vi "S16EPMS.vi"() -> ()   [LabVIEW 2019]
uses:
  sub_vi-s/Global/Global Variables/System Monitor Cluster.ctl
  sub_vi-s/Monitors/Utility/Monitor Communication/Gustav/20TVTI_Cluster.ctl
  sub_vi-s/Monitors/Utility/Monitor Communication/JT/JT-Cluster.ctl
  sub_vi-s/Monitors/Utility/Monitor Communication/S16/VTI-cluster.ctl
  sub_vi-s/Monitors/Utility/Monitor Communication/S16/16T-Cluster.ctl
  sub_vi-s/Monitors/Utility/Monitor Communication/SR830/SR830-Cluster.ctl
  sub_vi-s/Monitors/Utility/Monitor Communication/S16/ILM-Cluster.ctl
  sub_vi-s/Monitors/Utility/Status Monitor/Plot.ctl
  sub_vi-s/Monitors/Utility/Monitor Communication/Gustav/20T_Dewar_Cluster.ctl
  sub_vi-s/Monitors/Utility/Monitor Communication/K6221/K6221_Cluster.ctl
  sub_vi-s/Monitors/Utility/Monitor Communication/PE7265/PE7265-Cluster.ctl
  sub_vi-s/Monitors/Utility/Monitor Communication/PicowattAVS47/PicowattAVS47-Cluster.ctl
  sub_vi-s/Monitors/Utility/Monitor Communication/Mischer/Mischer_Levelmeter-Cluster.ctl
  sub_vi-s/Monitors/Utility/Monitor Communication/Mischer/5T-Cluster.ctl
  sub_vi-s/Monitors/Utility/Monitor Communication/Mischer/Mischer-Cluster.ctl
  sub_vi-s/Monitors/Utility/Monitor Communication/Mischer/VCM-Cluster.ctl
  sub_vi-s/Monitors/Utility/LS372/LS372-Cluster.ctl
  sub_vi-s/Monitors/Utility/Monitor Communication/AMI/AMI_cluster.ctl
  sub_vi-s/Monitors/Utility/Monitor Communication/AMI/AMI_Control.ctl
  sub_vi-s/Monitors/Utility/Monitor Communication/AH2500/AH2500-Cluster.ctl
  sub_vi-s/Monitors/Utility/Monitor Communication/AH2700/AH2700-Cluster.ctl
  sub_vi-s/Monitors/Utility/Monitor Communication/Berta/15T-Cluster.ctl
  sub_vi-s/Monitors/Utility/Monitor Communication/Gustav/20TILM_Cluster.ctl
  sub_vi-s/Monitors/Utility/LS370/Monitor/LS370_only_readout_cluster.ctl
  sub_vi-s/Monitors/Utility/LS372/LS372_read_only-Cluster.ctl
  sub_vi-s/Monitors/Utility/Monitor Communication/LS370/LS370-Control.ctl
  sub_vi-s/Monitors/Utility/ITC503/ITC503Monitor-Cluster.ctl
  sub_vi-s/Monitors/Utility/Monitor Communication/LIA7230/LIA7230-cluster.ctl
  sub_vi-s/Monitors/Utility/Monitor Communication/PPMS/P9_P14_Magnet-cluster.ctl
  sub_vi-s/Monitors/Utility/Monitor Communication/K2812A/K2812A_cluster.ctl
  sub_vi-s/Equipment/Keithley 622x/Configure/2182 -A/Low Level/Typedefs/KE2182 -- Voltage Ranges.ctl
  sub_vi-s/Monitors/Utility/Monitor Communication/Torque_TMC/TMCCluster.ctl
  sub_vi-s/Monitors/Utility/Monitor Communication/PPMS/P9P14-TCluster.ctl
  sub_vi-s/Monitors/Utility/Monitor Communication/zurich_lock_in/zurichinstMonitor.ctl
  sub_vi-s/Monitors/Utility/Monitor Communication/Gustav/20T_Cluster.ctl
  sub_vi-s/Monitors/Utility/Monitor Communication/Kelvinox/Kelvinox_Cluster.ctl
  sub_vi-s/Monitors/Utility/Monitor Communication/SIM921/SIM921_resistance_Bridge_cluster.ctl
  sub_vi-s/Monitors/Utility/Monitor Communication/S16/VTI-control.ctl
  sub_vi-s/Monitors/Utility/Monitor Communication/Gustav/20TVTI_Control.ctl
  sub_vi-s/Monitors/Utility/Monitor Communication/LS372/Ls372-Control.ctl
  sub_vi-s/Global/Global Variables/Data_Display_global.vi
  Instrument_Setup.vi
  sub_vi-s/Global/Global Variables/global.vi
  sub_vi-s/Monitors/Utility/Monitor Communication/sub-vis/ILM_Split_Cluster.vi
  sub_vi-s/Monitors/Utility/Monitor Communication/sub-vis/ILM_Open_Queue.vi
  sub_vi-s/Monitors/Utility/Monitor Communication/sub-vis/ILM_Queue_Commands.vi
  sub_vi-s/Monitors/Utility/Monitor Communication/sub-vis/ILM_Merge_Cluster.vi
  sub_vi-s/Monitors/Utility/Monitor Communication/sub-vis/20T_Open_Queue.vi
  sub_vi-s/Monitors/Utility/Monitor Communication/sub-vis/20T_Split_Cluster.vi
  sub_vi-s/Monitors/Utility/Monitor Communication/sub-vis/20T_Queue_Commands.vi
  sub_vi-s/Monitors/Utility/Monitor Communication/sub-vis/SR830_Open_Queue.vi
  sub_vi-s/Monitors/Utility/Monitor Communication/sub-vis/SR830_Manage_Monitor.vi
  sub_vi-s/Monitors/Utility/Monitor Communication/sub-vis/SR830-2_Open_Queue.vi
  sub_vi-s/Monitors/Utility/Monitor Communication/sub-vis/SR830-3_Open_Queue.vi
  sub_vi-s/Monitors/Utility/Monitor Communication/sub-vis/K6221_Manage_Monitor.vi
  sub_vi-s/Monitors/Utility/Monitor Communication/sub-vis/20TDewar_Open_Queue.vi
  sub_vi-s/Monitors/Utility/Monitor Communication/sub-vis/20TDewar_Manage_Monitor.vi
  sub_vi-s/Monitors/Utility/Monitor Communication/sub-vis/16T_Split_Cluster.vi
  sub_vi-s/Monitors/Utility/Monitor Communication/sub-vis/16T_Open_Queue.vi
  sub_vi-s/Monitors/Utility/Monitor Communication/sub-vis/16T_Queue_Commands.vi
  sub_vi-s/Monitors/Utility/Monitor Communication/sub-vis/16T_Merge_Cluster.vi
  sub_vi-s/Monitors/Utility/Monitor Communication/sub-vis/20T_Merge_Cluster.vi
  sub_vi-s/Monitors/Utility/Monitor Communication/sub-vis/20TVTI_Split_Cluster.vi
  sub_vi-s/Monitors/Utility/Monitor Communication/sub-vis/20TVTI_Open_Queue.vi
  sub_vi-s/Monitors/Utility/Monitor Communication/sub-vis/20TVTI_Queue_Commands.vi
  sub_vi-s/Monitors/Utility/Monitor Communication/sub-vis/20TVTI_Merge_Cluster.vi
  sub_vi-s/Monitors/Utility/Monitor Communication/sub-vis/LS370_Open_Queue.vi
  sub_vi-s/Monitors/Utility/Monitor Communication/sub-vis/JT_Split_Cluster.vi
  sub_vi-s/Monitors/Utility/Monitor Communication/sub-vis/LS370_Queue_Commands.vi
  sub_vi-s/Monitors/Utility/Monitor Communication/sub-vis/JT_Set_Monitor_Values.vi
  sub_vi-s/Monitors/Utility/Monitor Communication/sub-vis/JT_Merge_Cluster.vi
  sub_vi-s/Equipment/Keithley 622x/Keithley 622x.lvlib
panel:
  in  "SIM921":T1
  in  "Kelvinox-Cluster":T2 {"Sorb" format="%_3g"; "MC Heater" format="%#.0f"; "Sorb Heater" format="%#.0f"; "Still Heater" format="%#.0f"; "Rate (K/min)" min=0.0 max=1.0 step=0.001 format="%.3g"; "Setpoint-Manual" min=0.0 max=10.0 step=0.001 format="%.3f"; "T-Setpoint" format="%.3f"; "Sample" format="%_3g"; "4K" format="%_3g"; "MC" format="%_3g"; "Cold\nPlate" format="%_3g"; "1K Pot" format="%_3g"; "Still" format="%_3g"; "P5" format="%_3f"; "P4" format="%_3f"; "P3" format="%_3f"; "P2" format="%_3f"; "P1" format="%_3g"; "Dump" scale=0.0..1000.0}
  in  "20 T Magnet control":T3={"Clamp"=FALSE, "Switch Heater"=FALSE, "Go to Zero"=FALSE, "Go to set"=FALSE, "Go to Hold"=FALSE, "Clamped"=FALSE, "Hold"=FALSE, "Set"=FALSE, "Zero"=FALSE, "Magnet (T)"=0.0, "Leads (T)"=0.0, "Magnet T (K)"=3.4572, "Switch"=FALSE, "Target Field (T)"=3.4572, "Field Setpoint (T)"=0.0, "Rate Setpoint (T/min)"=0.0, "Set Rate"=FALSE, "Rate\n(T/min) "=3.4572, "lambda NV (%)"=3.4572, "lambda p (mbar)"=3.4572, "lambda-Control"=FALSE, "Activate lambda control"=FALSE, "lambda NV  SP"=3.4572, "Set lambda NV"=FALSE, "PSU Status"="", "PSU\nVoltage"=3.4572} {"PSU\nVoltage" format="%.3f"; "lambda NV  SP" format="%.1f"; "lambda p (mbar)" format="%.1f"; "lambda NV (%)" scale=0.0..100.0; "Rate\n(T/min)" format="%.3f"; "Rate Setpoint (T/min)" format="%6.3f"; "Field Setpoint (T)" format="%6.3f"; "Target Field (T)" format="%.3f"; "Magnet T (K)" format="%4.3f"; "Leads (T)" format="%.3f"; "Magnet (T)" format="%.3g"}
  in  "Zurich-Lock-In Monitor":T4
  in  "P9-P14 T-Cluster":T5={"Setpoint"=60.0, "Rate"=10.0, "Chanel 1"=92.8406, "Approach"=0, "Set"=FALSE, "Temperature\nStatus"=6, "Autoshutdown"=FALSE} {"Temperature\nStatus" items=["TemperatureUnknown"=0, "Stable"=1, "Tracking"=2, "Near"=5, "Chasing"=6, "Filling"=7, "Standby"=10, "Disabled"=13, "ImpedanceNotFunction"=14, "TempFailure"=15]; "Approach" items=["Fast Settle", "No O'Shoot"]}
  in  "TMC-Control":T6
  in  "K2182A":T7
  in  "P9/P14-Magnet-Cluster":T9={"Magnet (Oe)"=-0.333, "Setpoint (Oe)"=0.0, "Rate (Oe/min)"=100.0, "Set Field"=FALSE, "Go to zero"=FALSE, "Set Persitant/non-pers"=FALSE, "Approach"=0, "Magnet Status"=1, "Sweeping"=FALSE, "Quenched"=FALSE, "Persitant Mode "=TRUE, "Stable"=FALSE, "Steps"=1.0, "Paused Menu"=0.0, "B Step Start Field"=0.0} {"Magnet Status" items=["MagnetUnknown"=0, "StablePersistent"=1, "WarmingSwitch"=2, "CoolingSwitch"=3, "StableDriven"=4, "Iterating"=5, "Charging"=6, "Discharging"=7, "CurrentError"=8, "MagnetFailure"=15]; "Approach" items=["Linear", "NoOvershoot", "Oscillate"]}
  in  "LIA7230-3":T10={"Lockin 1"=[], "X1-Display"=0.0, "X1 Percent"=0.0, "Y1-Display"=0.0, "X1 Percent 2"=0.0, "Unit X1"="nV", "Unit X2"="nV", "X1 Overload"=FALSE, "Y1 Overload"=FALSE, "Sensitivity Setpoint"=26, "X1"=0.0, "Y1"=0.0, "Channel 3"=0.0, "Channel 4"=0.0, "Channel 4 Percent"=0.0, "Channel 3 Percent "=0.0, "Unit Channel 3"="nV", "Unit Channel 4"="nV", "Overload channel 3"=FALSE, "Overload channel 4"=FALSE, "Offsets (ON)"=FALSE, "Sensitivity Setpoint 2"=26} {"Sensitivity Setpoint 2" items=["2 nV", "5 nV", "10 nV", "20 nV", "50 nV", "100 nV", "200 nV", "500 nV", "1 µV", "2 µV", "5 µV", "10 µV", "20 µV", "50 µV", "100 µV", "200 µV", "500 µV", "1 mV", "2 mV", "5 mV", "10 mV", "20 mV", "50 mV", "100 mV", "200 mV", "500 mV", "1 V", ""]; "Channel 3 Percent" scale=0.0..100.0; "Channel 4 Percent" scale=0.0..100.0; "Sensitivity Setpoint" items=["2 nV", "5 nV", "10 nV", "20 nV", "50 nV", "100 nV", "200 nV", "500 nV", "1 µV", "2 µV", "5 µV", "10 µV", "20 µV", "50 µV", "100 µV", "200 µV", "500 µV", "1 mV", "2 mV", "5 mV", "10 mV", "20 mV", "50 mV", "100 mV", "200 mV", "500 mV", "1 V", ""]; "X1 Percent 2" scale=0.0..100.0; "X1 Percent" scale=0.0..100.0; "X1-Display" format="%#4_5f"}
  in  "LIA7230-2":T10={"Lockin 1"=[[0.0, 0.0, 0.0, 0.0, 0.0, -1e-08, -1e-08, -1e-08, 0.0, 0.0, 0.0, 0.0, 0.0, 0.0, 0.0, 0.0, 0.0, 0.0, 0.0, 0.0, 0.0, 0.0, 0.0, 0.0, 0.0, 0.0, 0.0, 0.0, 0.0, 0.0, 0.0, 0.0, 0.0, 0.0, 0.0, 0.0, 1e-08, 7e-08, 1.3e-07, 1.5e-07, 1.4e-07, 1.4e-07, 1.4e-07, 1.5e-07, 1.7000000000000001e-07, 1.7000000000000001e-07, 1.6e-07, 1.4e-07, 1.2e-07, 1.3e-07, 1.4e-07, 1.5e-07, 1.5e-07, 1.5e-07, 1.5e-07, 1.4e-07, 1.3e-07, 1.3e-07, 1.3e-07, 1.4e-07, 1.5e-07], [0.0, 0.0, 0.0, 0.0, 0.0, 0.0, 0.0, -1e-08, 0.0, 0.0, 0.0, 0.0, 0.0, 0.0, 0.0, 0.0, 0.0, 0.0, 0.0, 0.0, 0.0, 0.0, 0.0, 0.0, 0.0, 0.0, -1e-08, 0.0, 0.0, 0.0, 0.0, 0.0, 0.0, 0.0, 0.0, 0.0, 5.699999999999999e-07, 2.88e-06, 5.84e-06, 6.8e-06, 6.4000000000000006e-06, 6.38e-06, 6.480000000000001e-06, 6.9e-06, 7.8e-06, 8.2e-06, 7.62e-06, 6.59e-06, 5.940000000000001e-06, 6.04e-06, 6.5099999999999995e-06, 6.98e-06, 7.3099999999999995e-06, 7.34e-06, 7.04e-06, 6.730000000000001e-06, 6.570000000000001e-06, 6.24e-06, 6.22e-06, 6.89e-06, 7.42e-06]], "X1-Display"=0.15, "X1 Percent"=0.15, "Y1-Display"=7.42, "X1 Percent 2"=7.42, "Unit X1"="µV", "Unit X2"="µV", "X1 Overload"=FALSE, "Y1 Overload"=FALSE, "Sensitivity Setpoint"=15, "X1"=1.5e-07, "Y1"=7.42e-06, "Channel 3"=7.42, "Channel 4"=88.81, "Channel 4 Percent"=24.669444444444444, "Channel 3 Percent "=7.42, "Unit Channel 3"="µV", "Unit Channel 4"="°", "Overload channel 3"=FALSE, "Overload channel 4"=FALSE, "Offsets (ON)"=FALSE, "Sensitivity Setpoint 2"=15} {"Sensitivity Setpoint 2" items=["2 nV", "5 nV", "10 nV", "20 nV", "50 nV", "100 nV", "200 nV", "500 nV", "1 µV", "2 µV", "5 µV", "10 µV", "20 µV", "50 µV", "100 µV", "200 µV", "500 µV", "1 mV", "2 mV", "5 mV", "10 mV", "20 mV", "50 mV", "100 mV", "200 mV", "500 mV", "1 V", ""]; "Channel 3 Percent" scale=0.0..100.0; "Channel 4 Percent" scale=0.0..100.0; "Sensitivity Setpoint" items=["1 nV", "2 nV", "5 nV", "10 nV", "20 nV", "50 nV", "100 nV", "200 nV", "500 nV", "1 µV", "2 µV", "5 µV", "10 µV", "20 µV", "50 µV", "100 µV", "200 µV", "500 µV", "1 mV", "2 mV", "5 mV", "10 mV", "20 mV", "50 mV", "100 mV", "200 mV", "500 mV", "1 V"]; "X1 Percent 2" scale=0.0..100.0; "X1 Percent" scale=0.0..100.0; "X1-Display" format="%#4_6f"}
  in  "LIA7230-1":T10={"Lockin 1"=[[2e-06, 7e-06, 8.999999999999999e-06, 6e-06, 1e-06, -5e-06, -8.999999999999999e-06, -8.999999999999999e-06, -5e-06, 1e-06, 7e-06, 1e-05, 8.999999999999999e-06, 3e-06, -3e-06, -8e-06, -1e-05, -7e-06, -1e-06, 5e-06, 8.999999999999999e-06, 8e-06, 4e-06, -2e-06, -8e-06, -1e-05, -8e-06, -3e-06, 3e-06, 8e-06, 8.999999999999999e-06, 6e-06, 0.0, -6e-06, -1e-05, -8.999999999999999e-06, -3e-06, 0.0, -2e-06, -1e-06, 3e-06, 1e-06, -5e-06, -1e-05, -1.1e-05, -7e-06, 0.0, 6e-06, 8.999999999999999e-06, 7e-06, 3e-06, -3e-06, -8e-06, -1e-05, -7e-06, -2e-06, 4e-06, 8.999999999999999e-06, 8.999999999999999e-06, 5e-06, -1e-06], [-8.999999999999999e-06, -6e-06, 0.0, 6e-06, 8.999999999999999e-06, 8.999999999999999e-06, 4e-06, -3e-06, -8e-06, -1e-05, -7e-06, -1e-06, 5e-06, 8.999999999999999e-06, 8e-06, 4e-06, -1e-06, -7e-06, -1e-05, -8e-06, -3e-06, 3e-06, 8e-06, 1e-05, 6e-06, 0.0, -6e-06, -1e-05, -1e-05, -5e-06, 1e-06, 7e-06, 1e-05, 8e-06, 2e-06, -4e-06, -1.4e-05, -1.7999999999999997e-05, -6e-06, 2e-06, 5e-06, 8e-06, 8e-06, 4e-06, -3e-06, -8.999999999999999e-06, -1.1e-05, -8e-06, -2e-06, 3e-06, 7e-06, 8e-06, 5e-06, -1e-06, -7e-06, -1e-05, -8e-06, -4e-06, 2e-06, 8e-06, 1e-05]], "X1-Display"=-0.001, "X1 Percent"=0.01, "Y1-Display"=0.01, "X1 Percent 2"=0.1, "Unit X1"="mV", "Unit X2"="mV", "X1 Overload"=FALSE, "Y1 Overload"=FALSE, "Sensitivity Setpoint"=21, "X1"=-1e-06, "Y1"=1e-05, "Channel 3"=0.01, "Channel 4"=95.71, "Channel 4 Percent"=26.58611111111111, "Channel 3 Percent "=0.1, "Unit Channel 3"="mV", "Unit Channel 4"="°", "Overload channel 3"=FALSE, "Overload channel 4"=FALSE, "Offsets (ON)"=FALSE, "Sensitivity Setpoint 2"=21} {"Sensitivity Setpoint 2" items=["2 nV", "5 nV", "10 nV", "20 nV", "50 nV", "100 nV", "200 nV", "500 nV", "1 µV", "2 µV", "5 µV", "10 µV", "20 µV", "50 µV", "100 µV", "200 µV", "500 µV", "1 mV", "2 mV", "5 mV", "10 mV", "20 mV", "50 mV", "100 mV", "200 mV", "500 mV", "1 V", ""]; "Channel 3 Percent" scale=0.0..100.0; "Channel 4 Percent" scale=0.0..100.0; "Sensitivity Setpoint" items=["1 nV", "2 nV", "5 nV", "10 nV", "20 nV", "50 nV", "100 nV", "200 nV", "500 nV", "1 µV", "2 µV", "5 µV", "10 µV", "20 µV", "50 µV", "100 µV", "200 µV", "500 µV", "1 mV", "2 mV", "5 mV", "10 mV", "20 mV", "50 mV", "100 mV", "200 mV", "500 mV", "1 V"]; "X1 Percent 2" scale=0.0..100.0; "X1 Percent" scale=0.0..100.0; "X1-Display" format="%#4_6f"}
  in  "ITC503-Monitor":T11={"Temperatur (K)"=0.0, "Setpoint (K)"=0.0, "Rate (K/min)"=3.4572, "Heater (%)"=0.0, "NV (%)"=0.0, "Heater Manual"=FALSE, "NV Manual"=FALSE, "Go to Set"=FALSE, "Heater SP"=0.0, "Valid?"=FALSE, "Set Heater SP"=FALSE, "Set NV SP"=FALSE, "Heater (%) Display"=3.4572, "NV (%) Display"=3.4572, "NV Setpoint"=0.0, "Change Heater Status"=FALSE, "Change NV Status"=FALSE, "Sample 3"=0.0, "Sample 2"=0.0, "Sweep-State"=FALSE, "Set Auto PID"=FALSE, "Auto PID"=FALSE, "Stopp"=FALSE, "Setpoint-Sweep"=0.0, "Sample 1"=0.0, "Control Channel"=FALSE, "Channel 1"=FALSE, "Channel 2"=FALSE, "Channel 3"=FALSE} {"NV (%) Display" format="%4_5f"; "Heater (%) Display" format="%4_5f"; "NV (%)" scale=0.0..100.0; "Heater (%)" scale=0.0..100.0; "Rate (K/min)" format="%#4_5f"; "Setpoint (K)" format="%6_5f"}
  in  "LS370-Control":T12
  in  "LS372_Readout-Monitor":T13
  in  "LS370_Readout-Monitor":T14
  in  "20TILM":T15 {"Helium" format="%.2f"}
  in  "15T-Cluster":T16={"Magnet (T)"=0.0, "Leads (T)"=0.0, "Setpoint (T)"=3.4572, "Rate (T/min)"=0.0, "Set"=FALSE, "Zero"=FALSE, "Hold"=FALSE, "Go to zero"=FALSE, "Go to Hold"=FALSE, "Go to Set"=FALSE, "Clamp"=FALSE, "Switch Heater"=FALSE, "Rate limit"=FALSE, "Switch"=FALSE, "Clamped"=FALSE, "Persistent"=FALSE, "Quenched"=FALSE, "Sweeping"=FALSE, "Select"=FALSE} {"Rate (T/min)" format="%6_5f"; "Setpoint (T)" format="%6_5f"}
  in  "AH 2700 Monitor":T17={"Units Display"=1, "Sample Switch"=0, "Frequency"=0.0, "V excitation"=0.0, "Capacity Graphic"=[], "Loss Graphic"=[], "Capacity"=0.0, "Loss"=0.0, "Update AH2500"=FALSE, "Bias "=0.0, " AVerage"=0.0} {"V excitation" format="%#_6f"; "Units Display" items=["nanosiemens"=1, "dissipation factor"=2, "kilohms"=3, "gigohms"=4, "loss vector (jpF)"=5]}
  in  "AH2500 Monitor":T18={"Capacity Graphic"=[], "Loss Graphic"=[], "Update AH2500"=FALSE, "Capacity"=0.0, "Loss"=0.0, "AVerage"=enum."5", "ALternate"=enum."1", "BIas"=enum."Disabled", "V excitation"=enum."15.00"}
  out "AMI Status":T19
  in  "AMI_Cluster":T20={"Y Axis Status"=enum."RAMPING", "Z Axis Status"=enum."RAMPING", "Y-Axis (T)"=0.0, "Y-Axis Setpoint (T)"=0.0, "Y-Axis Rate (T/min)"=0.0, "Z-Axis (T)"=0.0, "Z-Axis Setpoint (T)"=0.0, "Z-Axis Rate (T/min)"=0.0, "B AMI rate (T)"=0.0, "AMI Monitor"=FALSE, "AMI Set field rates"=FALSE, "AMI Set field"=FALSE, "Switch Heater Y"=FALSE, "Switch Heater Z"=FALSE, "Switch Heater"=FALSE, "B AMI (T)"=0.0, "B AMI Setpoint (T)"=0.0, "Phi AMI (Deg) "=0.0, "Phi AMI Setpoint (Deg) "=0.0}
  in  "LS372-Cluster":T21={"Activate Tsweep"=FALSE, "Setpoint - Manual"=1.5, "Rate (K/min)"=0.05, "Update Lakeshores"=FALSE, "Still Heater"=FALSE, "Still Power (mW)"=0.0, "Manual Heater"=FALSE, "Manual Heater  (mW) "=0.0, "Heater Range"=0.0, "P (Gain)"=15.0, "I (Reset)"=80.0, "D (Rate)"=0.0, "Heater Power (mW)"=8.96, "MC Thermometer"=1, "MC Temperature"=1.49981, "LS372-T1"=3.18065, "LS372 -T2"=1.49981, "LS372-R1 "=779.91, "LS372-R2"=1745.45, "LS372-T3"=0.0, "LS372-T4"=0.0, "LS372-R3 "=0.0, "LS372-R4 \n\n\n\n"=0.0, "LS372-T5"=0.0, "LS372-T6"=0.0, "LS372-R5"=0.0, "LS372-R6 "=0.0, "Still Power ist"=0.0, "Set Temperatur Sweep main"=FALSE, "Setpoint ist"=1.5, "Disable Heater"=FALSE} {"MC Thermometer" items=["Speer 9905", "ROX U02453"]}
  in  "VCM Monitor":T22={"Steps"=50.0, "Amplitude SET"=1.5, "Frequenz"=19.0, "Amplitude IST"=0.0, "Frequenz IST"=0.0, "A max"=2.0, "iter"=0.0, "Update VCM"=FALSE}
  in  "Mischer Monitor":T23={"G4"=113.66, "G1"=805.0, "P2"=0.14926999999999999, "G3"=75.66, "Flow"=44.93228311689066, "Pot-Preas."=5.14, "IVC"=4.9729999999999996e-08, "G1 [mbar]"=TRUE, "G3 [mbar]"=TRUE, "G4 [mbar]"=TRUE, "IVC [mbar]"=TRUE, "P2 [mbar] "=TRUE, "Flow corrected"=149.3228311689066, "Pot-Pess. Cor"=3.661772246011217, "Pot Temp"=1.4493767123529135, "Pot [mbar]"=TRUE, "Plot"=array6x29267[175602 elements]}
  in  "5 T Cluster":T24={"Go to set"=FALSE, "Go to Zero"=FALSE, "Clamp"=FALSE, "Go to Hold"=FALSE, "Clamped "=FALSE, "Quenched 2"=FALSE, "Rate limit 2"=FALSE, "Magnet (T)"=0.0, "Leads (T)"=0.0, "Rate (T/min)"=0.2, "Sweeping"=FALSE, "Setpoint"=0.0, "Set"=FALSE, "Zero"=TRUE, "Hold"=FALSE, "Clamp"=FALSE} {"Rate (T/min)" format="%6_5f"; "Leads (T)" format="%6_5f"}
  in  "Mischer Levelmeter":T25={"Plot"=array4x25953[103812 elements], "N-Shield (%)"=70.0, "He (%)"=56.71010401793704, "Coldtrap (%)"=90.0, "He - POT (%)"=101.12017967442725, "N-Shield Refill"=FALSE, "Last fill Shield"="13.08.2019    05:51", "Auto Refill Shield"=FALSE, "Trap Refill"=FALSE, "Last fill Coldtrap"="13.08.2019    05:13", "Auto Refill Trap"=FALSE, "Shield Refill"=FALSE, "Coldtrap Refill"=FALSE, "Auto Trap activatet"=TRUE, "Auto Shield Activatet"=TRUE}
  in  "Picowatt AVS47/TS530 Cluster":T26={"Control Channel (K)"=1.4876135922130311, "AVS CH 5 (Res)"=0.0, "AVS CH 6 (Res) "=0.0, "AVS CH 7 (Res) "=0.0, "Control Res."=3914.0, "Auto Excitation"=FALSE, "Auto activatet"=FALSE, "AVS Excitation"=5} caption="Picowatt AVS47/TS530" {"AVS Excitation" items=["no Exc", "3uV", "10uV", "30uV", "100uV", "300uV", "1mV", "3mV"]}
  in  "PE7265-Cluster":T27={"Lockin 1"=[[1.143e-05, 1.14e-05, 1.139e-05, 1.142e-05, 1.142e-05, 1.142e-05, 1.138e-05, 1.133e-05, 1.136e-05, 1.133e-05, 1.124e-05, 1.124e-05, 1.129e-05, 1.132e-05, 1.138e-05, 1.141e-05, 1.132e-05, 1.124e-05, 1.123e-05, 1.125e-05, 1.132e-05, 1.142e-05, 1.142e-05, 1.131e-05, 1.124e-05, 1.126e-05, 1.125e-05, 1.124e-05, 1.131e-05, 1.131e-05, 1.126e-05, 1.126e-05, 1.131e-05, 1.133e-05, 1.131e-05, 1.132e-05, 1.136e-05, 1.135e-05, 1.134e-05, 1.14e-05, 1.14e-05, 1.135e-05, 1.133e-05, 1.133e-05, 1.129e-05, 1.124e-05, 1.131e-05, 1.13e-05, 1.133e-05, 1.137e-05, 1.134e-05, 1.134e-05, 1.134e-05, 1.131e-05, 1.134e-05, 1.138e-05, 1.137e-05, 1.131e-05, 1.13e-05, 1.134e-05, 1.137e-05], [3.5e-07, 3.5e-07, 3.1e-07, 3e-07, 2.8e-07, 2.7e-07, 2.9e-07, 3.2e-07, 3.7e-07, 4.5e-07, 4.3e-07, 3.3e-07, 3e-07, 3.8e-07, 4e-07, 2.9e-07, 2.7e-07, 3.5e-07, 3.9e-07, 3.5e-07, 3e-07, 2.9e-07, 2.9e-07, 2.9e-07, 2.8e-07, 2.9e-07, 3.5e-07, 4.2e-07, 4e-07, 3.5e-07, 3.3e-07, 3e-07, 2.6e-07, 2.2e-07, 2.3e-07, 2.9e-07, 2.8e-07, 1.8e-07, 1.5e-07, 2.3e-07, 3.5e-07, 3.5e-07, 3.3e-07, 3.3e-07, 3.4e-07, 3.6e-07, 3.7e-07, 3.4e-07, 3.1e-07, 2.9e-07, 3e-07, 3.3e-07, 3.4e-07, 3.3e-07, 3.6e-07, 3.6e-07, 3e-07, 2.4e-07, 2.1e-07, 2.6e-07, 3.6e-07]], "X1-Display"=11.37, "X1 Percent"=0.1137, "Y1-Display"=0.36, "X1 Percent 2"=0.0036, "Unit X1"="µV", "Unit X1a"="100 µV", "Unit X2"="µV", "Unit X2a"="100 µV", "X1 Overload"=FALSE, "Y1 Overload"=FALSE, "Sensitivity Setpoint"=14, "X1"=1.137e-05, "Y1"=3.6e-07} {"Sensitivity Setpoint" items=["2 nV", "5 nV", "10 nV", "20 nV", "50 nV", "100 nV", "200 nV", "500 nV", "1 µV", "2 µV", "5 µV", "10 µV", "20 µV", "50 µV", "100 µV", "200 µV", "500 µV", "1 mV", "2 mV", "5 mV", "10 mV", "20 mV", "50 mV", "100 mV", "200 mV", "500 mV", "1 V", ""]; "X1 Percent 2" scale=0.0..1.0; "X1 Percent" scale=0.0..1.0; "X1-Display" format="%#4_5f"}
  in  "Control Temperature":i16(ring)=8 caption="Control Temp" items=["Time", "LI1CH1", "LI1CH2", "LI2CH1", "LI2CH2", "LI3CH1", "LI3CH2", "Field", "N_Level", "H_Level", "Heat_370", "Sorb_Heat", "Still_Heat", "Capacity", "Loss", "Magnet_Temperature", "Lam_Pressure", "Lam_NValve", "370-T1", "370-T2", "370-T3", "370-T4", "370-T5", "370-R1", "370-R2", "370-R3", "370-R4", "370-R5", "372-T1", "372-T2", "372-T3", "372-T4", "372-T5", "372-T6", "372-R1", "372-R2", "372-R3", "372-R4", "372-R5", "372-R6", "Nada", "K2440_Res", "K2440_Current", "VTI_Heater", "VTI_NValve", "LS340_Heater", "K6221_Amplitude", "K6221_Frequency", "Cond_Pressure", "Still_Pressure", "FP_Out_Pressure", "Dump_Pressure", "V1", "V2", "V4", "V5", "V9", "Forepump", "Compressor", "K6221_Offset", "BoxTemp", "By", "Bz", "Phi", "heater-recond (%)", "Dewar Pressure ", "JT-SP-Control", "350 T1", "350 T2", "350 T3", "350 T4", "350 R1", "350 R2", "350 R3", "350 R4", "Angle", "VTI CH1", "VTI CH2", "VTI CH3", "ColdTrap", "Mischer Pot", "G1 (mbar)", "G3 (mbar) ", "G4 (mbar)", "IVC (mbar)", "P2 (mbar) ", "Pot mischer (mbar)", "AVS Control Channel (K)", "AVS Control Channel (RES)", "AVS  Channel 5 (RES) ", "LI3CH3", "LI3CH4", "LI1CH3", "LI1CH4", "LI2CH3", "LI2CH4", "Volt", "Watt", "Torque Angle", "Dewar heater (W)", "PSU Voltage", "Turbopump", "372-R7", "372-T7", "SIM921 Ch1"]
  in  "Main Sample Temperature":i16(ring)=8 caption="Sample Temp" items=["Time", "LI1CH1", "LI1CH2", "LI2CH1", "LI2CH2", "LI3CH1", "LI3CH2", "Field", "N_Level", "H_Level", "Heat_370", "Sorb_Heat", "Still_Heat", "Capacity", "Loss", "Magnet_Temperature", "Lam_Pressure", "Lam_NValve", "370-T1", "370-T2", "370-T3", "370-T4", "370-T5", "370-R1", "370-R2", "370-R3", "370-R4", "370-R5", "372-T1", "372-T2", "372-T3", "372-T4", "372-T5", "372-T6", "372-R1", "372-R2", "372-R3", "372-R4", "372-R5", "372-R6", "Nada", "K2440_Res", "K2440_Current", "VTI_Heater", "VTI_NValve", "LS340_Heater", "K6221_Amplitude", "K6221_Frequency", "Cond_Pressure", "Still_Pressure", "FP_Out_Pressure", "Dump_Pressure", "V1", "V2", "V4", "V5", "V9", "Forepump", "Compressor", "K6221_Offset", "BoxTemp", "By", "Bz", "Phi", "heater-recond (%)", "Dewar Pressure ", "JT-SP-Control", "350 T1", "350 T2", "350 T3", "350 T4", "350 R1", "350 R2", "350 R3", "350 R4", "Angle", "VTI CH1", "VTI CH2", "VTI CH3", "ColdTrap", "Mischer Pot", "G1 (mbar)", "G3 (mbar) ", "G4 (mbar)", "IVC (mbar)", "P2 (mbar) ", "Pot mischer (mbar)", "AVS Control Channel (K)", "AVS Control Channel (RES)", "AVS  Channel 5 (RES) ", "LI3CH3", "LI3CH4", "LI1CH3", "LI1CH4", "LI2CH3", "LI2CH4", "Volt", "Watt", "Torque Angle", "Dewar heater (W)", "PSU Voltage", "Turbopump", "372-R7", "372-T7", "SIM921 Ch1"]
  in  "K6221":T28={"Plot Window"=[], "A"=0.00707, "A (RMS)"=0.004999244934600001, "Hz"=22.08, "I (A)"=0.00707, "f (Hz)"=22.08, "Update"=FALSE, "Offset"=0.0, "Offset (A)"=0.0, "Compliance"=FALSE, "Output"=FALSE, "Output Status"=TRUE}
  out "Data #":dbl=44.0 format="%#_13g"
  out "Runtime":dbl=0.2294750213623047 format="%#_13g"
  in  "SR830-3":T29={"Lockin 1"=[], "X1-Display"=0.0, "Y1-Display"=0.0, "X1 Percent"=0.0, "X1 Overload"=FALSE, "Y1 Overload"=FALSE, "Unit X1"="nV", "Unit X2"="nV", "Unit X2a"="nV", "Unit X1a"="nV", "Sensitivity Setpoint"=26, "X1 Percent 2"=0.0, "Y1"=0.0, "X1"=0.0, "Preamp OVL"=FALSE} {"X1 Percent 2" scale=0.0..1.0; "Sensitivity Setpoint" items=["2 nV", "5 nV", "10 nV", "20 nV", "50 nV", "100 nV", "200 nV", "500 nV", "1 µV", "2 µV", "5 µV", "10 µV", "20 µV", "50 µV", "100 µV", "200 µV", "500 µV", "1 mV", "2 mV", "5 mV", "10 mV", "20 mV", "50 mV", "100 mV", "200 mV", "500 mV", "1 V", ""]; "X1 Percent" scale=0.0..1.0; "X1-Display" format="%#4_5f"}
  in  "20T-Dewar-Cluster":T30={"Dewar Heater (%) Bar"=0.0, "Dewar-Heater (%) Display"=3.4572, "Dewar-Heater (%) SP"=0.0, "Set Dewar-Heater SP"=FALSE, "Change D-Heater Status"=FALSE, "Dewar Pressure"=0.0, "Dewar heater manual"=FALSE, "Dewar Heater (W)"=0.0} {"Dewar Pressure" format="%4.2f"; "Dewar-Heater (%) Display" format="%4.2f"; "Dewar Heater (%) Bar" scale=0.0..100.0}
  in  "Plot 1":T31={"Measurement Graph"=[{"Y"=[3678179998.990376, 3678179999.2392263, 3678180000.2770944, 3678180001.2796392, 3678180002.2735825, 3678180003.27227, 3678180004.282026, 3678180005.268647, 3678180006.267665, 3678180007.2833424, 3678180008.273184, 3678180009.2614937, 3678180010.2721095, 3678180011.2755966, 3678180012.2743664, 3678180013.2815623, 3678180014.4197474, 3678180015.2346487, 3678180016.2441673, 3678180017.2422705, 3678180018.2973943, 3678180019.2844887, 3678180020.2784495, 3678180021.2750273, 3678180022.2797832, 3678180023.298014, 3678180024.271976, 3678180025.279363, 3678180026.2741265, 3678180027.2748265, 3678180028.281594, 3678180029.280332, 3678180030.2687154, 3678180031.2840753, 3678180032.277137, 3678180033.2809224, 3678180034.264525, 3678180035.385113, 3678180036.28983, 3678180037.285784, 3678180038.2776785, 3678180039.2631254, 3678180040.285936, 3678180041.2868166, 3678180042.264264], "X"=[-0.333, -0.333, -0.333, -0.333, -0.333, -0.333, -0.333, -0.333, -0.333, -0.333, -0.333, -0.333, -0.333, -0.333, -0.333, -0.333, -0.333, -0.333, -0.333, -0.333, -0.333, -0.333, -0.333, -0.333, -0.333, -0.333, -0.333, -0.333, -0.333, -0.333, -0.333, -0.333, -0.333, -0.333, -0.333, -0.333, -0.333, -0.333, -0.333, -0.333, -0.333, -0.333, -0.333, -0.333, -0.333]}, {"Y"=[3678179998.990376, 3678179999.2392263, 3678180000.2770944, 3678180001.2796392, 3678180002.2735825, 3678180003.27227, 3678180004.282026, 3678180005.268647, 3678180006.267665, 3678180007.2833424, 3678180008.273184, 3678180009.2614937, 3678180010.2721095, 3678180011.2755966, 3678180012.2743664, 3678180013.2815623, 3678180014.4197474, 3678180015.2346487, 3678180016.2441673, 3678180017.2422705, 3678180018.2973943, 3678180019.2844887, 3678180020.2784495, 3678180021.2750273, 3678180022.2797832, 3678180023.298014, 3678180024.271976, 3678180025.279363, 3678180026.2741265, 3678180027.2748265, 3678180028.281594, 3678180029.280332, 3678180030.2687154, 3678180031.2840753, 3678180032.277137, 3678180033.2809224, 3678180034.264525, 3678180035.385113, 3678180036.28983, 3678180037.285784, 3678180038.2776785, 3678180039.2631254, 3678180040.285936, 3678180041.2868166, 3678180042.264264], "X"=[1.5e-07, 1.5e-07, 1.5e-07, 1.5e-07, 1.5e-07, 1.5e-07, 1.5e-07, 1.5e-07, 1.5e-07, 1.5e-07, 1.5e-07, 1.5e-07, 1.5e-07, 1.5e-07, 1.5e-07, 1.5e-07, 1.5e-07, 1.5e-07, 1.5e-07, 1.5e-07, 1.5e-07, 1.5e-07, 1.5e-07, 1.5e-07, 1.5e-07, 1.5e-07, 1.5e-07, 1.5e-07, 1.5e-07, 1.5e-07, 1.5e-07, 1.5e-07, 1.5e-07, 1.5e-07, 1.5e-07, 1.5e-07, 1.5e-07, 1.5e-07, 1.5e-07, 1.5e-07, 1.5e-07, 1.5e-07, 1.5e-07, 1.5e-07, 1.5e-07]}, {"Y"=[3678179998.990376, 3678179999.2392263, 3678180000.2770944, 3678180001.2796392, 3678180002.2735825, 3678180003.27227, 3678180004.282026, 3678180005.268647, 3678180006.267665, 3678180007.2833424, 3678180008.273184, 3678180009.2614937, 3678180010.2721095, 3678180011.2755966, 3678180012.2743664, 3678180013.2815623, 3678180014.4197474, 3678180015.2346487, 3678180016.2441673, 3678180017.2422705, 3678180018.2973943, 3678180019.2844887, 3678180020.2784495, 3678180021.2750273, 3678180022.2797832, 3678180023.298014, 3678180024.271976, 3678180025.279363, 3678180026.2741265, 3678180027.2748265, 3678180028.281594, 3678180029.280332, 3678180030.2687154, 3678180031.2840753, 3678180032.277137, 3678180033.2809224, 3678180034.264525, 3678180035.385113, 3678180036.28983, 3678180037.285784, 3678180038.2776785, 3678180039.2631254, 3678180040.285936, 3678180041.2868166, 3678180042.264264], "X"=[-1e-06, -1e-06, -1e-06, -1e-06, -1e-06, -1e-06, -1e-06, -1e-06, -1e-06, -1e-06, -1e-06, -1e-06, -1e-06, -1e-06, -1e-06, -1e-06, -1e-06, -1e-06, -1e-06, -1e-06, -1e-06, -1e-06, -1e-06, -1e-06, -1e-06, -1e-06, -1e-06, -1e-06, -1e-06, -1e-06, -1e-06, -1e-06, -1e-06, -1e-06, -1e-06, -1e-06, -1e-06, -1e-06, -1e-06, -1e-06, -1e-06, -1e-06, -1e-06, -1e-06, -1e-06]}, {"Y"=[3678179998.990376, 3678179999.2392263, 3678180000.2770944, 3678180001.2796392, 3678180002.2735825, 3678180003.27227, 3678180004.282026, 3678180005.268647, 3678180006.267665, 3678180007.2833424, 3678180008.273184, 3678180009.2614937, 3678180010.2721095, 3678180011.2755966, 3678180012.2743664, 3678180013.2815623, 3678180014.4197474, 3678180015.2346487, 3678180016.2441673, 3678180017.2422705, 3678180018.2973943, 3678180019.2844887, 3678180020.2784495, 3678180021.2750273, 3678180022.2797832, 3678180023.298014, 3678180024.271976, 3678180025.279363, 3678180026.2741265, 3678180027.2748265, 3678180028.281594, 3678180029.280332, 3678180030.2687154, 3678180031.2840753, 3678180032.277137, 3678180033.2809224, 3678180034.264525, 3678180035.385113, 3678180036.28983, 3678180037.285784, 3678180038.2776785, 3678180039.2631254, 3678180040.285936, 3678180041.2868166, 3678180042.264264], "X"=[-1e-06, -1e-06, -1e-06, -1e-06, -1e-06, -1e-06, -1e-06, -1e-06, -1e-06, -1e-06, -1e-06, -1e-06, -1e-06, -1e-06, -1e-06, -1e-06, -1e-06, -1e-06, -1e-06, -1e-06, -1e-06, -1e-06, -1e-06, -1e-06, -1e-06, -1e-06, -1e-06, -1e-06, -1e-06, -1e-06, -1e-06, -1e-06, -1e-06, -1e-06, -1e-06, -1e-06, -1e-06, -1e-06, -1e-06, -1e-06, -1e-06, -1e-06, -1e-06, -1e-06, -1e-06]}], "X-Axis"=0, "Y-Axis Array"=[1, 1, 3, 7], "Scale Plot"=[], "Rescale X"=FALSE, "Rescale Y"=FALSE} {"Y-Axis Array" items=["Time", "LI1CH1", "LI1CH2", "LI2CH1", "LI2CH2", "LI3CH1", "LI3CH2", "Field", "N_Level", "H_Level", "Heat_370", "Sorb_Heat", "Still_Heat", "Capacity", "Loss", "Magnet_Temperature", "Lam_Pressure", "Lam_NValve", "370-T1", "370-T2", "370-T3", "370-T4", "370-T5", "370-R1", "370-R2", "370-R3", "370-R4", "370-R5", "372-T1", "372-T2", "372-T3", "372-T4", "372-T5", "372-T6", "372-R1", "372-R2", "372-R3", "372-R4", "372-R5", "372-R6", "Nada", "K2440_Res", "K2440_Current", "VTI_Heater", "VTI_NValve", "LS340_Heater", "K6221_Amplitude", "K6221_Frequency", "Cond_Pressure", "Still_Pressure", "FP_Out_Pressure", "Dump_Pressure", "V1", "V2", "V4", "V5", "V9", "Forepump", "Compressor", "K6221_Offset", "BoxTemp", "By", "Bz", "Phi", "heater-recond (%)", "Dewar Pressure ", "JT-SP-Control", "350 T1", "350 T2", "350 T3", "350 T4", "350 R1", "350 R2", "350 R3", "350 R4", "Angle", "VTI CH1", "VTI CH2", "VTI CH3", "ColdTrap", "Mischer Pot", "G1 (mbar)", "G3 (mbar) ", "G4 (mbar)", "IVC (mbar)", "P2 (mbar) ", "Pot mischer (mbar)", "AVS Control Channel (K)", "AVS Control Channel (RES)", "AVS  Channel 5 (RES) ", "LI3CH3", "LI3CH4", "LI1CH3", "LI1CH4", "LI2CH3", "LI2CH4", "Volt", "Watt", "Torque Angle", "Dewar heater (W)", "PSU Voltage", "Turbopump", "372-R7", "372-T7", "SIM921 Ch1"]; "X-Axis" items=["Time", "LI1CH1", "LI1CH2", "LI2CH1", "LI2CH2", "LI3CH1", "LI3CH2", "Field", "N_Level", "H_Level", "Heat_370", "Sorb_Heat", "Still_Heat", "Capacity", "Loss", "Magnet_Temperature", "Lam_Pressure", "Lam_NValve", "370-T1", "370-T2", "370-T3", "370-T4", "370-T5", "370-R1", "370-R2", "370-R3", "370-R4", "370-R5", "372-T1", "372-T2", "372-T3", "372-T4", "372-T5", "372-T6", "372-R1", "372-R2", "372-R3", "372-R4", "372-R5", "372-R6", "Nada", "K2440_Res", "K2440_Current", "VTI_Heater", "VTI_NValve", "LS340_Heater", "K6221_Amplitude", "K6221_Frequency", "Cond_Pressure", "Still_Pressure", "FP_Out_Pressure", "Dump_Pressure", "V1", "V2", "V4", "V5", "V9", "Forepump", "Compressor", "K6221_Offset", "BoxTemp", "By", "Bz", "Phi", "heater-recond (%)", "Dewar Pressure ", "JT-SP-Control", "350 T1", "350 T2", "350 T3", "350 T4", "350 R1", "350 R2", "350 R3", "350 R4", "Angle", "VTI CH1", "VTI CH2", "VTI CH3", "ColdTrap", "Mischer Pot", "G1 (mbar)", "G3 (mbar) ", "G4 (mbar)", "IVC (mbar)", "P2 (mbar) ", "Pot mischer (mbar)", "AVS Control Channel (K)", "AVS Control Channel (RES)", "AVS  Channel 5 (RES) ", "LI3CH3", "LI3CH4", "LI1CH3", "LI1CH4", "LI2CH3", "LI2CH4", "Volt", "Watt", "Torque Angle", "Dewar heater (W)", "PSU Voltage", "Turbopump", "372-R7", "372-T7", "SIM921 Ch1"]}
  in  "Plot 2":T31={"Measurement Graph"=[{"Y"=[3678179998.990376, 3678179999.2392263, 3678180000.2770944, 3678180001.2796392, 3678180002.2735825, 3678180003.27227, 3678180004.282026, 3678180005.268647, 3678180006.267665, 3678180007.2833424, 3678180008.273184, 3678180009.2614937, 3678180010.2721095, 3678180011.2755966, 3678180012.2743664, 3678180013.2815623, 3678180014.4197474, 3678180015.2346487, 3678180016.2441673, 3678180017.2422705, 3678180018.2973943, 3678180019.2844887, 3678180020.2784495, 3678180021.2750273, 3678180022.2797832, 3678180023.298014, 3678180024.271976, 3678180025.279363, 3678180026.2741265, 3678180027.2748265, 3678180028.281594, 3678180029.280332, 3678180030.2687154, 3678180031.2840753, 3678180032.277137, 3678180033.2809224, 3678180034.264525, 3678180035.385113, 3678180036.28983, 3678180037.285784, 3678180038.2776785, 3678180039.2631254, 3678180040.285936, 3678180041.2868166, 3678180042.264264], "X"=[]}, {"Y"=[3678179998.990376, 3678179999.2392263, 3678180000.2770944, 3678180001.2796392, 3678180002.2735825, 3678180003.27227, 3678180004.282026, 3678180005.268647, 3678180006.267665, 3678180007.2833424, 3678180008.273184, 3678180009.2614937, 3678180010.2721095, 3678180011.2755966, 3678180012.2743664, 3678180013.2815623, 3678180014.4197474, 3678180015.2346487, 3678180016.2441673, 3678180017.2422705, 3678180018.2973943, 3678180019.2844887, 3678180020.2784495, 3678180021.2750273, 3678180022.2797832, 3678180023.298014, 3678180024.271976, 3678180025.279363, 3678180026.2741265, 3678180027.2748265, 3678180028.281594, 3678180029.280332, 3678180030.2687154, 3678180031.2840753, 3678180032.277137, 3678180033.2809224, 3678180034.264525, 3678180035.385113, 3678180036.28983, 3678180037.285784, 3678180038.2776785, 3678180039.2631254, 3678180040.285936, 3678180041.2868166, 3678180042.264264], "X"=[1e-05, 1e-05, 1e-05, 1e-05, 1e-05, 1e-05, 1e-05, 1e-05, 1e-05, 1e-05, 1e-05, 1e-05, 1e-05, 1e-05, 1e-05, 1e-05, 1e-05, 1e-05, 1e-05, 1e-05, 1e-05, 1e-05, 1e-05, 1e-05, 1e-05, 1e-05, 1e-05, 1e-05, 1e-05, 1e-05, 1e-05, 1e-05, 1e-05, 1e-05, 1e-05, 1e-05, 1e-05, 1e-05, 1e-05, 1e-05, 1e-05, 1e-05, 1e-05, 1e-05, 1e-05]}, {"Y"=[3678179998.990376, 3678179999.2392263, 3678180000.2770944, 3678180001.2796392, 3678180002.2735825, 3678180003.27227, 3678180004.282026, 3678180005.268647, 3678180006.267665, 3678180007.2833424, 3678180008.273184, 3678180009.2614937, 3678180010.2721095, 3678180011.2755966, 3678180012.2743664, 3678180013.2815623, 3678180014.4197474, 3678180015.2346487, 3678180016.2441673, 3678180017.2422705, 3678180018.2973943, 3678180019.2844887, 3678180020.2784495, 3678180021.2750273, 3678180022.2797832, 3678180023.298014, 3678180024.271976, 3678180025.279363, 3678180026.2741265, 3678180027.2748265, 3678180028.281594, 3678180029.280332, 3678180030.2687154, 3678180031.2840753, 3678180032.277137, 3678180033.2809224, 3678180034.264525, 3678180035.385113, 3678180036.28983, 3678180037.285784, 3678180038.2776785, 3678180039.2631254, 3678180040.285936, 3678180041.2868166, 3678180042.264264], "X"=[-1e-06, -1e-06, -1e-06, -1e-06, -1e-06, -1e-06, -1e-06, -1e-06, -1e-06, -1e-06, -1e-06, -1e-06, -1e-06, -1e-06, -1e-06, -1e-06, -1e-06, -1e-06, -1e-06, -1e-06, -1e-06, -1e-06, -1e-06, -1e-06, -1e-06, -1e-06, -1e-06, -1e-06, -1e-06, -1e-06, -1e-06, -1e-06, -1e-06, -1e-06, -1e-06, -1e-06, -1e-06, -1e-06, -1e-06, -1e-06, -1e-06, -1e-06, -1e-06, -1e-06, -1e-06]}, {"Y"=[3678179998.990376, 3678179999.2392263, 3678180000.2770944, 3678180001.2796392, 3678180002.2735825, 3678180003.27227, 3678180004.282026, 3678180005.268647, 3678180006.267665, 3678180007.2833424, 3678180008.273184, 3678180009.2614937, 3678180010.2721095, 3678180011.2755966, 3678180012.2743664, 3678180013.2815623, 3678180014.4197474, 3678180015.2346487, 3678180016.2441673, 3678180017.2422705, 3678180018.2973943, 3678180019.2844887, 3678180020.2784495, 3678180021.2750273, 3678180022.2797832, 3678180023.298014, 3678180024.271976, 3678180025.279363, 3678180026.2741265, 3678180027.2748265, 3678180028.281594, 3678180029.280332, 3678180030.2687154, 3678180031.2840753, 3678180032.277137, 3678180033.2809224, 3678180034.264525, 3678180035.385113, 3678180036.28983, 3678180037.285784, 3678180038.2776785, 3678180039.2631254, 3678180040.285936, 3678180041.2868166, 3678180042.264264], "X"=[-1e-06, -1e-06, -1e-06, -1e-06, -1e-06, -1e-06, -1e-06, -1e-06, -1e-06, -1e-06, -1e-06, -1e-06, -1e-06, -1e-06, -1e-06, -1e-06, -1e-06, -1e-06, -1e-06, -1e-06, -1e-06, -1e-06, -1e-06, -1e-06, -1e-06, -1e-06, -1e-06, -1e-06, -1e-06, -1e-06, -1e-06, -1e-06, -1e-06, -1e-06, -1e-06, -1e-06, -1e-06, -1e-06, -1e-06, -1e-06, -1e-06, -1e-06, -1e-06, -1e-06, -1e-06]}], "X-Axis"=0, "Y-Axis Array"=[1, 1, 2, 82], "Scale Plot"=[], "Rescale X"=FALSE, "Rescale Y"=FALSE} {"Y-Axis Array" items=["Time", "LI1CH1", "LI1CH2", "LI2CH1", "LI2CH2", "LI3CH1", "LI3CH2", "Field", "N_Level", "H_Level", "Heat_370", "Sorb_Heat", "Still_Heat", "Capacity", "Loss", "Magnet_Temperature", "Lam_Pressure", "Lam_NValve", "370-T1", "370-T2", "370-T3", "370-T4", "370-T5", "370-R1", "370-R2", "370-R3", "370-R4", "370-R5", "372-T1", "372-T2", "372-T3", "372-T4", "372-T5", "372-T6", "372-R1", "372-R2", "372-R3", "372-R4", "372-R5", "372-R6", "Nada", "K2440_Res", "K2440_Current", "VTI_Heater", "VTI_NValve", "LS340_Heater", "K6221_Amplitude", "K6221_Frequency", "Cond_Pressure", "Still_Pressure", "FP_Out_Pressure", "Dump_Pressure", "V1", "V2", "V4", "V5", "V9", "Forepump", "Compressor", "K6221_Offset", "BoxTemp", "By", "Bz", "Phi", "heater-recond (%)", "Dewar Pressure ", "JT-SP-Control", "350 T1", "350 T2", "350 T3", "350 T4", "350 R1", "350 R2", "350 R3", "350 R4", "Angle", "VTI CH1", "VTI CH2", "VTI CH3", "ColdTrap", "Mischer Pot", "G1 (mbar)", "G3 (mbar) ", "G4 (mbar)", "IVC (mbar)", "P2 (mbar) ", "Pot mischer (mbar)", "AVS Control Channel (K)", "AVS Control Channel (RES)", "AVS  Channel 5 (RES) ", "LI3CH3", "LI3CH4", "LI1CH3", "LI1CH4", "LI2CH3", "LI2CH4", "Volt", "Watt", "Torque Angle", "Dewar heater (W)", "PSU Voltage", "Turbopump", "372-R7", "372-T7", "SIM921 Ch1"]; "X-Axis" items=["Time", "LI1CH1", "LI1CH2", "LI2CH1", "LI2CH2", "LI3CH1", "LI3CH2", "Field", "N_Level", "H_Level", "Heat_370", "Sorb_Heat", "Still_Heat", "Capacity", "Loss", "Magnet_Temperature", "Lam_Pressure", "Lam_NValve", "370-T1", "370-T2", "370-T3", "370-T4", "370-T5", "370-R1", "370-R2", "370-R3", "370-R4", "370-R5", "372-T1", "372-T2", "372-T3", "372-T4", "372-T5", "372-T6", "372-R1", "372-R2", "372-R3", "372-R4", "372-R5", "372-R6", "Nada", "K2440_Res", "K2440_Current", "VTI_Heater", "VTI_NValve", "LS340_Heater", "K6221_Amplitude", "K6221_Frequency", "Cond_Pressure", "Still_Pressure", "FP_Out_Pressure", "Dump_Pressure", "V1", "V2", "V4", "V5", "V9", "Forepump", "Compressor", "K6221_Offset", "BoxTemp", "By", "Bz", "Phi", "heater-recond (%)", "Dewar Pressure ", "JT-SP-Control", "350 T1", "350 T2", "350 T3", "350 T4", "350 R1", "350 R2", "350 R3", "350 R4", "Angle", "VTI CH1", "VTI CH2", "VTI CH3", "ColdTrap", "Mischer Pot", "G1 (mbar)", "G3 (mbar) ", "G4 (mbar)", "IVC (mbar)", "P2 (mbar) ", "Pot mischer (mbar)", "AVS Control Channel (K)", "AVS Control Channel (RES)", "AVS  Channel 5 (RES) ", "LI3CH3", "LI3CH4", "LI1CH3", "LI1CH4", "LI2CH3", "LI2CH4", "Volt", "Watt", "Torque Angle", "Dewar heater (W)", "PSU Voltage", "Turbopump", "372-R7", "372-T7", "SIM921 Ch1"]}
  in  "Plot 3":T31 {"Y-Axis Array" items=["Time", "LI1CH1", "LI1CH2", "LI2CH1", "LI2CH2", "LI3CH1", "LI3CH2", "Field", "N_Level", "H_Level", "Heat_370", "Sorb_Heat", "Still_Heat", "Capacity", "Loss", "Magnet_Temperature", "Lam_Pressure", "Lam_NValve", "370-T1", "370-T2", "370-T3", "370-T4", "370-T5", "370-R1", "370-R2", "370-R3", "370-R4", "370-R5", "372-T1", "372-T2", "372-T3", "372-T4", "372-T5", "372-T6", "372-R1", "372-R2", "372-R3", "372-R4", "372-R5", "372-R6", "Nada", "K2440_Res", "K2440_Current", "VTI_Heater", "VTI_NValve", "LS340_Heater", "K6221_Amplitude", "K6221_Frequency", "Cond_Pressure", "Still_Pressure", "FP_Out_Pressure", "Dump_Pressure", "V1", "V2", "V4", "V5", "V9", "Forepump", "Compressor", "K6221_Offset", "BoxTemp", "By", "Bz", "Phi", "heater-recond (%)", "Dewar Pressure ", "JT-SP-Control", "350 T1", "350 T2", "350 T3", "350 T4", "350 R1", "350 R2", "350 R3", "350 R4", "Angle", "VTI CH1", "VTI CH2", "VTI CH3", "ColdTrap", "Mischer Pot", "G1 (mbar)", "G3 (mbar) ", "G4 (mbar)", "IVC (mbar)", "P2 (mbar) ", "Pot mischer (mbar)", "AVS Control Channel (K)", "AVS Control Channel (RES)", "AVS  Channel 5 (RES) ", "LI3CH3", "LI3CH4", "LI1CH3", "LI1CH4", "LI2CH3", "LI2CH4", "Volt", "Watt", "Torque Angle", "Dewar heater (W)", "PSU Voltage", "Turbopump", "372-R7", "372-T7", "SIM921 Ch1"]; "X-Axis" items=["Time", "LI1CH1", "LI1CH2", "LI2CH1", "LI2CH2", "LI3CH1", "LI3CH2", "Field", "N_Level", "H_Level", "Heat_370", "Sorb_Heat", "Still_Heat", "Capacity", "Loss", "Magnet_Temperature", "Lam_Pressure", "Lam_NValve", "370-T1", "370-T2", "370-T3", "370-T4", "370-T5", "370-R1", "370-R2", "370-R3", "370-R4", "370-R5", "372-T1", "372-T2", "372-T3", "372-T4", "372-T5", "372-T6", "372-R1", "372-R2", "372-R3", "372-R4", "372-R5", "372-R6", "Nada", "K2440_Res", "K2440_Current", "VTI_Heater", "VTI_NValve", "LS340_Heater", "K6221_Amplitude", "K6221_Frequency", "Cond_Pressure", "Still_Pressure", "FP_Out_Pressure", "Dump_Pressure", "V1", "V2", "V4", "V5", "V9", "Forepump", "Compressor", "K6221_Offset", "BoxTemp", "By", "Bz", "Phi", "heater-recond (%)", "Dewar Pressure ", "JT-SP-Control", "350 T1", "350 T2", "350 T3", "350 T4", "350 R1", "350 R2", "350 R3", "350 R4", "Angle", "VTI CH1", "VTI CH2", "VTI CH3", "ColdTrap", "Mischer Pot", "G1 (mbar)", "G3 (mbar) ", "G4 (mbar)", "IVC (mbar)", "P2 (mbar) ", "Pot mischer (mbar)", "AVS Control Channel (K)", "AVS Control Channel (RES)", "AVS  Channel 5 (RES) ", "LI3CH3", "LI3CH4", "LI1CH3", "LI1CH4", "LI2CH3", "LI2CH4", "Volt", "Watt", "Torque Angle", "Dewar heater (W)", "PSU Voltage", "Turbopump", "372-R7", "372-T7", "SIM921 Ch1"]}
  in  "20TVTI":T32={"Temperatur (K)"=70.6986, "Setpoint (K)"=0.0, "Rate (K/min)"=3.4572, "Heater (%)"=0.0017142857142857142, "NV (%)"=0.0, "Heater Manual"=TRUE, "NV Manual"=TRUE, "Go to Set"=FALSE, "Pressure"=1.0208606, "Heater SP"=0.0, "Valid?"=FALSE, "Set Heater SP"=FALSE, "Set NV SP"=FALSE, "Heater (%) Display"=0.0, "NV (%) Display"=0.0, "NV Setpoint"=0.0, "Change Heater Status"=FALSE, "Change NV Status"=FALSE, "Change Sweep Type"=FALSE} {"NV (%) Display" format="%4_5f"; "Heater (%) Display" format="%4_5f"; "Heater SP" format="%#4_5f"; "Pressure" format="%#4_5f"; "NV (%)" scale=0.0..100.0; "Heater (%)" scale=0.0..100.0; "Rate (K/min)" format="%#4_5f"; "Setpoint (K)" format="%6_5f"}
  in  "ILM":T33 {"Nitrogen" format="%#4_5f"}
  out "Final rate":dbl format="%#4_5f"
  out "Init rate":dbl format="%#4_5f"
  in  "Panel 6":i16(ring) items=["empty", "SR830-1", "SR830-2", "ILM", "20TILM", "AH2700", "K6221", "Plot3", "20T-Dewar", "SR830-3", "PE7265", "MischerMonitor", "MischerLevelmeter", "LS370 Readout", "LS372 Readout", "LIA7230-1", "LIA7230-2", "LIA7230-3", "K2182A", "TMC Monitor", "zurich_Lock_in", "SIM921"]
  in  "Panel 2":i16(ring) items=["empty", "SR830-1", "SR830-2", "ILM", "20TILM", "AH2700", "K6221", "Plot3", "20T-Dewar", "SR830-3", "PE7265", "MischerMonitor", "MischerLevelmeter", "LS370 Readout", "LS372 Readout", "LIA7230-1", "LIA7230-2", "LIA7230-3", "K2182A", "TMC Monitor", "zurich_Lock_in", "SIM921"]
  in  "Panel 4":i16(ring) items=["empty", "SR830-1", "SR830-2", "ILM", "20TILM", "AH2700", "K6221", "Plot3", "20T-Dewar", "SR830-3", "PE7265", "MischerMonitor", "MischerLevelmeter", "LS370 Readout", "LS372 Readout", "LIA7230-1", "LIA7230-2", "LIA7230-3", "K2182A", "TMC Monitor", "zurich_Lock_in", "SIM921"]
  in  "Panel 5":i16(ring) items=["empty", "SR830-1", "SR830-2", "ILM", "20TILM", "AH2700", "K6221", "Plot3", "20T-Dewar", "SR830-3", "PE7265", "MischerMonitor", "MischerLevelmeter", "LS370 Readout", "LS372 Readout", "LIA7230-1", "LIA7230-2", "LIA7230-3", "K2182A", "TMC Monitor", "zurich_Lock_in", "SIM921"]
  in  "Panel 3":i16(ring)=16 items=["empty", "SR830-1", "SR830-2", "ILM", "20TILM", "AH2700", "K6221", "Plot3", "20T-Dewar", "SR830-3", "PE7265", "MischerMonitor", "MischerLevelmeter", "LS370 Readout", "LS372 Readout", "LIA7230-1", "LIA7230-2", "LIA7230-3", "K2182A", "TMC Monitor", "zurich_Lock_in", "SIM921"]
  in  "Panel 1":i16(ring)=15 items=["empty", "SR830-1", "SR830-2", "ILM", "20TILM", "AH2700", "K6221", "Plot3", "20T-Dewar", "SR830-3", "PE7265", "MischerMonitor", "MischerLevelmeter", "LS370 Readout", "LS372 Readout", "LIA7230-1", "LIA7230-2", "LIA7230-3", "K2182A", "TMC Monitor", "zurich_Lock_in", "SIM921"]
  in  "SR830-2":T29={"Lockin 1"=[], "X1-Display"=0.0, "Y1-Display"=0.0, "X1 Percent"=0.0, "X1 Overload"=FALSE, "Y1 Overload"=FALSE, "Unit X1"="nV", "Unit X2"="nV", "Unit X2a"="nV", "Unit X1a"="nV", "Sensitivity Setpoint"=22, "X1 Percent 2"=0.0, "Y1"=0.0, "X1"=0.0, "Preamp OVL"=FALSE} {"X1 Percent 2" scale=0.0..1.0; "Sensitivity Setpoint" items=["2 nV", "5 nV", "10 nV", "20 nV", "50 nV", "100 nV", "200 nV", "500 nV", "1 µV", "2 µV", "5 µV", "10 µV", "20 µV", "50 µV", "100 µV", "200 µV", "500 µV", "1 mV", "2 mV", "5 mV", "10 mV", "20 mV", "50 mV", "100 mV", "200 mV", "500 mV", "1 V", ""]; "X1 Percent" scale=0.0..1.0; "X1-Display" format="%#_5f"}
  in  "SR830-1":T29={"Lockin 1"=[[1.4931e-05, 1.4931e-05, 1.4931e-05, 1.4931e-05, 1.4931e-05, 1.4931e-05, 1.4931e-05, 1.4931e-05, 1.4931e-05, 1.4931e-05, 1.4931e-05, 1.4931e-05, 1.4931e-05, 1.4931e-05, 1.4931e-05, 1.4931e-05, 1.4931e-05, 1.4931e-05, 1.4931e-05, 1.4931e-05, 1.4931e-05, 1.4931e-05, 1.4931e-05, 1.4931e-05, 1.4931e-05, 1.4931e-05, 1.4931e-05, 1.4931e-05, 1.4931e-05, 1.4931e-05, 1.4931e-05, 1.4931e-05, 1.4931e-05, 1.4931e-05, 1.4931e-05, 1.4931e-05, 1.4931e-05, 1.4931e-05, 1.4931e-05, 1.4931e-05, 1.4931e-05, 1.4931e-05, 1.4931e-05, 1.4931e-05, 1.4931e-05, 1.4931e-05, 1.4931e-05, 1.4931e-05, 1.4931e-05, 1.4931e-05, 1.4931e-05, 1.4931e-05, 1.4931e-05, 1.4931e-05, 1.4931e-05, 1.4931e-05, 1.4931e-05, 1.4931e-05, 1.4931e-05, 1.4931e-05, 1.4931e-05], [2.11598e-06, 2.11598e-06, 2.11598e-06, 2.11598e-06, 2.11598e-06, 2.11598e-06, 2.11598e-06, 2.11598e-06, 2.11598e-06, 2.11598e-06, 2.11598e-06, 2.11598e-06, 2.11598e-06, 2.11598e-06, 2.11598e-06, 2.11598e-06, 2.11598e-06, 2.11598e-06, 2.11598e-06, 2.11598e-06, 2.11598e-06, 2.11598e-06, 2.11598e-06, 2.11598e-06, 2.11598e-06, 2.11598e-06, 2.11598e-06, 2.11598e-06, 2.11598e-06, 2.11598e-06, 2.11598e-06, 2.11598e-06, 2.11598e-06, 2.11598e-06, 2.11598e-06, 2.11598e-06, 2.11598e-06, 2.11598e-06, 2.11598e-06, 2.11598e-06, 2.11598e-06, 2.11598e-06, 2.11598e-06, 2.11598e-06, 2.11598e-06, 2.11598e-06, 2.11598e-06, 2.11598e-06, 2.11598e-06, 2.11598e-06, 2.11598e-06, 2.11598e-06, 2.11598e-06, 2.11598e-06, 2.11598e-06, 2.11598e-06, 2.11598e-06, 2.11598e-06, 2.11598e-06, 2.11598e-06, 2.11598e-06]], "X1-Display"=14.931, "Y1-Display"=2.11598, "X1 Percent"=0.029862, "X1 Overload"=FALSE, "Y1 Overload"=FALSE, "Unit X1"="µV", "Unit X2"="µV", "Unit X2a"="500 µV", "Unit X1a"="500 µV", "Sensitivity Setpoint"=16, "X1 Percent 2"=0.00423196, "Y1"=2.11598e-06, "X1"=1.4931e-05, "Preamp OVL"=FALSE} {"X1 Percent 2" scale=0.0..1.0; "Sensitivity Setpoint" items=["2 nV", "5 nV", "10 nV", "20 nV", "50 nV", "100 nV", "200 nV", "500 nV", "1 µV", "2 µV", "5 µV", "10 µV", "20 µV", "50 µV", "100 µV", "200 µV", "500 µV", "1 mV", "2 mV", "5 mV", "10 mV", "20 mV", "50 mV", "100 mV", "200 mV", "500 mV", "1 V", ""]; "X1 Percent" scale=0.0..1.0; "X1-Display" format="%-#1_5f"}
  in  "16 T Magnet control":T34={"Clamp"=FALSE, "Switch Heater"=FALSE, "Go to Zero"=FALSE, "Go to set"=FALSE, "Go to Hold"=FALSE, "Clamped"=FALSE, "Quenched"=FALSE, "Rate limit"=FALSE, "Persistent"=FALSE, "Hold"=FALSE, "Set"=FALSE, "Zero"=FALSE, "Magnet (T)"=0.0, "Leads (T)"=0.0, "Magnet T (K)"=0.0, "Switch"=FALSE, "Setpoint (T)"=0.0, "Rate (T/min)"=0.001, "Select"=FALSE, "Sweeping"=FALSE} {"Rate (T/min)" format="%#_5f"; "Setpoint (T)" format="%#_5f"; "Magnet T (K)" format="%#4_5f"; "Leads (T)" format="%#_5f"}
  in  "VTI":T35={"Temperatur (K)"=0.0, "Setpoint (K)"=0.0, "Rate (K/min)"=3.4572, "Heater (%)"=0.0, "NV (%)"=0.0, "Heater Manual"=FALSE, "NV Manual"=FALSE, "Go to Set"=FALSE, "Pressure"=0.0, "Heater SP"=0.0, "Valid?"=FALSE, "Set Heater SP"=FALSE, "Set NV SP"=FALSE, "Heater (%) Display"=3.4572, "NV (%) Display"=3.4572, "NV Setpoint"=0.0, "Change Heater Status"=FALSE, "Change NV Status"=FALSE, "Sample 3"=0.0, "Sample 2"=0.0, "Sweep-State"=FALSE, "Set Auto PID"=FALSE, "Auto PID"=FALSE, "Stopp"=FALSE, "Setpoint-Sweep"=0.0} {"NV (%) Display" format="%4_5f"; "Heater (%) Display" format="%4_5f"; "Pressure" format="%#4_5f"; "NV (%)" scale=0.0..100.0; "Heater (%)" scale=0.0..100.0; "Rate (K/min)" format="%#4_5f"; "Setpoint (K)" format="%#_5f"}
  in  "Reset Warning":bool
  in  "JT-Cluster":T36={"Setpoint - Manual"=0.0, "Rate (K/min)"=0.0, "Activate Tsweep"=FALSE, "Disable Heater"=FALSE, "Update Lakeshores"=FALSE, "Still Heater"=FALSE, "Sorb Heater"=FALSE, "Still Power (mW)"=0.0, "Sorb Power (mW)"=0.0, "V2"=FALSE, "V5"=FALSE, "V1"=FALSE, "V9"=FALSE, "F"=FALSE, "C"=FALSE, "V4"=FALSE, "Dump"=0, "P3"=0.0, "P1"=0.0, "P2"=0.0, "P5"=0.0, "Box Temp"=0.0, "Pressure 1"=0, "Pressure 2"=0, "Pressure 3"=15, "Pressure 4"=13, "Setpoint"=0.0, "MC Heater Output"=0.0, "Still Heater Output"=0.0, "Sorb  Heater Output"=0.0, "Heater"=[], "Pressures"=[]} {"Pressure 4" items=["Time", "LI1CH1", "LI1CH2", "LI2CH1", "LI2CH2", "LI3CH1", "LI3CH2", "Field", "Temperature", "Temperature 2", "Temperatrue 3", "Nitrogen_Level", "Helium_Level", "Heater_LS370", "Sorb_Heater", "Still_Heater", "Capacity", "Loss", "Magnet_Temperature", "Lambda_Pressure", "Lambda_Needle_Valve", "LS370-CH1-T", "LS370-CH2-T", "LS370-CH3-T", "LS370-CH4-T", "LS370-TC-T", "LS370-CH1-R", "LS370-CH2-R", "LS370-CH3-R", "LS370-CH4-R", "LS370-TC-R", "LS372-CH1-T", "LS372-CH2-T", "LS372-CH3-T", "LS372-CH4-T", "LS372-CH5-T", "LS372-CH1-R", "LS372-CH2-R", "LS372-CH3-R", "LS372-CH4-R", "LS372-CH5-R", "Nada", "Keithley_Res", "Keithley_Current", "VTI_Heater", "VTI_Needle Valve", "LS340_Heater", "Keithley_6221_Amplitude", "Keithley_6221_Frequency", "Condense_Pressure", "Still_Pressure", "FP_Out_Pressure", "Dump_Pressure", "V1", "V2", "V4", "V5", "V9", "Forepump", "Compressor", "Keihtley_6221_Offset", "BoxTemp", "By", "Bz", "Phi", "heater-recond (%)", "Dewar Pressure "]; "Pressure 3" items=["Time", "LI1CH1", "LI1CH2", "LI2CH1", "LI2CH2", "LI3CH1", "LI3CH2", "Field", "Temperature", "Temperature 2", "Temperatrue 3", "Nitrogen_Level", "Helium_Level", "Heater_LS370", "Sorb_Heater", "Still_Heater", "Capacity", "Loss", "Magnet_Temperature", "Lambda_Pressure", "Lambda_Needle_Valve", "LS370-CH1-T", "LS370-CH2-T", "LS370-CH3-T", "LS370-CH4-T", "LS370-TC-T", "LS370-CH1-R", "LS370-CH2-R", "LS370-CH3-R", "LS370-CH4-R", "LS370-TC-R", "LS372-CH1-T", "LS372-CH2-T", "LS372-CH3-T", "LS372-CH4-T", "LS372-CH5-T", "LS372-CH1-R", "LS372-CH2-R", "LS372-CH3-R", "LS372-CH4-R", "LS372-CH5-R", "Nada", "Keithley_Res", "Keithley_Current", "VTI_Heater", "VTI_Needle Valve", "LS340_Heater", "Keithley_6221_Amplitude", "Keithley_6221_Frequency", "Condense_Pressure", "Still_Pressure", "FP_Out_Pressure", "Dump_Pressure", "V1", "V2", "V4", "V5", "V9", "Forepump", "Compressor", "Keihtley_6221_Offset", "BoxTemp", "By", "Bz", "Phi", "heater-recond (%)", "Dewar Pressure "]; "Pressure 2" items=["Time", "LI1CH1", "LI1CH2", "LI2CH1", "LI2CH2", "LI3CH1", "LI3CH2", "Field", "Temperature", "Temperature 2", "Temperatrue 3", "Nitrogen_Level", "Helium_Level", "Heater_LS370", "Sorb_Heater", "Still_Heater", "Capacity", "Loss", "Magnet_Temperature", "Lambda_Pressure", "Lambda_Needle_Valve", "LS370-CH1-T", "LS370-CH2-T", "LS370-CH3-T", "LS370-CH4-T", "LS370-TC-T", "LS370-CH1-R", "LS370-CH2-R", "LS370-CH3-R", "LS370-CH4-R", "LS370-TC-R", "LS372-CH1-T", "LS372-CH2-T", "LS372-CH3-T", "LS372-CH4-T", "LS372-CH5-T", "LS372-CH1-R", "LS372-CH2-R", "LS372-CH3-R", "LS372-CH4-R", "LS372-CH5-R", "Nada", "Keithley_Res", "Keithley_Current", "VTI_Heater", "VTI_Needle Valve", "LS340_Heater", "Keithley_6221_Amplitude", "Keithley_6221_Frequency", "Condense_Pressure", "Still_Pressure", "FP_Out_Pressure", "Dump_Pressure", "V1", "V2", "V4", "V5", "V9", "Forepump", "Compressor", "Keihtley_6221_Offset", "BoxTemp", "By", "Bz", "Phi", "heater-recond (%)", "Dewar Pressure "]; "Pressure 1" items=["Time", "LI1CH1", "LI1CH2", "LI2CH1", "LI2CH2", "LI3CH1", "LI3CH2", "Field", "Temperature", "Temperature 2", "Temperatrue 3", "Nitrogen_Level", "Helium_Level", "Heater_LS370", "Sorb_Heater", "Still_Heater", "Capacity", "Loss", "Magnet_Temperature", "Lambda_Pressure", "Lambda_Needle_Valve", "LS370-CH1-T", "LS370-CH2-T", "LS370-CH3-T", "LS370-CH4-T", "LS370-TC-T", "LS370-CH1-R", "LS370-CH2-R", "LS370-CH3-R", "LS370-CH4-R", "LS370-TC-R", "LS372-CH1-T", "LS372-CH2-T", "LS372-CH3-T", "LS372-CH4-T", "LS372-CH5-T", "LS372-CH1-R", "LS372-CH2-R", "LS372-CH3-R", "LS372-CH4-R", "LS372-CH5-R", "Nada", "Keithley_Res", "Keithley_Current", "VTI_Heater", "VTI_Needle Valve", "LS340_Heater", "Keithley_6221_Amplitude", "Keithley_6221_Frequency", "Condense_Pressure", "Still_Pressure", "FP_Out_Pressure", "Dump_Pressure", "V1", "V2", "V4", "V5", "V9", "Forepump", "Compressor", "Keihtley_6221_Offset", "BoxTemp", "By", "Bz", "Phi", "heater-recond (%)", "Dewar Pressure "]; "Dump" scale=0.0..540.0}
  in  "Open":bool
  in  "Save":bool
  out "Emergency Stop JT":string
  out "Phi (Deg)":dbl format="%#4_5f"
  out "Step #":dbl format="%#4_5f"
  in  "Truncate Button 2":bool
  in  "Time Stamp":timestamp
  in  "Truncate Button":bool
  in  "Keep every nth":i32=2 min=1 max=10 step=1
  in  "Readout \nMeas (s)":dbl=1.0 format="%#_13g"
  in  "Readout\nMonitor (s)":dbl=1.0 format="%#_13g"
  in  "E-mail of Experiment resposible":string
  out "Warning-Bool":bool
  out "Warning":string
  in  "Temperature 6":i16(ring)=41 items=["Time", "LI1CH1", "LI1CH2", "LI2CH1", "LI2CH2", "LI3CH1", "LI3CH2", "Field", "N_Level", "H_Level", "Heat_370", "Sorb_Heat", "Still_Heat", "Capacity", "Loss", "Magnet_Temperature", "Lam_Pressure", "Lam_NValve", "370-T1", "370-T2", "370-T3", "370-T4", "370-T5", "370-R1", "370-R2", "370-R3", "370-R4", "370-R5", "372-T1", "372-T2", "372-T3", "372-T4", "372-T5", "372-T6", "372-R1", "372-R2", "372-R3", "372-R4", "372-R5", "372-R6", "Nada", "K2440_Res", "K2440_Current", "VTI_Heater", "VTI_NValve", "LS340_Heater", "K6221_Amplitude", "K6221_Frequency", "Cond_Pressure", "Still_Pressure", "FP_Out_Pressure", "Dump_Pressure", "V1", "V2", "V4", "V5", "V9", "Forepump", "Compressor", "K6221_Offset", "BoxTemp", "By", "Bz", "Phi", "heater-recond (%)", "Dewar Pressure ", "JT-SP-Control", "350 T1", "350 T2", "350 T3", "350 T4", "350 R1", "350 R2", "350 R3", "350 R4", "Angle", "VTI CH1", "VTI CH2", "VTI CH3", "ColdTrap", "Mischer Pot", "G1 (mbar)", "G3 (mbar) ", "G4 (mbar)", "IVC (mbar)", "P2 (mbar) ", "Pot mischer (mbar)", "AVS Control Channel (K)", "AVS Control Channel (RES)", "AVS  Channel 5 (RES) ", "LI3CH3", "LI3CH4", "LI1CH3", "LI1CH4", "LI2CH3", "LI2CH4", "Volt", "Watt", "Torque Angle", "Dewar heater (W)", "PSU Voltage", "Turbopump", "372-R7", "372-T7", "SIM921 Ch1"]
  in  "Temperature 5":i16(ring)=41 items=["Time", "LI1CH1", "LI1CH2", "LI2CH1", "LI2CH2", "LI3CH1", "LI3CH2", "Field", "N_Level", "H_Level", "Heat_370", "Sorb_Heat", "Still_Heat", "Capacity", "Loss", "Magnet_Temperature", "Lam_Pressure", "Lam_NValve", "370-T1", "370-T2", "370-T3", "370-T4", "370-T5", "370-R1", "370-R2", "370-R3", "370-R4", "370-R5", "372-T1", "372-T2", "372-T3", "372-T4", "372-T5", "372-T6", "372-R1", "372-R2", "372-R3", "372-R4", "372-R5", "372-R6", "Nada", "K2440_Res", "K2440_Current", "VTI_Heater", "VTI_NValve", "LS340_Heater", "K6221_Amplitude", "K6221_Frequency", "Cond_Pressure", "Still_Pressure", "FP_Out_Pressure", "Dump_Pressure", "V1", "V2", "V4", "V5", "V9", "Forepump", "Compressor", "K6221_Offset", "BoxTemp", "By", "Bz", "Phi", "heater-recond (%)", "Dewar Pressure ", "JT-SP-Control", "350 T1", "350 T2", "350 T3", "350 T4", "350 R1", "350 R2", "350 R3", "350 R4", "Angle", "VTI CH1", "VTI CH2", "VTI CH3", "ColdTrap", "Mischer Pot", "G1 (mbar)", "G3 (mbar) ", "G4 (mbar)", "IVC (mbar)", "P2 (mbar) ", "Pot mischer (mbar)", "AVS Control Channel (K)", "AVS Control Channel (RES)", "AVS  Channel 5 (RES) ", "LI3CH3", "LI3CH4", "LI1CH3", "LI1CH4", "LI2CH3", "LI2CH4", "Volt", "Watt", "Torque Angle", "Dewar heater (W)", "PSU Voltage", "Turbopump", "372-R7", "372-T7", "SIM921 Ch1"]
  in  "Temperature 4":i16(ring)=41 items=["Time", "LI1CH1", "LI1CH2", "LI2CH1", "LI2CH2", "LI3CH1", "LI3CH2", "Field", "N_Level", "H_Level", "Heat_370", "Sorb_Heat", "Still_Heat", "Capacity", "Loss", "Magnet_Temperature", "Lam_Pressure", "Lam_NValve", "370-T1", "370-T2", "370-T3", "370-T4", "370-T5", "370-R1", "370-R2", "370-R3", "370-R4", "370-R5", "372-T1", "372-T2", "372-T3", "372-T4", "372-T5", "372-T6", "372-R1", "372-R2", "372-R3", "372-R4", "372-R5", "372-R6", "Nada", "K2440_Res", "K2440_Current", "VTI_Heater", "VTI_NValve", "LS340_Heater", "K6221_Amplitude", "K6221_Frequency", "Cond_Pressure", "Still_Pressure", "FP_Out_Pressure", "Dump_Pressure", "V1", "V2", "V4", "V5", "V9", "Forepump", "Compressor", "K6221_Offset", "BoxTemp", "By", "Bz", "Phi", "heater-recond (%)", "Dewar Pressure ", "JT-SP-Control", "350 T1", "350 T2", "350 T3", "350 T4", "350 R1", "350 R2", "350 R3", "350 R4", "Angle", "VTI CH1", "VTI CH2", "VTI CH3", "ColdTrap", "Mischer Pot", "G1 (mbar)", "G3 (mbar) ", "G4 (mbar)", "IVC (mbar)", "P2 (mbar) ", "Pot mischer (mbar)", "AVS Control Channel (K)", "AVS Control Channel (RES)", "AVS  Channel 5 (RES) ", "LI3CH3", "LI3CH4", "LI1CH3", "LI1CH4", "LI2CH3", "LI2CH4", "Volt", "Watt", "Torque Angle", "Dewar heater (W)", "PSU Voltage", "Turbopump", "372-R7", "372-T7", "SIM921 Ch1"]
  out "T2-v 2":dbl format="%#4_5f"
  out "T1-v 2":dbl format="%#4_5f"
  out "T3-v 2":dbl format="%#4_5f"
  in  "Temperature 3":i16(ring)=29 items=["Time", "LI1CH1", "LI1CH2", "LI2CH1", "LI2CH2", "LI3CH1", "LI3CH2", "Field", "N_Level", "H_Level", "Heat_370", "Sorb_Heat", "Still_Heat", "Capacity", "Loss", "Magnet_Temperature", "Lam_Pressure", "Lam_NValve", "370-T1", "370-T2", "370-T3", "370-T4", "370-T5", "370-R1", "370-R2", "370-R3", "370-R4", "370-R5", "372-T1", "372-T2", "372-T3", "372-T4", "372-T5", "372-T6", "372-R1", "372-R2", "372-R3", "372-R4", "372-R5", "372-R6", "Nada", "K2440_Res", "K2440_Current", "VTI_Heater", "VTI_NValve", "LS340_Heater", "K6221_Amplitude", "K6221_Frequency", "Cond_Pressure", "Still_Pressure", "FP_Out_Pressure", "Dump_Pressure", "V1", "V2", "V4", "V5", "V9", "Forepump", "Compressor", "K6221_Offset", "BoxTemp", "By", "Bz", "Phi", "heater-recond (%)", "Dewar Pressure ", "JT-SP-Control", "350 T1", "350 T2", "350 T3", "350 T4", "350 R1", "350 R2", "350 R3", "350 R4", "Angle", "VTI CH1", "VTI CH2", "VTI CH3", "ColdTrap", "Mischer Pot", "G1 (mbar)", "G3 (mbar) ", "G4 (mbar)", "IVC (mbar)", "P2 (mbar) ", "Pot mischer (mbar)", "AVS Control Channel (K)", "AVS Control Channel (RES)", "AVS  Channel 5 (RES) ", "LI3CH3", "LI3CH4", "LI1CH3", "LI1CH4", "LI2CH3", "LI2CH4", "Volt", "Watt", "Torque Angle", "Dewar heater (W)", "PSU Voltage", "Turbopump", "372-R7", "372-T7", "SIM921 Ch1"]
  in  "Temperature 2":i16(ring)=9 items=["Time", "LI1CH1", "LI1CH2", "LI2CH1", "LI2CH2", "LI3CH1", "LI3CH2", "Field", "N_Level", "H_Level", "Heat_370", "Sorb_Heat", "Still_Heat", "Capacity", "Loss", "Magnet_Temperature", "Lam_Pressure", "Lam_NValve", "370-T1", "370-T2", "370-T3", "370-T4", "370-T5", "370-R1", "370-R2", "370-R3", "370-R4", "370-R5", "372-T1", "372-T2", "372-T3", "372-T4", "372-T5", "372-T6", "372-R1", "372-R2", "372-R3", "372-R4", "372-R5", "372-R6", "Nada", "K2440_Res", "K2440_Current", "VTI_Heater", "VTI_NValve", "LS340_Heater", "K6221_Amplitude", "K6221_Frequency", "Cond_Pressure", "Still_Pressure", "FP_Out_Pressure", "Dump_Pressure", "V1", "V2", "V4", "V5", "V9", "Forepump", "Compressor", "K6221_Offset", "BoxTemp", "By", "Bz", "Phi", "heater-recond (%)", "Dewar Pressure ", "JT-SP-Control", "350 T1", "350 T2", "350 T3", "350 T4", "350 R1", "350 R2", "350 R3", "350 R4", "Angle", "VTI CH1", "VTI CH2", "VTI CH3", "ColdTrap", "Mischer Pot", "G1 (mbar)", "G3 (mbar) ", "G4 (mbar)", "IVC (mbar)", "P2 (mbar) ", "Pot mischer (mbar)", "AVS Control Channel (K)", "AVS Control Channel (RES)", "AVS  Channel 5 (RES) ", "LI3CH3", "LI3CH4", "LI1CH3", "LI1CH4", "LI2CH3", "LI2CH4", "Volt", "Watt", "Torque Angle", "Dewar heater (W)", "PSU Voltage", "Turbopump", "372-R7", "372-T7", "SIM921 Ch1"]
  in  "Temperature 1":i16(ring)=8 items=["Time", "LI1CH1", "LI1CH2", "LI2CH1", "LI2CH2", "LI3CH1", "LI3CH2", "Field", "N_Level", "H_Level", "Heat_370", "Sorb_Heat", "Still_Heat", "Capacity", "Loss", "Magnet_Temperature", "Lam_Pressure", "Lam_NValve", "370-T1", "370-T2", "370-T3", "370-T4", "370-T5", "370-R1", "370-R2", "370-R3", "370-R4", "370-R5", "372-T1", "372-T2", "372-T3", "372-T4", "372-T5", "372-T6", "372-R1", "372-R2", "372-R3", "372-R4", "372-R5", "372-R6", "Nada", "K2440_Res", "K2440_Current", "VTI_Heater", "VTI_NValve", "LS340_Heater", "K6221_Amplitude", "K6221_Frequency", "Cond_Pressure", "Still_Pressure", "FP_Out_Pressure", "Dump_Pressure", "V1", "V2", "V4", "V5", "V9", "Forepump", "Compressor", "K6221_Offset", "BoxTemp", "By", "Bz", "Phi", "heater-recond (%)", "Dewar Pressure ", "JT-SP-Control", "350 T1", "350 T2", "350 T3", "350 T4", "350 R1", "350 R2", "350 R3", "350 R4", "Angle", "VTI CH1", "VTI CH2", "VTI CH3", "ColdTrap", "Mischer Pot", "G1 (mbar)", "G3 (mbar) ", "G4 (mbar)", "IVC (mbar)", "P2 (mbar) ", "Pot mischer (mbar)", "AVS Control Channel (K)", "AVS Control Channel (RES)", "AVS  Channel 5 (RES) ", "LI3CH3", "LI3CH4", "LI1CH3", "LI1CH4", "LI2CH3", "LI2CH4", "Volt", "Watt", "Torque Angle", "Dewar heater (W)", "PSU Voltage", "Turbopump", "372-R7", "372-T7", "SIM921 Ch1"]
  out "T2-v":dbl format="%#4_5f"
  out "T1-v":dbl format="%#4_5f"
  out "T3-v":dbl format="%#4_5f"
  out "Runstring":string
  out "Runtime":timestamp=timestamp(3678179993.3334064 s since 1904-01-01)
  in  "System Monitor Variables":T37={"Time"=[], "LI1CH1"=[], "LI1CH2"=[], "LI2CH1"=[], "LI2CH2"=[], "LI3CH1"=[], "LI3CH2"=[], "Field"=[], "N_Level"=[], "H_Level"=[], "Heat_370"=[], "Sorb_Heat"=[], "Still_Heat"=[], "Capacity"=[], "Loss"=[], "Magnet_Temperature"=[], "Lam_Pressure"=[], "Lam_NValve"=[], "370-T1"=[], "370-T2"=[], "370-T3"=[], "370-T4"=[], "370-T5"=[], "370-R1"=[], "370-R2"=[], "370-R3"=[], "370-R4"=[], "370-R5"=[], "372-T1"=[], "372-T2"=[], "372-T3"=[], "372-T4"=[], "372-T5"=[], "372-T6"=[], "372-R1"=[], "372-R2"=[], "372-R3"=[], "372-R4"=[], "372-R5"=[], "372-R6"=[], "Nada"=[nan], "K2440_Res"=[], "K2440_Current"=[], "VTI_Heater"=[], "VTI_NValve"=[], "LS340_Heater"=[], "K6221_Amplitude"=[], "K6221_Frequency"=[], "Cond_Pressure"=[], "Still_Pressure"=[], "FP_Out_Pressure"=[], "Dump_Pressure"=[], "V1"=[], "V2"=[], "V4"=[], "V5"=[], "V9"=[], "Forepump"=[], "Compressor"=[], "K6221_Offset"=[], "BoxTemp"=[], "By"=[], "Bz"=[], "Phi"=[], "heater-recond (%)"=[], "Dewar Pressure "=[], "JT-SP-Control"=[], "350 T1"=[], "350 T2"=[], "350 T3"=[], "350 T4"=[], "350 R1"=[], "350 R2"=[], "350 R3"=[], "350 R4"=[], "Angle"=[], "VTI CH1"=[], "VTI CH2"=[], "VTI CH3"=[], "ColdTrap"=[], "Mischer Pot"=[], "G1 (mbar)"=[], "G3 (mbar) "=[], "G4 (mbar)"=[], "IVC (mbar)"=[], "P2 (mbar) "=[], "Pot mischer (mbar)"=[], "AVS Control Channel (K)"=[], "AVS Control Channel (RES)"=[], "AVS  Channel 5 (RES) "=[], "LI3CH3"=[], "LI3CH4"=[], "LI1CH3"=[], "LI1CH4"=[], "LI2CH3"=[], "LI2CH4"=[], "Volt"=[], "Watt"=[], "Torque Angle"=[], "Dewar heater (W)"=[], "PSU Voltage"=[], "Turbopump"=[], "372-R7"=[], "372-T7"=[], "SIM921 Ch1"=[]}
  out "Stop Main":bool
  out "Quench Danger":bool=TRUE
  out "Remaining time of rows":string="Row 18 ends 7/17/2020 5:32:07 PM (00h:54m:50s)\r\nRow 19 ends 7/17/2020 5:39:15 PM (00h:07m:08s)\r\nRow 20 ends 7/17/2020 6:34:05 PM (00h:54m:50s)\r\nRow 21 ends 7/17/2020 8:22:15 PM (01h:48m:09s)\r\nRow 22 ends 7/17/2020 8:29:23 PM (00h:07m:08s)\r\nRow 23 ends 7/17/2020 9:24:13 PM (00h:54m:50s)\r\nRow 24 ends 7/17/2020 9:31:21 PM (00h:07m:08s)\r\nRow 25 ends 7/17/2020 10:26:11 PM (00h:54m:50s)\r\nRow 26 ends 7/18/2020 12:14:21 AM (01h:48m:09s)\r\nRow 27 ends 7/18/2020 12:14:41 AM (00h:00m:20s)\r\n"
  out "Remaining time":string="-00d 00h:00m:48s"
  out "Waiting time":dbl format="%#4_5f"
  out "CC Running time":dbl format="%#4_5f"
  out "Sweep Type":string
  out "Init":dbl format="%#4_5f"
  out "Final":dbl format="%#4_5f"
  out "B (T)":dbl format="%#4_5f"
  out "T (K)":dbl format="%#4_5f"
  out "Row":dbl format="%#4_5f"
  in  "Pause":bool
  in  "Stop":bool
  in  "Start":bool
  out "Current Measurement":string="Stopped"
  out "End of measurement":string="7/21/2020 2:39:53 PM"
  out "Measurement":bool
  in  "Stop Monitor":bool
  # "Lehrstuhl für Topologie korrelierter Systeme"
  # "Sweet 16 enhanced precision measurement software"
  # "Remaining time\nTotal:"
  # "Single rows:"
  # "Measurement ends:"
  # "Current row"
  # "Hz"
  # "Pressures in mbar"
  # "Temperatures in K"
  # "Heater Outputs\nin µW"
  # "DU"
  # "He\nTrap"
  # "LN2\nTrap"
  # "20 T"
  # "K 2182A"
  # "Helium (%)"
  # "Levelmeter"
  # "AMI-Cluster"
  # "2"
  # "to Condenser"
  # "1"
  # "7"
  # "From Still"
  # "5"
  # "Mischer\nEinheit"
  # "12"
  # "Cold\nTrap"
  # "Dump"
  # "9"
  # "8"
  # "K 6221"
  # "SR830-3"
  # "Dewar Pressure\n(mbar)"
  # "Dewar Heater\nPower (%)"
  # "Dewar Heater\nPower (W)"
  # "20T Dewar"
  # "N (%)"
  # "He (%)"
  # "Levelmeter"
  # "SR830-2"
  # "SR830-1"
  # "Dill. unit"
  # "LN2\nTrap"
  # "15"
  # "12"
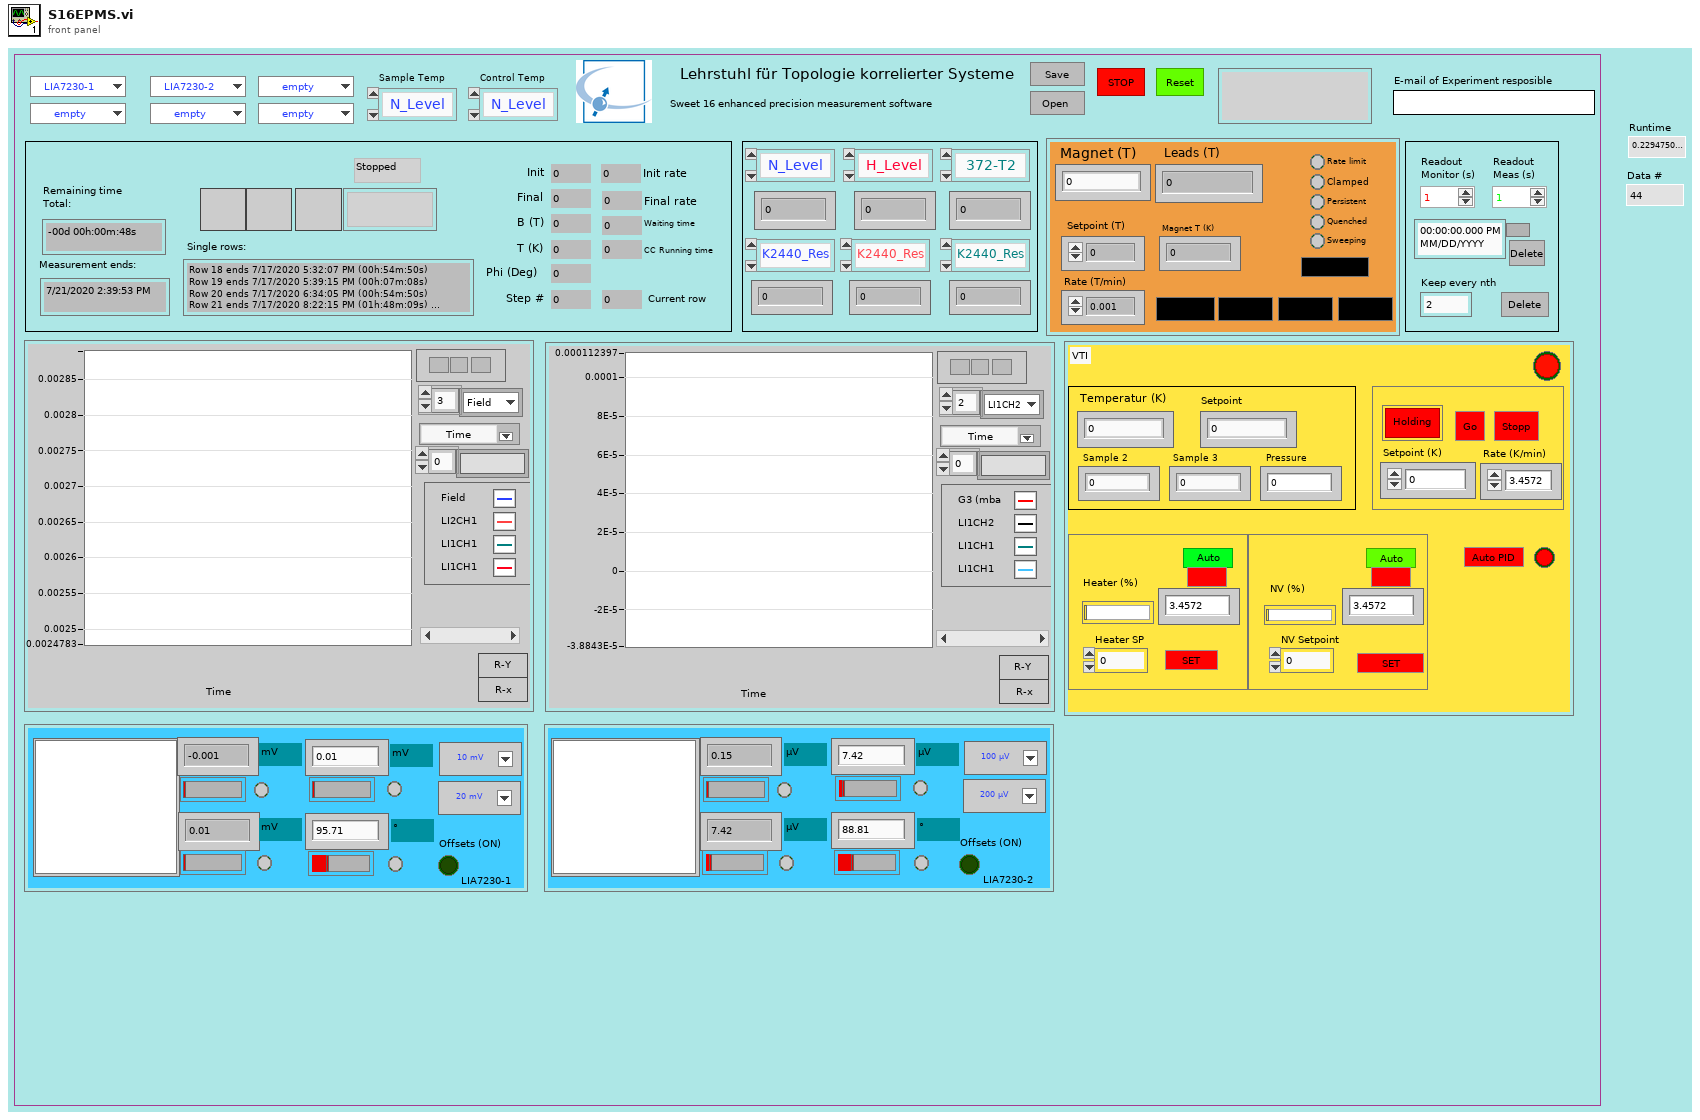
[diagram p1: front panel]
types:
  T1 = typedef "SIM921_resistance_Bridge_cluster.ctl" = cluster{"Resistance Ch1":dbl, "Update":bool}
  T2 = typedef "Kelvinox_Cluster.ctl" = cluster{"V1":bool, "V2":bool, "Dump":u16, "V4":bool, "V5":bool, "V9":bool, "P1":dbl, "P2":dbl, "P3":dbl, "P4":dbl, "P5":dbl, "Turbo":bool, "Forepump":bool, "speed":dbl, "Sorb":dbl, "1K Pot":dbl, "Still":dbl, "Cold\nPlate":dbl, "MC":dbl, "4K":dbl, "Sample":dbl, "T-Setpoint":dbl, "Setpoint-Manual":dbl, "Rate (K/min)":dbl, "Emergency Stop":bool, "Still Heater":dbl, "Sorb Heater":dbl, "T Control active":bool, "MC Heater":dbl, "Sorb Res":dbl, "1K Pot Res":dbl, "Still Res":dbl, "Cold Plate Res":dbl, "MC Res":dbl, "4K Res":dbl, "Sample Res":dbl, "Set Setpoint":bool, "Ramping":bool, "Change T Control Status":bool}
  T3 = typedef "20T_Cluster.ctl" = cluster{"Clamp":bool, "Switch Heater":bool, "Go to Zero":bool, "Go to set":bool, "Go to Hold":bool, "Clamped":bool, "Hold":bool, "Set":bool, "Zero":bool, "Magnet (T)":dbl, "Leads (T)":dbl, "Magnet T (K)":dbl, "Switch":bool, "Target Field (T)":dbl, "Field Setpoint (T)":dbl, "Rate Setpoint (T/min)":dbl, "Set Rate":bool, "Rate\n(T/min) ":dbl, "lambda NV (%)":dbl, "lambda p (mbar)":dbl, "lambda-Control":bool, "Activate lambda control":bool, "lambda NV  SP":dbl, "Set lambda NV":bool, "PSU Status":string, "PSU\nVoltage":dbl}
  T4 = typedef "zurichinstMonitor.ctl" = cluster{"Dmod 1 X":dbl, "Dmod 1 Y":dbl, "Dmod 1 R":dbl, "Dmod 1 Theta":dbl, "Update Oscillators":bool, "Dmod 2 X":dbl, "Dmod 2 R":dbl, "Dmod 2 Y":dbl, "Dmod 2 Theta":dbl}
  T5 = typedef "P9P14-TCluster.ctl" = cluster{"Setpoint":dbl, "Rate":dbl, "Chanel 1":dbl, "Approach":u16, "Set":bool, "Temperature\nStatus":i32, "Autoshutdown":bool}
  T6 = typedef "TMCCluster.ctl" = cluster{"Winkel Setpoint":dbl, "Ausgelesener Winkel":dbl, "Aktuelle Position als 0° Setzen":bool, "Da ist was verkehrt!":bool, "Winkel setzen":bool}
  T7 = typedef "K2812A_cluster.ctl" = cluster{"Plot Window":dbl[][], "Range":dbl, "Update":bool, "Range selector":T8, "Auto Range":bool, "V":dbl, "Auto Range set":bool}
  T8 = typedef "Keithley 622x.lvlib/KE2182 -- Voltage Ranges.ctl" = enum16{"10mV", "100mV", "1V", "10V", "100V"}
  T9 = typedef "P9_P14_Magnet-cluster.ctl" = cluster{"Magnet (Oe)":dbl, "Setpoint (Oe)":dbl, "Rate (Oe/min)":dbl, "Set Field":bool, "Go to zero":bool, "Set Persitant/non-pers":bool, "Approach":i32, "Magnet Status":i32, "Sweeping":bool, "Quenched":bool, "Persitant Mode ":bool, "Stable":bool, "Steps":dbl, "Paused Menu":dbl, "B Step Start Field":dbl}
  T10 = typedef "LIA7230-cluster.ctl" = cluster{"Lockin 1":dbl[][], "X1-Display":dbl, "X1 Percent":dbl, "Y1-Display":dbl, "X1 Percent 2":dbl, "Unit X1":string, "Unit X2":string, "X1 Overload":bool, "Y1 Overload":bool, "Sensitivity Setpoint":i16, "X1":dbl, "Y1":dbl, "Channel 3":dbl, "Channel 4":dbl, "Channel 4 Percent":dbl, "Channel 3 Percent ":dbl, "Unit Channel 3":string, "Unit Channel 4":string, "Overload channel 3":bool, "Overload channel 4":bool, "Offsets (ON)":bool, "Sensitivity Setpoint 2":i16}
  T11 = typedef "ITC503Monitor-Cluster.ctl" = cluster{"Temperatur (K)":dbl, "Setpoint (K)":dbl, "Rate (K/min)":dbl, "Heater (%)":dbl, "NV (%)":dbl, "Heater Manual":bool, "NV Manual":bool, "Go to Set":bool, "Heater SP":dbl, "Valid?":bool, "Set Heater SP":bool, "Set NV SP":bool, "Heater (%) Display":dbl, "NV (%) Display":dbl, "NV Setpoint":dbl, "Change Heater Status":bool, "Change NV Status":bool, "Sample 3":dbl, "Sample 2":dbl, "Sweep-State":bool, "Set Auto PID":bool, "Auto PID":bool, "Stopp":bool, "Setpoint-Sweep":dbl, "Sample 1":dbl, "Control Channel":bool, "Channel 1":bool, "Channel 2":bool, "Channel 3":bool}
  T12 = typedef "LS370-Control.ctl" = cluster{"Disable Heater":bool, "Activate Tsweep":bool, "Update Lakeshores":bool, "Setpoint - Manual":dbl, "Rate (K/min)":dbl, "Sorb Power (mW)":dbl, "Still Power (mW)":dbl, "Sorb Heater":bool, "Still Heater":bool, "Set Temperature Sweep Main":bool}
  T13 = typedef "LS372_read_only-Cluster.ctl" = cluster{"LS372-T1":dbl, "LS372 -T2":dbl, "LS372-T4":dbl, "LS372-T5":dbl, "LS372-T6":dbl, "LS372-R1 ":dbl, "LS372-R2":dbl, "LS372-R3 ":dbl, "LS372-R4 \n\n\n\n":dbl, "LS372-R5":dbl, "LS372-R6 ":dbl, "LS372-T3":dbl, "Update Lakeshores":bool}
  T14 = typedef "LS370_only_readout_cluster.ctl" = cluster{"LS370 T1":dbl, "LS370 T2":dbl, "LS370 T3":dbl, "LS370 T4":dbl, "LS370 T5":dbl, "LS370 R1":dbl, "LS370 R2":dbl, "LS370 R3":dbl, "LS370 R4":dbl, "LS370 R5":dbl, "LS370 T6":dbl, "LS370 T7":dbl, "LS370 T8":dbl, "LS370 T9":dbl, "LS370 R6":dbl, "LS370 R7":dbl, "LS370 R8":dbl, "LS370 R9":dbl, "LS370 TC-T":dbl, "LS370 TC-R":dbl, "Update Lakeshores":bool}
  T15 = typedef "20TILM_Cluster.ctl" = cluster{"Helium":dbl, "Nitrogen":dbl, "Slow":bool, "Fast":bool, "Plot":cluster{"X":dbl, "Y":dbl}[], "Rate":bool}
  T16 = typedef "15T-Cluster.ctl" = cluster{"Magnet (T)":dbl, "Leads (T)":dbl, "Setpoint (T)":dbl, "Rate (T/min)":dbl, "Set":bool, "Zero":bool, "Hold":bool, "Go to zero":bool, "Go to Hold":bool, "Go to Set":bool, "Clamp":bool, "Switch Heater":bool, "Rate limit":bool, "Switch":bool, "Clamped":bool, "Persistent":bool, "Quenched":bool, "Sweeping":bool, "Select":bool}
  T17 = typedef "AH2700-Cluster.ctl" = cluster{"Units Display":i32, "Sample Switch":i32, "Frequency":dbl, "V excitation":dbl, "Capacity Graphic":dbl[][], "Loss Graphic":dbl[][], "Capacity":dbl, "Loss":dbl, "Update AH2500":bool, "Bias ":dbl, " AVerage":dbl}
  T18 = typedef "AH2500-Cluster.ctl" = cluster{"Capacity Graphic":dbl[][], "Loss Graphic":dbl[][], "Update AH2500":bool, "Capacity":dbl, "Loss":dbl, "AVerage":enum16{"0", "1", "2", "3", "4", "5", "6", "7", "8", "9", "10", "11", "12", "13", "14", "15"}, "ALternate":enum16{"0", "1", "2", "3", "4", "5", "6", "7"}, "BIas":enum16{"Disabled", "100 MOhm", "1 MOhm"}, "V excitation":enum16{"15.00", "7.50", "3.75", "3.00", "1.50", "0.750", "0.375", "0.250", "0.125", "0.100", "0.050", "0.030", "0.015", "0.010", "0.0050", "0.0030", "0.0015", "0.0010", "0.0005"}}
  T19 = typedef "AMI_Control.ctl" = cluster{"B AMI rate (T)":dbl, "AMI Set field":bool, "B AMI Setpoint (T)":dbl, "Phi AMI Setpoint (Deg) ":dbl, "Switch Heater":bool, "Y-Axis Setpoint (T)":dbl, "Y-Axis Rate (T/min)":dbl, "Z-Axis Setpoint (T)":dbl, "Z-Axis Rate (T/min)":dbl}
  T20 = typedef "AMI_cluster.ctl" = cluster{"Y Axis Status":enum16{"", "RAMPING", "HOLDING", "PAUSED", "MANUAL UP", "MANUAL DOWN", "ZEROING CURRENT", "QUENCH DETECTED", "HEATING SWITCH", "AT ZER0", "COOLING SWITCH"}, "Z Axis Status":enum16{"", "RAMPING", "HOLDING", "PAUSED", "MANUAL UP", "MANUAL DOWN", "ZEROING CURRENT", "QUENCH DETECTED", "HEATING SWITCH", "AT ZER0", "COOLING SWITCH"}, "Y-Axis (T)":dbl, "Y-Axis Setpoint (T)":dbl, "Y-Axis Rate (T/min)":dbl, "Z-Axis (T)":dbl, "Z-Axis Setpoint (T)":dbl, "Z-Axis Rate (T/min)":dbl, "B AMI rate (T)":dbl, "AMI Monitor":bool, "AMI Set field rates":bool, "AMI Set field":bool, "Switch Heater Y":bool, "Switch Heater Z":bool, "Switch Heater":bool, "B AMI (T)":dbl, "B AMI Setpoint (T)":dbl, "Phi AMI (Deg) ":dbl, "Phi AMI Setpoint (Deg) ":dbl}
  T21 = typedef "LS372-Cluster.ctl" = cluster{"Activate Tsweep":bool, "Setpoint - Manual":dbl, "Rate (K/min)":dbl, "Update Lakeshores":bool, "Still Heater":bool, "Still Power (mW)":dbl, "Manual Heater":bool, "Manual Heater  (mW) ":dbl, "Heater Range":dbl, "P (Gain)":dbl, "I (Reset)":dbl, "D (Rate)":dbl, "Heater Power (mW)":dbl, "MC Thermometer":u16, "MC Temperature":dbl, "LS372-T1":dbl, "LS372 -T2":dbl, "LS372-R1 ":dbl, "LS372-R2":dbl, "LS372-T3":dbl, "LS372-T4":dbl, "LS372-R3 ":dbl, "LS372-R4 \n\n\n\n":dbl, "LS372-T5":dbl, "LS372-T6":dbl, "LS372-R5":dbl, "LS372-R6 ":dbl, "Still Power ist":dbl, "Set Temperatur Sweep main":bool, "Setpoint ist":dbl, "Disable Heater":bool}
  T22 = typedef "VCM-Cluster.ctl" = cluster{"Steps":dbl, "Amplitude SET":dbl, "Frequenz":dbl, "Amplitude IST":dbl, "Frequenz IST":dbl, "A max":dbl, "iter":dbl, "Update VCM":bool}
  T23 = typedef "Mischer-Cluster.ctl" = cluster{"G4":dbl, "G1":dbl, "P2":dbl, "G3":dbl, "Flow":dbl, "Pot-Preas.":dbl, "IVC":dbl, "G1 [mbar]":bool, "G3 [mbar]":bool, "G4 [mbar]":bool, "IVC [mbar]":bool, "P2 [mbar] ":bool, "Flow corrected":dbl, "Pot-Pess. Cor":dbl, "Pot Temp":dbl, "Pot [mbar]":bool, "Plot":dbl[][]}
  T24 = typedef "5T-Cluster.ctl" = cluster{"Go to set":bool, "Go to Zero":bool, "Clamp":bool, "Go to Hold":bool, "Clamped ":bool, "Quenched 2":bool, "Rate limit 2":bool, "Magnet (T)":dbl, "Leads (T)":dbl, "Rate (T/min)":dbl, "Sweeping":bool, "Setpoint":dbl, "Set":bool, "Zero":bool, "Hold":bool, "Clamp":bool}
  T25 = typedef "Mischer_Levelmeter-Cluster.ctl" = cluster{"Plot":dbl[][], "N-Shield (%)":dbl, "He (%)":dbl, "Coldtrap (%)":dbl, "He - POT (%)":dbl, "N-Shield Refill":bool, "Last fill Shield":string, "Auto Refill Shield":bool, "Trap Refill":bool, "Last fill Coldtrap":string, "Auto Refill Trap":bool, "Shield Refill":bool, "Coldtrap Refill":bool, "Auto Trap activatet":bool, "Auto Shield Activatet":bool}
  T26 = typedef "PicowattAVS47-Cluster.ctl" = cluster{"Control Channel (K)":dbl, "AVS CH 5 (Res)":dbl, "AVS CH 6 (Res) ":dbl, "AVS CH 7 (Res) ":dbl, "Control Res.":dbl, "Auto Excitation":bool, "Auto activatet":bool, "AVS Excitation":i16}
  T27 = typedef "PE7265-Cluster.ctl" = cluster{"Lockin 1":dbl[][], "X1-Display":dbl, "X1 Percent":dbl, "Y1-Display":dbl, "X1 Percent 2":dbl, "Unit X1":string, "Unit X1a":string, "Unit X2":string, "Unit X2a":string, "X1 Overload":bool, "Y1 Overload":bool, "Sensitivity Setpoint":i16, "X1":dbl, "Y1":dbl}
  T28 = typedef "K6221_Cluster.ctl" = cluster{"Plot Window":dbl[][], "A":dbl, "A (RMS)":dbl, "Hz":dbl, "I (A)":dbl, "f (Hz)":dbl, "Update":bool, "Offset":dbl, "Offset (A)":dbl, "Compliance":bool, "Output":bool, "Output Status":bool}
  T29 = typedef "SR830-Cluster.ctl" = cluster{"Lockin 1":dbl[][], "X1-Display":dbl, "Y1-Display":dbl, "X1 Percent":dbl, "X1 Overload":bool, "Y1 Overload":bool, "Unit X1":string, "Unit X2":string, "Unit X2a":string, "Unit X1a":string, "Sensitivity Setpoint":i16, "X1 Percent 2":dbl, "Y1":dbl, "X1":dbl, "Preamp OVL":bool}
  T30 = typedef "20T_Dewar_Cluster.ctl" = cluster{"Dewar Heater (%) Bar":dbl, "Dewar-Heater (%) Display":dbl, "Dewar-Heater (%) SP":dbl, "Set Dewar-Heater SP":bool, "Change D-Heater Status":bool, "Dewar Pressure":dbl, "Dewar heater manual":bool, "Dewar Heater (W)":dbl}
  T31 = typedef "Plot.ctl" = cluster{"Measurement Graph":cluster{"Y":dbl[], "X":dbl[]}[], "X-Axis":i16, "Y-Axis Array":i16[], "Scale Plot":string[], "Rescale X":bool, "Rescale Y":bool}
  T32 = typedef "20TVTI_Cluster.ctl" = cluster{"Temperatur (K)":dbl, "Setpoint (K)":dbl, "Rate (K/min)":dbl, "Heater (%)":dbl, "NV (%)":dbl, "Heater Manual":bool, "NV Manual":bool, "Go to Set":bool, "Pressure":dbl, "Heater SP":dbl, "Valid?":bool, "Set Heater SP":bool, "Set NV SP":bool, "Heater (%) Display":dbl, "NV (%) Display":dbl, "NV Setpoint":dbl, "Change Heater Status":bool, "Change NV Status":bool, "Change Sweep Type":bool}
  T33 = typedef "ILM-Cluster.ctl" = cluster{"Plot":dbl[][], "Nitrogen":dbl, "Helium":dbl, "Fast":bool, "Slow":bool, "Rate":bool}
  T34 = typedef "16T-Cluster.ctl" = cluster{"Clamp":bool, "Switch Heater":bool, "Go to Zero":bool, "Go to set":bool, "Go to Hold":bool, "Clamped":bool, "Quenched":bool, "Rate limit":bool, "Persistent":bool, "Hold":bool, "Set":bool, "Zero":bool, "Magnet (T)":dbl, "Leads (T)":dbl, "Magnet T (K)":dbl, "Switch":bool, "Setpoint (T)":dbl, "Rate (T/min)":dbl, "Select":bool, "Sweeping":bool}
  T35 = typedef "VTI-cluster.ctl" = cluster{"Temperatur (K)":dbl, "Setpoint (K)":dbl, "Rate (K/min)":dbl, "Heater (%)":dbl, "NV (%)":dbl, "Heater Manual":bool, "NV Manual":bool, "Go to Set":bool, "Pressure":dbl, "Heater SP":dbl, "Valid?":bool, "Set Heater SP":bool, "Set NV SP":bool, "Heater (%) Display":dbl, "NV (%) Display":dbl, "NV Setpoint":dbl, "Change Heater Status":bool, "Change NV Status":bool, "Sample 3":dbl, "Sample 2":dbl, "Sweep-State":bool, "Set Auto PID":bool, "Auto PID":bool, "Stopp":bool, "Setpoint-Sweep":dbl}
  T36 = typedef "JT-Cluster.ctl" = cluster{"Setpoint - Manual":dbl, "Rate (K/min)":dbl, "Activate Tsweep":bool, "Disable Heater":bool, "Update Lakeshores":bool, "Still Heater":bool, "Sorb Heater":bool, "Still Power (mW)":dbl, "Sorb Power (mW)":dbl, "V2":bool, "V5":bool, "V1":bool, "V9":bool, "F":bool, "C":bool, "V4":bool, "Dump":u8, "P3":dbl, "P1":dbl, "P2":dbl, "P5":dbl, "Box Temp":dbl, "Pressure 1":i16, "Pressure 2":i16, "Pressure 3":i16, "Pressure 4":i16, "Setpoint":dbl, "MC Heater Output":dbl, "Still Heater Output":dbl, "Sorb  Heater Output":dbl, "Heater":dbl[][], "Pressures":dbl[][]}
  T37 = typedef "System Monitor Cluster.ctl" = cluster{"Time":timestamp[], "LI1CH1":dbl[], "LI1CH2":dbl[], "LI2CH1":dbl[], "LI2CH2":dbl[], "LI3CH1":dbl[], "LI3CH2":dbl[], "Field":dbl[], "N_Level":dbl[], "H_Level":dbl[], "Heat_370":dbl[], "Sorb_Heat":dbl[], "Still_Heat":dbl[], "Capacity":dbl[], "Loss":dbl[], "Magnet_Temperature":dbl[], "Lam_Pressure":dbl[], "Lam_NValve":dbl[], "370-T1":dbl[], "370-T2":dbl[], "370-T3":dbl[], "370-T4":dbl[], "370-T5":dbl[], "370-R1":dbl[], "370-R2":dbl[], "370-R3":dbl[], "370-R4":dbl[], "370-R5":dbl[], "372-T1":dbl[], "372-T2":dbl[], "372-T3":dbl[], "372-T4":dbl[], "372-T5":dbl[], "372-T6":dbl[], "372-R1":dbl[], "372-R2":dbl[], "372-R3":dbl[], "372-R4":dbl[], "372-R5":dbl[], "372-R6":dbl[], "Nada":dbl[], "K2440_Res":dbl[], "K2440_Current":dbl[], "VTI_Heater":dbl[], "VTI_NValve":dbl[], "LS340_Heater":dbl[], "K6221_Amplitude":dbl[], "K6221_Frequency":dbl[], "Cond_Pressure":dbl[], "Still_Pressure":dbl[], "FP_Out_Pressure":dbl[], "Dump_Pressure":dbl[], "V1":dbl[], "V2":dbl[], "V4":dbl[], "V5":dbl[], "V9":dbl[], "Forepump":dbl[], "Compressor":dbl[], "K6221_Offset":dbl[], "BoxTemp":dbl[], "By":dbl[], "Bz":dbl[], "Phi":dbl[], "heater-recond (%)":dbl[], "Dewar Pressure ":dbl[], "JT-SP-Control":dbl[], "350 T1":dbl[], "350 T2":dbl[], "350 T3":dbl[], "350 T4":dbl[], "350 R1":dbl[], "350 R2":dbl[], "350 R3":dbl[], "350 R4":dbl[], "Angle":dbl[], "VTI CH1":dbl[], "VTI CH2":dbl[], "VTI CH3":dbl[], "ColdTrap":dbl[], "Mischer Pot":dbl[], "G1 (mbar)":dbl[], "G3 (mbar) ":dbl[], "G4 (mbar)":dbl[], "IVC (mbar)":dbl[], "P2 (mbar) ":dbl[], "Pot mischer (mbar)":dbl[], "AVS Control Channel (K)":dbl[], "AVS Control Channel (RES)":dbl[], "AVS  Channel 5 (RES) ":dbl[], "LI3CH3":dbl[], "LI3CH4":dbl[], "LI1CH3":dbl[], "LI1CH4":dbl[], "LI2CH3":dbl[], "LI2CH4":dbl[], "Volt":dbl[], "Watt":dbl[], "Torque Angle":dbl[], "Dewar heater (W)":dbl[], "PSU Voltage":dbl[], "Turbopump":dbl[], "372-R7":dbl[], "372-T7":dbl[], "SIM921 Ch1":dbl[]}
  T38 = enum16{"open", "replace", "create", "open or create", "replace or create", "replace or create with confirmation"}
  T39 = enum32{"Bad", "Idle", "Run top level", "Running"}
  T40 = enum8{"Enabled", "Disabled", "Disabled and Grayed Out"}
  T41 = typedef "Ls372-Control.ctl" = cluster{"Activate Tsweep":bool, "Setpoint - Manual":dbl, "Rate (K/min)":dbl, "Update Lakeshores":bool, "Still Heater":bool, "Still Power (mW)":dbl, "Manual Heater":bool, "Manual Heater  (mW) ":dbl, "MC Thermometer":u16, "Set Temperature Sweeep main":bool, "Disable Heater":bool}
  T42 = cluster{"AVerage":dbl, "Bias":dbl, "V excitation":dbl, "AH Frequency":dbl}
  T43 = cluster{"LIA7230-Running":bool, "LIA7230-Running 2":bool, "LIA7230-Running 3":bool, "SR830-Running":bool, "SR830-Running 2":bool, "SR830-Running 3":bool, "PE7265-running":bool, "zurich_Lock_in-running":bool}
  T44 = typedef "Mischer_Levelmeter_Status.ctl" = cluster{"Plot":dbl[][], "N-Shield (%)":dbl, "He (%)":dbl, "Coldtrap (%)":dbl, "He - POT (%)":dbl, "Shield Refill":bool, "Coldtrap Refill":bool, "Last fill Shield":string, "Last fill Coldtrap":string, "Auto Shield refill Activatet":bool, "Auto Trap refill activatet":bool}
  T45 = typedef "Mischer_Levelmeter_Control.ctl" = cluster{"N-Shield Refill":bool, "Automatic Refill Shield":bool, "Trap Refill":bool, "Automatic Refill Trap":bool}
  T46 = typedef "Mischer-Control.ctl" = cluster{"G1 [mbar]":bool, "G3 [mbar]":bool, "G4 [mbar]":bool, "IVC [mbar]":bool, "P2 [mbar] ":bool, "Pot [mbar]":bool}
  T47 = typedef "Mischer-Status.ctl" = cluster{"G4":dbl, "G1":dbl, "P2":dbl, "G3":dbl, "Flow":dbl, "Pot-Preas.":dbl, "IVC":dbl, "Flow corrected":dbl, "Pot-Pess. Cor":dbl, "Pot Temp":dbl, "Plot":dbl[][]}
  T48 = typedef "ILM-Control.ctl" = cluster{"Rate":bool}
  T49 = typedef "ILM-Status.ctl" = cluster{"Plot":dbl[][], "Nitrogen":dbl, "Helium":dbl, "Fast":bool, "Slow":bool}
  T50 = typedef "20TILM_Control.ctl" = cluster{"Rate":bool}
  T51 = typedef "20TILM_Status.ctl" = cluster{"Helium":dbl, "Nitrogen":dbl, "Slow":bool, "Fast":bool, "Plot":cluster{"X":dbl, "Y":dbl}[]}
  T52 = typedef "20T_Control.ctl" = cluster{"Clamp":bool, "Switch Heater":bool, "Go to Zero":bool, "Go to Set":bool, "Go to Hold":bool, "Field Setpoint (T)":dbl, "Rate Setpoint (T/min)":dbl, "Set Rate":bool, "Activate lambda control":bool, "Set lambda NV":bool, "lambda NV  SP":dbl}
  T53 = typedef "K2812A_control.ctl" = cluster{"Update":bool, "Range selector":T8, "Auto Range":bool}
  T54 = typedef "K2812A_status.ctl" = cluster{"Plot Window":dbl[][], "Range":dbl, "V":dbl, "Auto Range set":bool}
  T55 = typedef "AH2500-Control.ctl" = cluster{"Update AH2500":bool}
  T56 = typedef "AH2500-Status.ctl" = cluster{"Capacity Graphic":dbl[][], "Loss Graphic":dbl[][], "Capacity":dbl, "Loss":dbl, "AVerage":enum16{"0", "1", "2", "3", "4", "5", "6", "7", "8", "9", "10", "11", "12", "13", "14", "15"}, "ALternate":enum16{"0", "1", "2", "3", "4", "5", "6", "7"}, "BIas":enum16{"Disabled", "100 MOhm", "1 MOhm"}, "V excitation":enum16{"15.00", "7.50", "3.75", "3.00", "1.50", "0.750", "0.375", "0.250", "0.125", "0.100", "0.050", "0.030", "0.015", "0.010", "0.0050", "0.0030", "0.0015", "0.0010", "0.0005"}}
  T57 = typedef "AH2700-Control.ctl" = cluster{"Update AH2500":bool}
  T58 = typedef "AH2700-Status.ctl" = cluster{"Units Display":i32, "Sample Switch":i32, "Frequency":dbl, "V excitation":dbl, "Capacity Graphic":dbl[][], "Loss Graphic":dbl[][], "Capacity":dbl, "Loss":dbl, "Bias ":dbl, " AVerage":dbl}
  T59 = typedef "SIM921_control_cluster.ctl" = cluster{"Update":bool}
  T60 = typedef "SIM921_status_cluster.ctl" = cluster{"Resistance Ch1":dbl}
  T61 = typedef "VCM-Status.ctl" = cluster{"Amplitude IST":dbl, "Frequenz IST":dbl, "iter":dbl}
  T62 = typedef "VCM-Control.ctl" = cluster{"Steps":dbl, "Amplitude SET":dbl, "Frequenz":dbl, "A max":dbl, "Update VCM":bool}
  T63 = typedef "TMC_Status.ctl" = cluster{"Ausgelesener Winkel":dbl, "Da ist was verkehrt!":bool}
  T64 = typedef "TMC_Control.ctl" = cluster{"Winkel Setpoint":dbl, "Aktuelle Position als 0° Setzen":bool, "Winkel setzen":bool}
  T65 = typedef "16T_Control.ctl" = cluster{"Clamp":bool, "Switch Heater":bool, "Go to Zero":bool, "Go to Set":bool, "Go to Hold":bool, "Setpoint (T)":dbl, "Rate (T/min)":dbl, "Set Rate":bool}
  T66 = typedef "16T_Status.ctl" = cluster{"Clamped":bool, "Quenched":bool, "Rate limit":bool, "Persistent":bool, "Hold":bool, "Set":bool, "Zero":bool, "Magnet (T)":dbl, "Leads (T)":dbl, "Magnet T (K)":dbl, "Switch":bool, "Sweeping":bool}
  T67 = typedef "5T_Control.ctl" = cluster{"Rate (T/min)":dbl, "Setpoint":dbl, "Go to set":bool, "Go to Zero":bool, "Clamp":bool, "Go to Hold":bool, "Set Rate":bool}
  T68 = typedef "5T_Status.ctl" = cluster{"Magnet (T)":dbl, "Leads (T)":dbl, "Clamped ":bool, "Quenched 2":bool, "Rate limit 2":bool, "Sweeping":bool, "Set":bool, "Zero":bool, "Hold":bool}
  T69 = typedef "15T-Control.ctl" = cluster{"Setpoint (T)":dbl, "Rate (T/min)":dbl, "Go to zero":bool, "Go to Hold":bool, "Go to Set":bool, "Clamp":bool, "Switch Heater":bool}
  T70 = typedef "15T-Status.ctl" = cluster{"Magnet (T)":dbl, "Leads (T)":dbl, "Set":bool, "Zero":bool, "Hold":bool, "Rate limit":bool, "Switch":bool, "Clamped":bool, "Persistent":bool, "Quenched":bool, "Sweeping":bool, "Select":bool}
  T71 = typedef "AMI_Status.ctl" = cluster{"Y-Axis (T)":dbl, "Z-Axis (T)":dbl, "B AMI (T)":dbl, "Phi AMI (Deg) ":dbl, "Switch Heater Y":bool, "Switch Heater Z":bool, "Y Axis Status":enum16{"", "RAMPING", "HOLDING", "PAUSED", "MANUAL UP", "MANUAL DOWN", "ZEROING CURRENT", "QUENCH DETECTED", "HEATING SWITCH", "AT ZER0", "COOLING SWITCH"}, "Z Axis Status":enum16{"", "RAMPING", "HOLDING", "PAUSED", "MANUAL UP", "MANUAL DOWN", "ZEROING CURRENT", "QUENCH DETECTED", "HEATING SWITCH", "AT ZER0", "COOLING SWITCH"}}
  T72 = typedef "20T_Status.ctl" = cluster{"Clamped":bool, "lambda-Control":bool, "Hold":bool, "Set":bool, "Zero":bool, "Magnet (T)":dbl, "Leads (T)":dbl, "Magnet T (K)":dbl, "Switch":bool, "Target Field (T)":dbl, "Rate (T/min)":dbl, "lambda NV (%)":dbl, "lambda p (mbar)":dbl, "PSU Status":string, "PSU Voltage":dbl}
  T73 = typedef "P9P14_Magnet_Status.ctl" = cluster{"Magnet (Oe)":dbl, "Magnet Status":i32, "Sweeping":bool, "Quenched":bool, "Persitant Mode ":bool, "Stable":bool}
  T74 = typedef "P9P14_Magnet_Control.ctl" = cluster{"Setpoint (Oe)":dbl, "Rate (Oe/min)":dbl, "Set Field":bool, "Go to zero":bool, "Set Persitant/non-pers":bool, "Approach":i32, "Steps":dbl, "Paused Menu":dbl, "B Step start Field":dbl}
  T75 = typedef "VTI-control.ctl" = cluster{"Set VTI SP":bool, "Change NV Status":bool, "Set NV Setpoint":bool, "Change Heater Status":bool, "Set Heater Setpoint":bool, "Setpoint (K)":dbl, "Rate (K/min)":dbl, "Setpoint Heater":dbl, "Setpoint NV":dbl, "Change Auto PID":bool, "Stop Sweep":bool}
  T76 = typedef "VTI-status.ctl" = cluster{"Temperatur (K)":dbl, "Heater (%)":dbl, "NV (%)":dbl, "Heater Manual":bool, "NV Manual":bool, "Pressure":dbl, "Valid?":bool, "Heater (%) Display":dbl, "NV (%) Display":dbl, "Sample 2":dbl, "Sample 3":dbl, "Auto PID":bool, "Sweep-Status":bool, "Setpoint-Sweep":dbl}
  T77 = typedef "20TVTI_Control.ctl" = cluster{"Set VTI SP":bool, "Change NV Status":bool, "Set NV Setpoint":bool, "Change Heater Status":bool, "Set D-Heater Setpoint":bool, "Set Heater Setpoint":bool, "Change D-Heater Status":bool, "Set Sweep Type":bool, "Setpoint (K)":dbl, "Rate (K/min)":dbl, "Setpoint Heater":dbl, "Setpoint D-Heater":dbl, "Setpoint NV":dbl}
  T78 = typedef "20TVTI_Status.ctl" = cluster{"Temperatur (K)":dbl, "Heater (%)":dbl, "NV (%)":dbl, "Heater Manual":bool, "NV Manual":bool, "Pressure":dbl, "Dewar Pressure":dbl, "Valid?":bool, "Dewar Heater Manual":bool, "Heater (%) Display":dbl, "NV (%) Display":dbl, "Dewar Heater (%)":dbl, "D-Heater (%) Display":dbl}
  T79 = typedef "JT-Status.ctl" = cluster{"V2":bool, "V5":bool, "V1":bool, "V9":bool, "F":bool, "C":bool, "V4":bool, "Dump":u8, "P3":dbl, "P1":dbl, "P2":dbl, "P5":dbl, "Box Temp":dbl, "Pressure 1":i16, "Pressure 2":i16, "Pressure 3":i16, "Pressure 4":i16, "Setpoint":dbl, "MC Heater Output":dbl, "Still Heater Output":dbl, "Sorb  Heater Output":dbl, "Heater":dbl[][], "Pressures":dbl[][]}
  T80 = typedef "Kelvinox_Status.ctl" = cluster{"V1":bool, "V2":bool, "Dump":u16, "V4":bool, "V5":bool, "V9":bool, "P1":dbl, "P2":dbl, "P3":dbl, "P4":dbl, "P5":dbl, "Turbo":bool, "Forepump":bool, "speed":dbl, "Sorb":dbl, "1K Pot":dbl, "Still":dbl, "Cold\nPlate":dbl, "MC":dbl, "4K":dbl, "Sample":dbl, "T-Setpoint":dbl, "MC Heater":dbl, "Still Heater":dbl, "Sorb Heater":dbl, "T Control active":bool, "Sorb Res":dbl, "1K Pot Res":dbl, "Still Res":dbl, "Cold Plate Res":dbl, "MC Res":dbl, "4K Res":dbl, "Sample Res":dbl, "Ramping":bool}
  T81 = typedef "Kelvinox_Control.ctl" = cluster{"T-Setpoint-Manual":dbl, "Rate (K/min)":dbl, "Change T Control Status":bool, "Emergency Stop":bool, "Set Setpoint":bool}
  T82 = typedef "LS370_read_only_control.ctl" = cluster{"Update Lakeshores":bool}
  T83 = typedef "LS370_read_only_status.ctl" = cluster{"LS370 T1":dbl, "LS370 T2":dbl, "LS370 T3":dbl, "LS370 T4":dbl, "LS370 T5":dbl, "LS370 R1":dbl, "LS370 R2":dbl, "LS370 R3":dbl, "LS370 R4":dbl, "LS370 R5":dbl, "LS370 T6":dbl, "LS370 T7":dbl, "LS370 T8":dbl, "LS370 T9":dbl, "LS370 R6":dbl, "LS370 R7":dbl, "LS370 R8":dbl, "LS370 R9":dbl, "LS370 TC-T":dbl, "LS370 TC-R":dbl}
  T84 = typedef "LS372_read_only-Control.ctl" = cluster{"Update Lakeshores":bool}
  T85 = typedef "LS372_read_only-Status.ctl" = cluster{"LS372-T1":dbl, "LS372 -T2":dbl, "LS372-T4":dbl, "LS372-T5":dbl, "LS372-T6":dbl, "LS372-R1 ":dbl, "LS372-R2":dbl, "LS372-R3 ":dbl, "LS372-R4 \n\n\n\n":dbl, "LS372-R5":dbl, "LS372-R6 ":dbl, "LS372-T3":dbl}
  T86 = typedef "LS372-Status.ctl" = cluster{"Heater Range":dbl, "P (Gain)":dbl, "I (Reset)":dbl, "D (Rate)":dbl, "Heater Power (mW)":dbl, "MC Temperature":dbl, "LS372-T1":dbl, "LS372 -T2":dbl, "LS372-R1 ":dbl, "LS372-R2":dbl, "LS372-T3":dbl, "LS372-T4":dbl, "LS372-R3 ":dbl, "LS372-R4 \n\n\n\n":dbl, "LS372-T5":dbl, "LS372-T6":dbl, "LS372-R5":dbl, "LS372-R6 ":dbl, "Still Power ist":dbl, "Setpoint ist":dbl}
  T87 = typedef "ITC503_control.ctl" = cluster{"Setpoint (K)":dbl, "Rate (K/min)":dbl, "Go to Set":bool, "Set Heater SP":bool, "Set NV SP":bool, "Change Heater Status":bool, "Change NV Status":bool, "Set Auto PID":bool, "Stopp":bool, "Control Channel":bool, "Heater SP":dbl, "NV Setpoint":dbl}
  T88 = typedef "ITC503_Status.ctl" = cluster{"Temperatur (K)":dbl, "Heater (%)":dbl, "NV (%)":dbl, "Heater Manual":bool, "NV Manual":bool, "Valid?":bool, "Heater (%) Display":dbl, "NV (%) Display":dbl, "Sample 3":dbl, "Sample 2":dbl, "Sweep-State":bool, "Auto PID":bool, "Setpoint-Sweep":dbl, "Sample 1":dbl, "Channel 1":bool, "Channel 2":bool, "Channel 3":bool}
  T89 = typedef "P9P14-TCluster-Status.ctl" = cluster{"Chanel 1":dbl, "Temperature\nStatus":i32}
  T90 = typedef "P9P14-TCluster-Control.ctl" = cluster{"Setpoint":dbl, "Rate":dbl, "Approach":u16, "Set":bool, "Autoshutdown":bool}
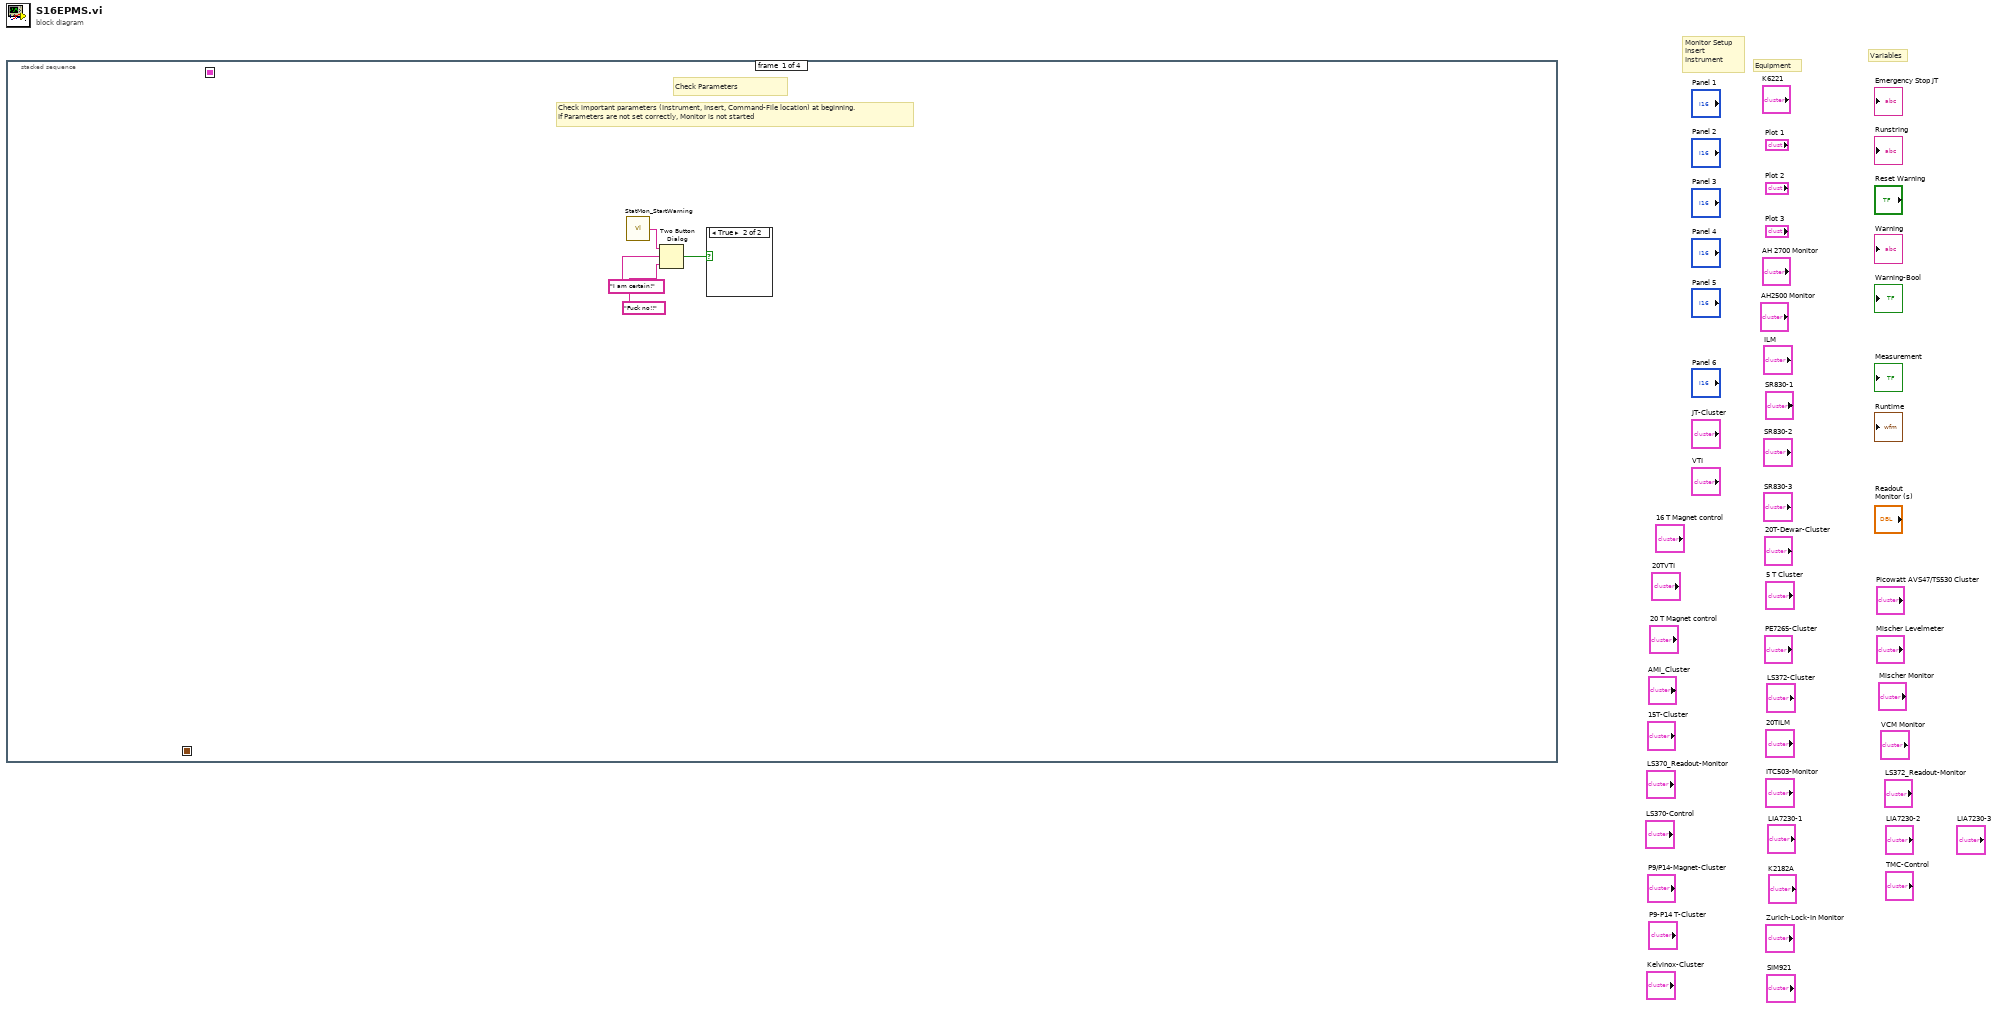
[diagram p0: block diagram]
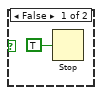
[diagram p2: hidden frame]
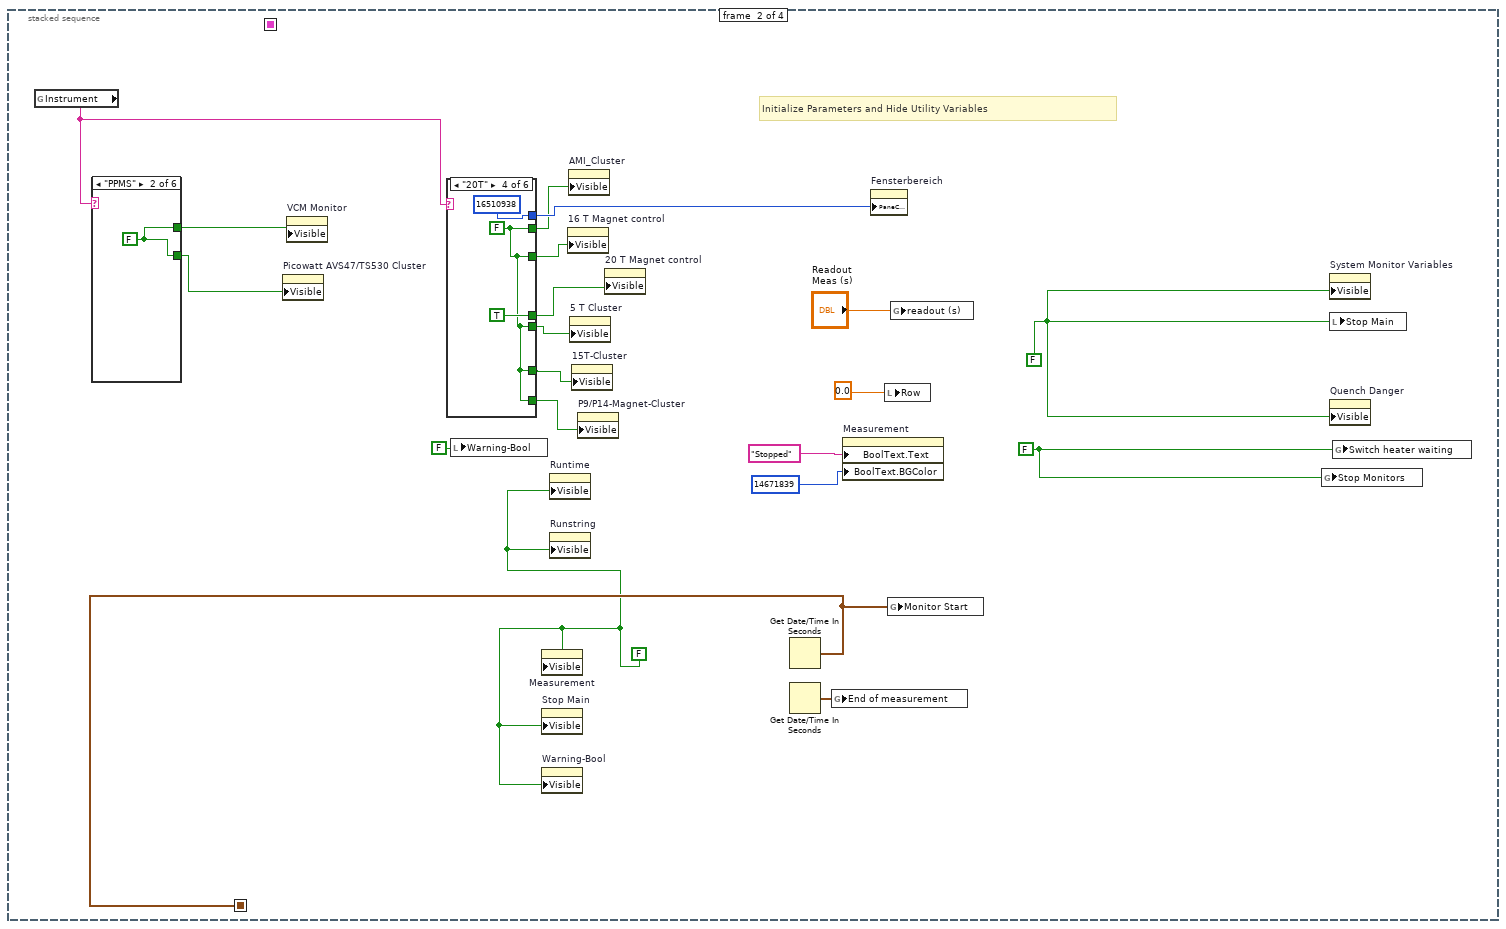
[diagram p3: hidden frame]
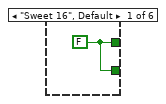
[diagram p4: hidden frame]
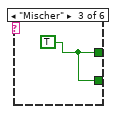
[diagram p5: hidden frame]
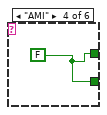
[diagram p6: hidden frame]
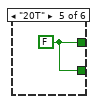
[diagram p7: hidden frame]
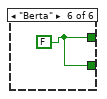
[diagram p8: hidden frame]
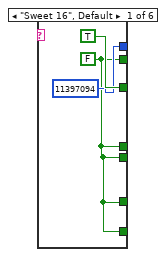
[diagram p9: hidden frame]
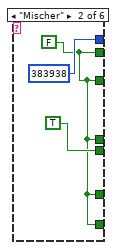
[diagram p10: hidden frame]
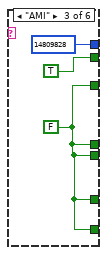
[diagram p11: hidden frame]
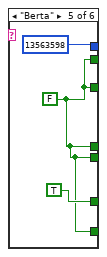
[diagram p12: hidden frame]
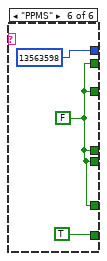
[diagram p13: hidden frame]
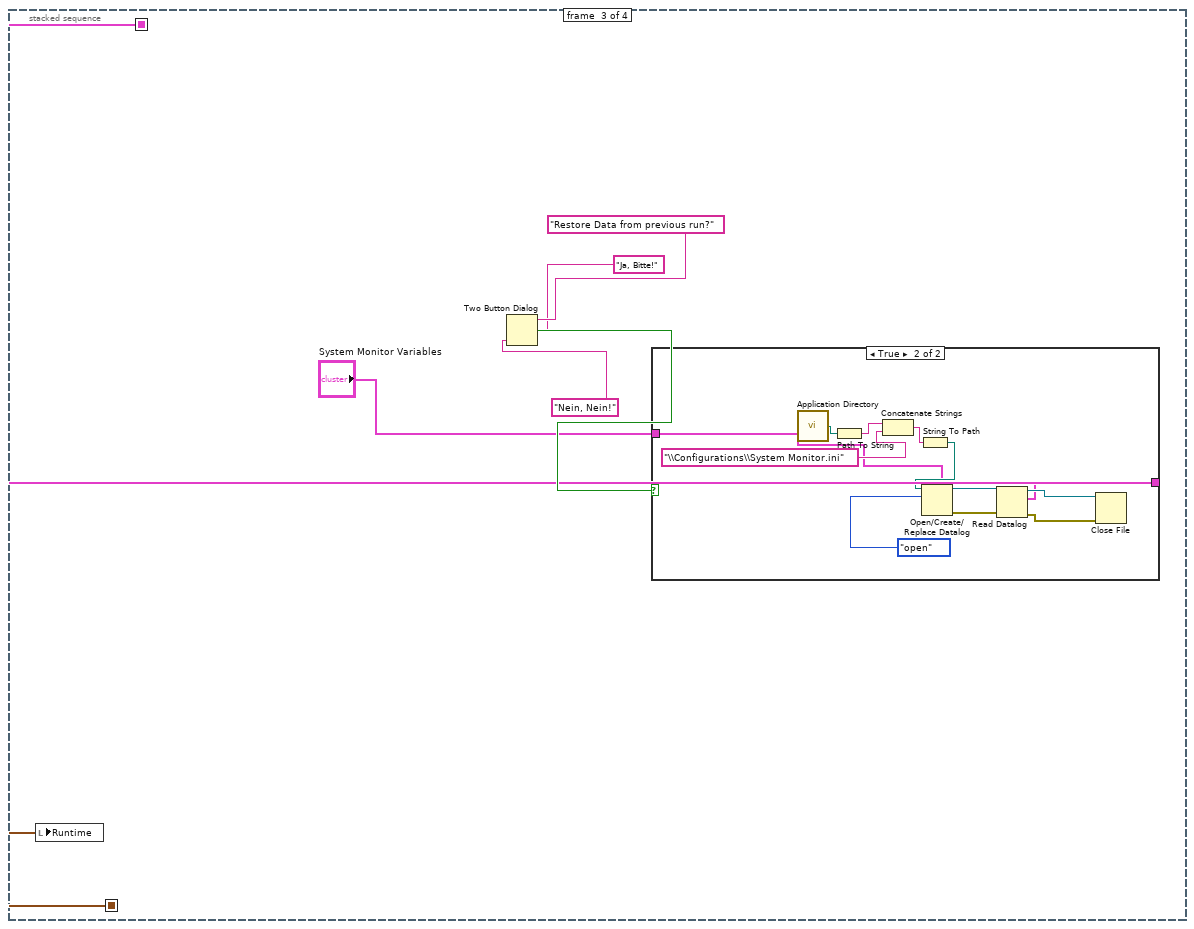
[diagram p14: hidden frame]
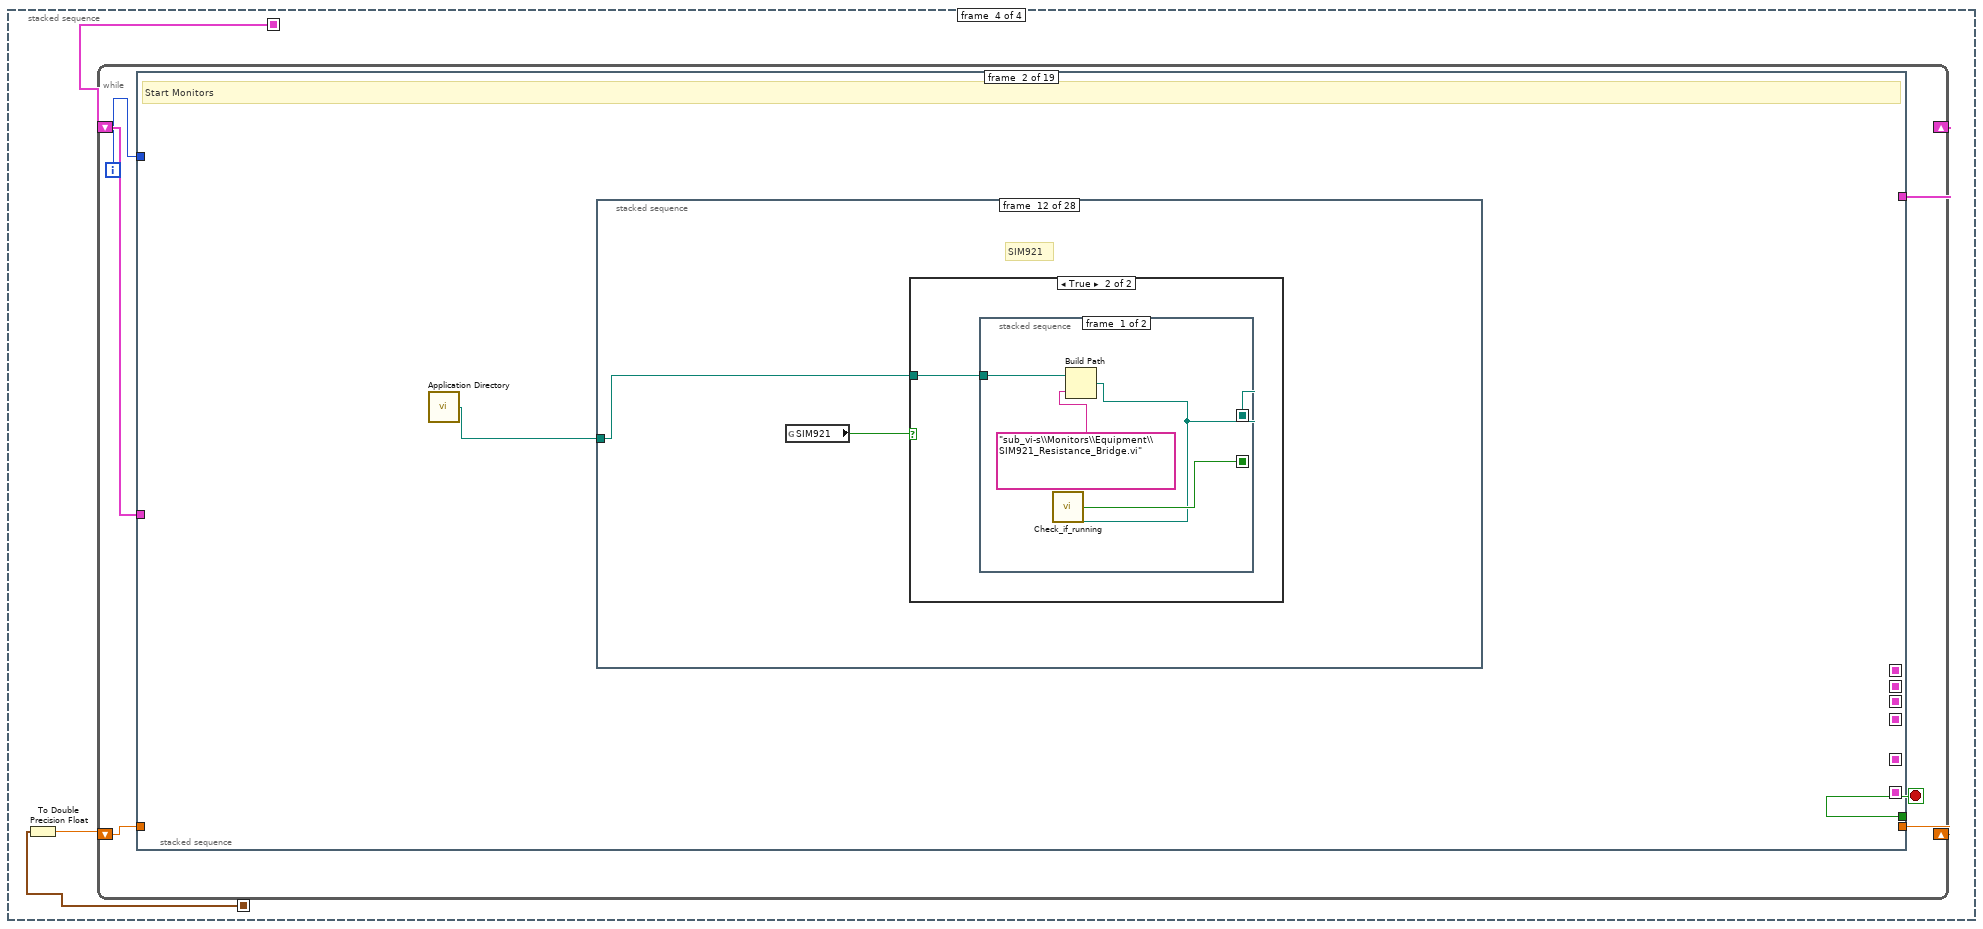
[diagram p16: hidden frame]
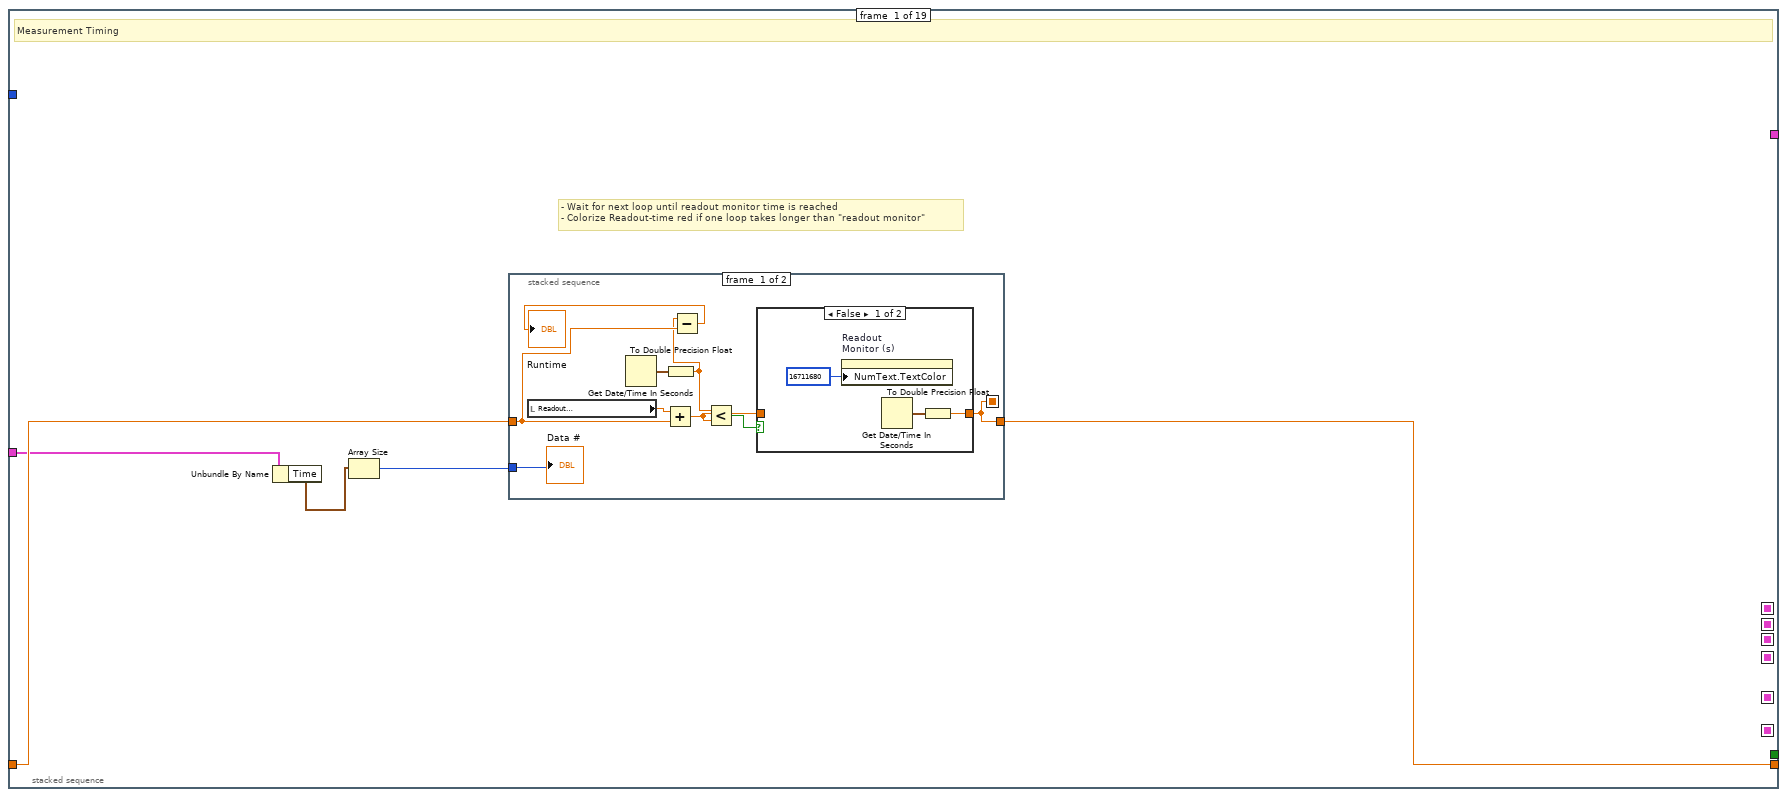
[diagram p17: hidden frame]
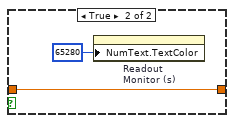
[diagram p18: hidden frame]
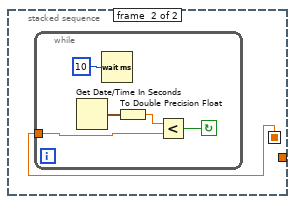
[diagram p19: hidden frame]
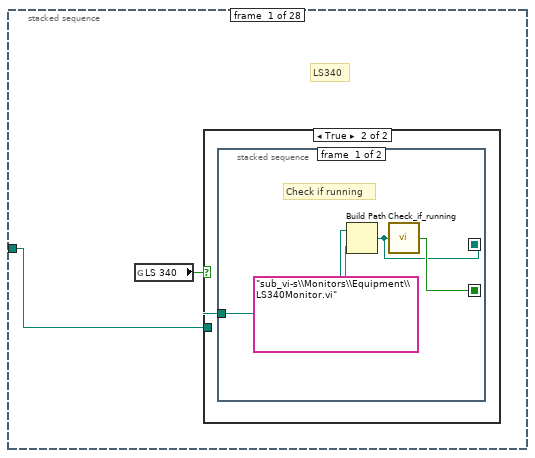
[diagram p20: hidden frame]
diagram:
  # "Variables"
  # "Equipment"
  # "Monitor Setup\nInsert\nInstrument"
  n1 = stacked-sequence {
    seq-local: [_ w17 _ _] -> [_ _ w51 w70]
    seq-local: [_ _ w55 _] -> [_ _ _ w71]
    frame #0 {
      # "Check Parameters"
      # "Check important parameters (Instrument, Insert, Command-File location) at beginning.\nIf Parameters are not set correctly, Monitor is not started"
      n2 = call "StatMon_StartWarning.vi"() -> ("String"=w4:string)  [unwired: 2 in]
      n3 = Two Button Dialog(message=w4, 1:"Fuck no!!", 2:"I am certain!") -> (T button?=w1:bool)
      n4 = case shown="True" w1 {
        frame False {
          n5 = Stop(stop? (T)=TRUE) -> ()
        }
        frame True {
        }
      }
    }
    frame #1 {
      w16 = FALSE
      w20 = FALSE
      w22 = FALSE
      # "Initialize Parameters and Hide Utility Variables"
      n6 = global read "Instrument_Setup.vi" "Instrument"() -> (w12:string)
      n7 = case shown="\"PPMS\"" w12 {
        tunnel: [w26 w27 w28 w29 w30 w31] -> w11
        tunnel: [w26 w27 w28 w29 w30 w31] -> w10
        frame "Sweet 16", Default {
          w26 = FALSE
        }
        frame "PPMS" {
          w27 = FALSE
        }
        frame "Mischer" {
          w28 = TRUE
        }
        frame "AMI" {
          w29 = FALSE
        }
        frame "20T" {
          w30 = FALSE
        }
        frame "Berta" {
          w31 = FALSE
        }
      }
      n8 = property on="Picowatt AVS47/TS530 Cluster" class="Clust (strict)"("Visible"=w10) -> ()  [unwired: 2 in, 2 out]
      n9 = property on="VCM Monitor" class="Clust (strict)"("Visible"=w11) -> ()  [unwired: 2 in, 2 out]
      n10 = case shown="\"20T\"" w12 {
        tunnel: [w32 w35 w38 TRUE w44 w49] -> w6
        tunnel: [w32 w35 TRUE w41 w44 w49] -> w9
        tunnel: [TRUE w35 w38 w41 w44 w49] -> w15
        tunnel: [u32 11397094 ("Pane Color") u32 383938 ("Pane Color") u32 14809828 ("Pane Color") u32 16510938 ("Pane Color") u32 13563598 ("Pane Color") u32 13563598 ("Pane Color")] -> w14
        tunnel: [w32 TRUE w38 w41 w44 w49] -> w13
        tunnel: [w32 w35 w38 w41 TRUE w49] -> w8
        tunnel: [w32 w35 w38 w41 w44 TRUE] -> w7
        frame "Sweet 16", Default {
          w32 = FALSE
        }
        frame "Mischer" {
          w35 = FALSE
        }
        frame "AMI" {
          w38 = FALSE
        }
        frame "20T" {
          w41 = FALSE
        }
        frame "Berta" {
          w44 = FALSE
        }
        frame "PPMS" {
          w49 = FALSE
        }
      }
      n11 = local write "Warning-Bool"(FALSE) -> ()
      n12 = property on="Measurement" class="Bool (strict)"("Visible"=w16) -> ()  [unwired: 2 in, 2 out]
      n13 = property on="Stop Main" class="Bool (strict)"("Visible"=w16) -> ()  [unwired: 2 in, 2 out]
      n14 = property on="Warning-Bool" class="Bool (strict)"("Visible"=w16) -> ()  [unwired: 2 in, 2 out]
      n15 = property on="Runtime" class="AbsTime (strict)"("Visible"=w16) -> ()  [unwired: 2 in, 2 out]
      n16 = property on="Runstring" class="Str"("Visible"=w16) -> ()  [unwired: 2 in, 2 out]
      n17 = property on="16 T Magnet control" class="Clust (strict)"("Visible"=w15) -> ()  [unwired: 2 in, 2 out]
      n18 = property on="AMI_Cluster" class="Clust (strict)"("Visible"=w9) -> ()  [unwired: 2 in, 2 out]
      n19 = property on="5 T Cluster" class="Clust (strict)"("Visible"=w13) -> ()  [unwired: 2 in, 2 out]
      n20 = property on="15T-Cluster" class="Clust (strict)"("Visible"=w8) -> ()  [unwired: 2 in, 2 out]
      n21 = property on="P9/P14-Magnet-Cluster" class="Clust (strict)"("Visible"=w7) -> ()  [unwired: 2 in, 2 out]
      n22 = property on="20 T Magnet control" class="Clust (strict)"("Visible"=w6) -> ()  [unwired: 2 in, 2 out]
      n23 = Get Date/Time In Seconds() -> (seconds since 1Jan1904=w17:timestamp)
      n24 = Get Date/Time In Seconds() -> (seconds since 1Jan1904=w19:timestamp)
      n25 = global write "Data_Display_global.vi" "End of measurement"(w19) -> ()
      n26 = property on="Measurement" class="Bool (strict)"("BoolText.Text"="Stopped", "BoolText.BGColor"=14671839) -> ()  [unwired: 2 in, 2 out]
      n27 = property on="Fensterbereich" class="Pane"("PaneColor"=w14) -> ()  [unwired: 2 in, 2 out]
      n28 = local write "Row"(0.0) -> ()
      n29 = global write "Data_Display_global.vi" "Monitor Start"(w17) -> ()
      n30 = global write "Instrument_Setup.vi" "readout (s)"("Readout \nMeas (s)") -> ()
      n31 = global write "Data_Display_global.vi" "Stop Monitors"(w22) -> ()
      n32 = property on="System Monitor Variables" class="Clust (strict)"("Visible"=w20) -> ()  [unwired: 2 in, 2 out]
      n33 = local write "Stop Main"(w20) -> ()
      n34 = property on="Quench Danger" class="Bool (strict)"("Visible"=w20) -> ()  [unwired: 2 in, 2 out]
      n35 = global write "Data_Display_global.vi" "Switch heater waiting"(w22) -> ()
    }
    frame #2 {
      n36 = local write "Runtime"(w51) -> ()
      n37 = Two Button Dialog(message="Restore Data from previous run?", 1:"Nein, Nein!", 2:"Ja, Bitte!") -> (T button?=w56:bool)
      n38 = case shown="True" w56 {
        tunnel: [w57 w60] -> w55
        tunnel: "System Monitor Variables" -> [w57 w58]
        frame False {
        }
        frame True {
          n39 = call <vilib>:"Application Directory.vi"() -> ("Application Directory"=w67:path)
          n40 = Path To String(path=w67) -> (string=w68:string)
          n41 = Concatenate Strings(w68, "\\Configurations\\System Monitor.ini") -> (w66:string)
          n42 = String To Path(string=w66) -> (path=w62:path)
          n43 = Open/Create/Replace Datalog(5:w58, 10:T38."open" ("operation (0:open)"), 11:w62) -> (0:w65:errorcluster, 3:w61:refnum<k1>)  [unwired: 1 in, 3 out]
          n44 = Read Datalog(4:w65, 7:w61) -> (0:w63:errorcluster, 2:w60:T37, 3:w64:refnum<k1>)  [unwired: 1 in]
          n45 = Close File(refnum=w64, error in=w63) -> ()  [unwired: 2 out]
        }
      }
    }
    frame #3 {
      n46 = To Double Precision Float(number=w70) -> (double precision float=w72:dbl)
      n47 = while {
        shift-right: [w75] -> _
        shift-left: w71 -> [w78]
        shift-right: [w76] -> _
        shift-left: w72 -> [w77]
        i -> [w74]
        stop <- w73 stop-if-true
        n48 = stacked-sequence {
          seq-local: [_ _ _ _ w802 _ _ _ _ _ _ _ _ _ _ _ _ _ _] -> [_ _ _ _ _ _ w940 w958 _ _ _ _ _ _ _ _ _ _ _]
          seq-local: [_ _ _ _ _ _ _ _ w1278 _ _ _ _ _ _ _ _ _ _] -> [_ _ _ _ _ _ _ _ _ w1447 _ _ _ _ _ _ _ _ _]
          seq-local: [_ _ _ _ _ _ _ _ _ w1446 _ _ _ _ _ _ _ _ _] -> [_ _ _ _ _ _ _ _ _ _ w1466 _ _ _ _ _ _ _ _]
          seq-local: [_ _ _ _ _ _ _ _ _ _ w1469 _ _ _ _ _ _ _ _] -> [_ _ _ _ _ _ _ _ _ _ _ w1545 _ _ _ _ _ _ _]
          seq-local: [_ _ _ _ _ _ _ w959 _ _ _ _ _ _ _ _ _ _ _] -> [_ _ _ _ _ _ _ _ w1279 _ _ _ _ _ _ _ _ _ _]
          seq-local: [_ _ _ _ _ _ _ _ _ _ _ w1544 _ _ _ _ _ _ _] -> [_ _ _ _ _ _ _ _ _ _ _ _ w1629 _ w1633 _ w1664 w1699 w1717]
          tunnel: w78 -> [w81 _ _ _ w803 _ _ _ _ _ _ _ _ _ _ _ _ _ _]
          tunnel: [_ _ _ _ _ _ _ _ _ _ _ _ _ _ _ _ _ w1700 _] -> w75
          tunnel: w77 -> [w83 _ _ _ _ _ _ _ _ _ _ _ _ _ _ _ _ _ _]
          tunnel: [w82 _ _ _ _ _ _ _ _ _ _ _ _ _ _ _ _ _ _] -> w76
          tunnel: [_ _ _ _ _ _ _ _ _ _ _ _ _ _ w1634 _ _ _ _] -> w73
          tunnel: w74 -> [_ _ w578 _ _ _ _ _ _ _ _ _ _ _ _ _ _ _ _]
          frame #0 {
            # "- Wait for next loop until readout monitor time is reached\n- Colorize Readout-time red if one loop takes longer than \"readout monitor\""
            # "Measurement Timing"
            n49 = Unbundle By Name(w81) -> ("Time"=w80:timestamp[])
            n50 = Array Size(array=w80) -> (size(s)=w79:i32)
            n51 = stacked-sequence {
              seq-local: [w88 _] -> [_ w98]
              tunnel: w83 -> [w87 _]
              tunnel: [w88 _] -> w82
              tunnel: w79 -> [w84 _]
              frame #0 {
                n52 = local read "Readout\nMonitor (s)"() -> (w90:dbl)
                n53 = Get Date/Time In Seconds() -> (seconds since 1Jan1904=w92:timestamp)
                n54 = Add(x=w90, y=w87) -> (x+y=w89:dbl)
                n55 = To Double Precision Float(number=w92) -> (double precision float=w86:dbl)
                n56 = Subtract(x=w86, y=w87) -> (x-y=→"Runtime":dbl)
                n57 = Less?(x=w86, y=w89) -> (x < y?=w91:bool)
                n58 = case shown="False" w91 {
                  tunnel: w89 -> [_ w96]
                  tunnel: [w93 w96] -> w88
                  frame False {
                    n59 = property on="Readout\nMonitor (s)" class="DigNum (strict)"("NumText.TextColor"=16711680) -> ()  [unwired: 2 in, 2 out]
                    n60 = Get Date/Time In Seconds() -> (seconds since 1Jan1904=w94:timestamp)
                    n61 = To Double Precision Float(number=w94) -> (double precision float=w93:dbl)
                  }
                  frame True {
                    n62 = property on="Readout\nMonitor (s)" class="DigNum (strict)"("NumText.TextColor"=65280) -> ()  [unwired: 2 in, 2 out]
                  }
                }
                "Data #" <- w84
              }
              frame #1 {
                n63 = while {
                  tunnel: w98 -> [w100]
                  stop <- w101 continue-if-true
                  n64 = Get Date/Time In Seconds() -> (seconds since 1Jan1904=w103:timestamp)
                  n65 = Wait (ms)(milliseconds to wait=10) -> ()  [unwired: 1 out]
                  n66 = To Double Precision Float(number=w103) -> (double precision float=w102:dbl)
                  n67 = Less?(x=w102, y=w100) -> (x < y?=w101:bool)
                }
              }
            }
          }
          frame #1 {
            # "Start Monitors"
            n68 = call <vilib>:"Application Directory.vi"() -> ("Application Directory"=w104:path)
            n69 = stacked-sequence {
              tunnel: w104 -> [w105 _ w123 w133 w149 w158 w168 w178 w192 _ _ w223 w249 w285 w332 w383 w434 w444 w454 w464 w474 w485 w512 w522 w535 w552 w567 _]
              frame #0 {
                # "LS340"
                n70 = global read "Instrument_Setup.vi" "LS 340"() -> (w106:bool)
                n71 = case shown="True" w106 {
                  tunnel: w105 -> [_ w107]
                  frame False {
                  }
                  frame True {
                    n72 = stacked-sequence {
                      seq-local: [w109 _] -> [_ w113]
                      seq-local: [w111 _] -> [_ w112]
                      tunnel: w107 -> [w108 _]
                      frame #0 {
                        # "Check if running"
                        n73 = Build Path(base path=w108, name or relative path="sub_vi-s\\Monitors\\Equipment\\LS340Monitor.vi") -> (appended path=w109:path)
                        n74 = call "Check_if_running.vi"("VI-Pfad"=w109) -> ("Running"=w111:bool)
                      }
                      frame #1 {
                        n75 = case shown="False" w112 {
                          tunnel: w113 -> [w114 _]
                          frame False {
                            # "Start Monitor"
                            n76 = call "Start_Vi.vi"("VI-Pfad"=w114) -> ()  [unwired: 1 in]
                          }
                          frame True {
                          }
                        }
                      }
                    }
                  }
                }
              }
              frame #1 {
                # "LS350"
                n77 = global read "Instrument_Setup.vi" "LS 350"() -> (w115:bool)
                n78 = case shown="True" w115 {
                  frame False {
                  }
                  frame True {
                    n79 = stacked-sequence {
                      seq-local: [w116 _] -> [_ w121]
                      seq-local: [w119 _] -> [_ w120]
                      frame #0 {
                        n80 = call <vilib>:"Application Directory.vi"() -> ("Application Directory"=w118:path)
                        n81 = Build Path(base path=w118, name or relative path="sub_vi-s\\Monitors\\Equipment\\LS350Monitor.vi") -> (appended path=w116:path)
                        n82 = call "Check_if_running.vi"("VI-Pfad"=w116) -> ("Running"=w119:bool)
                      }
                      frame #1 {
                        n83 = case shown="False" w120 {
                          tunnel: w121 -> [w122 _]
                          frame False {
                            # "Start Monitor"
                            n84 = call "Start_Vi.vi"("VI-Pfad"=w122) -> ()  [unwired: 1 in]
                          }
                          frame True {
                          }
                        }
                      }
                    }
                  }
                }
              }
              frame #2 {
                # "LS 370 start über T-control"
                n85 = global read "Instrument_Setup.vi" "T-control"() -> (w124:string)
                n86 = case shown="\"LS370\"" w124 {
                  tunnel: w123 -> [_ w125]
                  frame "None", Default {
                  }
                  frame "LS370" {
                    n87 = stacked-sequence {
                      seq-local: [w127 _] -> [_ w131]
                      seq-local: [w129 _] -> [_ w130]
                      tunnel: w125 -> [w126 _]
                      frame #0 {
                        n88 = Build Path(base path=w126, name or relative path="sub_vi-s\\Monitors\\Equipment\\LS370Monitor.vi") -> (appended path=w127:path)
                        n89 = call "Check_if_running.vi"("VI-Pfad"=w127) -> ("Running"=w129:bool)
                      }
                      frame #1 {
                        n90 = case shown="False" w130 {
                          tunnel: w131 -> [w132 _]
                          frame False {
                            # "Start Monitor"
                            n91 = call "Start_Vi.vi"("VI-Pfad"=w132) -> ()  [unwired: 1 in]
                          }
                          frame True {
                          }
                        }
                      }
                    }
                  }
                }
              }
              frame #3 {
                # "LS 370 start über Insert JT"
                n92 = global read "Instrument_Setup.vi" "Insert"() -> (w134:string)
                n93 = case shown="\"JT\"" w134 {
                  tunnel: w133 -> [_ w135]
                  frame "None", Default {
                  }
                  frame "JT" {
                    n94 = stacked-sequence {
                      seq-local: [w137 _] -> [_ w141]
                      seq-local: [w139 _] -> [_ w140]
                      tunnel: w135 -> [w136 _]
                      frame #0 {
                        n95 = Build Path(base path=w136, name or relative path="sub_vi-s\\Monitors\\Equipment\\LS370Monitor.vi") -> (appended path=w137:path)
                        n96 = call "Check_if_running.vi"("VI-Pfad"=w137) -> ("Running"=w139:bool)
                      }
                      frame #1 {
                        n97 = case shown="False" w140 {
                          tunnel: w141 -> [w142 _]
                          frame False {
                            # "Start Monitor"
                            n98 = call "Start_Vi.vi"("VI-Pfad"=w142) -> ()  [unwired: 1 in]
                          }
                          frame True {
                          }
                        }
                      }
                    }
                  }
                }
              }
              frame #4 {
                # "LS 370 readout no temperature Control"
                n99 = global read "Instrument_Setup.vi" "LS 370"() -> (w145:bool)
                n100 = Build Path(base path=w149, name or relative path="sub_vi-s\\Monitors\\Equipment\\LS370Monitor.vi") -> (appended path=w147:path)
                n101 = call "Check_if_running.vi"("VI-Pfad"=w147) -> ("Running"=w146:bool)
                n102 = Not(x=w146) -> (.not. x?=w144:bool)
                n103 = And(x=w144, y=w145) -> (x .and. y?=w143:bool)
                n104 = case shown="False" w143 {
                  tunnel: w149 -> [_ w150]
                  frame False {
                  }
                  frame True {
                    n105 = stacked-sequence {
                      seq-local: [w152 _] -> [_ w155]
                      seq-local: [w151 _] -> [_ w156]
                      tunnel: w150 -> [w154 _]
                      frame #0 {
                        n106 = Build Path(base path=w154, name or relative path="sub_vi-s\\Monitors\\Equipment\\LS370_only_readout_Monitor.vi") -> (appended path=w152:path)
                        n107 = call "Check_if_running.vi"("VI-Pfad"=w152) -> ("Running"=w151:bool)
                      }
                      frame #1 {
                        n108 = case shown="False" w156 {
                          tunnel: w155 -> [w157 _]
                          frame False {
                            n109 = call "Start_Vi.vi"("VI-Pfad"=w157) -> ()  [unwired: 1 in]
                          }
                          frame True {
                          }
                        }
                      }
                    }
                  }
                }
              }
              frame #5 {
                # "LS 372"
                n110 = global read "Instrument_Setup.vi" "T-control"() -> (w159:string)
                n111 = case shown="\"None\", Default" w159 {
                  tunnel: w158 -> [_ w160]
                  frame "None", Default {
                  }
                  frame "LS372" {
                    n112 = stacked-sequence {
                      seq-local: [w162 _] -> [_ w166]
                      seq-local: [w164 _] -> [_ w165]
                      tunnel: w160 -> [w161 _]
                      frame #0 {
                        n113 = Build Path(base path=w161, name or relative path="sub_vi-s\\Monitors\\Equipment\\LS372Monitor.vi") -> (appended path=w162:path)
                        n114 = call "Check_if_running.vi"("VI-Pfad"=w162) -> ("Running"=w164:bool)
                      }
                      frame #1 {
                        n115 = case shown="False" w165 {
                          tunnel: w166 -> [w167 _]
                          frame False {
                            # "Start Vi"
                            n116 = call "Start_Vi.vi"("VI-Pfad"=w167) -> ()  [unwired: 1 in]
                          }
                          frame True {
                          }
                        }
                      }
                    }
                  }
                }
              }
              frame #6 {
                n117 = global read "Instrument_Setup.vi" "T-control"() -> (w169:string)
                n118 = case shown="\"ITC503\"" w169 {
                  tunnel: w168 -> [_ w170]
                  frame "None", Default {
                  }
                  frame "ITC503" {
                    n119 = stacked-sequence {
                      seq-local: [w172 _] -> [_ w176]
                      seq-local: [w174 _] -> [_ w175]
                      tunnel: w170 -> [w171 _]
                      frame #0 {
                        n120 = Build Path(base path=w171, name or relative path="sub_vi-s\\Monitors\\Equipment\\ITC503controlMonitor.vi") -> (appended path=w172:path)
                        n121 = call "Check_if_running.vi"("VI-Pfad"=w172) -> ("Running"=w174:bool)
                      }
                      frame #1 {
                        n122 = case shown="False" w175 {
                          tunnel: w176 -> [w177 _]
                          frame False {
                            # "Start Vi"
                            n123 = call "Start_Vi.vi"("VI-Pfad"=w177) -> ()  [unwired: 1 in]
                          }
                          frame True {
                          }
                        }
                      }
                    }
                  }
                }
              }
              frame #7 {
                n124 = global read "Instrument_Setup.vi" "T-control"() -> (w179:string)
                n125 = case shown="\"PPMS\"" w179 {
                  tunnel: w178 -> [_ w180]
                  frame "None", Default {
                  }
                  frame "PPMS" {
                    n126 = stacked-sequence {
                      seq-local: [w182 _] -> [_ w186]
                      seq-local: [w184 _] -> [_ w185]
                      tunnel: w180 -> [w181 _]
                      frame #0 {
                        n127 = Build Path(base path=w181, name or relative path="sub_vi-s\\Monitors\\Instrument\\P9-P14TMonitor.vi") -> (appended path=w182:path)
                        n128 = call "Check_if_running.vi"("VI-Pfad"=w182) -> ("Running"=w184:bool)
                      }
                      frame #1 {
                        n129 = case shown="False" w185 {
                          tunnel: w186 -> [w187 _]
                          frame False {
                            # "Start Vi"
                            n130 = call "Start_Vi.vi"("VI-Pfad"=w187) -> ()  [unwired: 1 in]
                          }
                          frame True {
                          }
                        }
                      }
                    }
                  }
                }
              }
              frame #8 {
                # "LS 372 only readout Monitor no temperture Control"
                n131 = global read "Instrument_Setup.vi" "LS 372"() -> (w191:bool)
                n132 = Build Path(base path=w192, name or relative path="sub_vi-s\\Monitors\\Equipment\\LS372Monitor.vi") -> (appended path=w194:path)
                n133 = call "Check_if_running.vi"("VI-Pfad"=w194) -> ("Running"=w193:bool)
                n134 = Not(x=w193) -> (.not. x?=w190:bool)
                n135 = And(x=w191, y=w190) -> (x .and. y?=w189:bool)
                n136 = case shown="True" w189 {
                  tunnel: w192 -> [_ w195]
                  frame False {
                  }
                  frame True {
                    n137 = stacked-sequence {
                      seq-local: [w197 _] -> [_ w201]
                      seq-local: [w196 _] -> [_ w200]
                      tunnel: w195 -> [w198 _]
                      frame #0 {
                        n138 = Build Path(base path=w198, name or relative path="sub_vi-s\\Monitors\\Equipment\\LS372_only_readout_Monitor.vi") -> (appended path=w196:path)
                        n139 = call "Check_if_running.vi"("VI-Pfad"=w196) -> ("Running"=w197:bool)
                      }
                      frame #1 {
                        n140 = case shown="True" w201 {
                          tunnel: w200 -> [_ w202]
                          frame False {
                          }
                          frame True {
                            n141 = call "Start_Vi.vi"("VI-Pfad"=w202) -> ()  [unwired: 1 in]
                          }
                        }
                      }
                    }
                  }
                }
              }
              frame #9 {
                # "AH2700"
                n142 = global read "Instrument_Setup.vi" "AH 2700"() -> (w203:bool)
                n143 = case shown="True" w203 {
                  frame False {
                  }
                  frame True {
                    n144 = stacked-sequence {
                      frame #0 {
                        # "Set frequency"
                        n145 = global read "Instrument_Setup.vi" "AH 2700 Parameters"() -> (w205:T42)
                        n146 = Unbundle By Name(w205) -> ("AH Frequency"=w204:dbl)
                        n147 = global write "global.vi" "Frequency"(w204) -> ()
                      }
                      frame #1 {
                        n148 = stacked-sequence {
                          seq-local: [w206 _] -> [_ w211]
                          seq-local: [w209 _] -> [_ w210]
                          frame #0 {
                            n149 = call <vilib>:"Application Directory.vi"() -> ("Application Directory"=w208:path)
                            n150 = Build Path(base path=w208, name or relative path="sub_vi-s\\Monitors\\Equipment\\AH2700Monitor.vi") -> (appended path=w206:path)
                            n151 = call "Check_if_running.vi"("VI-Pfad"=w206) -> ("Running"=w209:bool)
                          }
                          frame #1 {
                            n152 = case shown="False" w210 {
                              tunnel: w211 -> [w212 _]
                              frame False {
                                # "Start Monitor"
                                n153 = call "Start_Vi.vi"("VI-Pfad"=w212) -> ()  [unwired: 1 in]
                              }
                              frame True {
                              }
                            }
                          }
                        }
                      }
                    }
                  }
                }
              }
              frame #10 {
                # "AH2500"
                n154 = global read "Instrument_Setup.vi" "AH 2500"() -> (w213:bool)
                n155 = case shown="True" w213 {
                  frame False {
                  }
                  frame True {
                    n156 = stacked-sequence {
                      frame #0 {
                        # "Set frequency"
                        n157 = global read "Instrument_Setup.vi" "AH 2700 Parameters"() -> (w215:T42)
                        n158 = Unbundle By Name(w215) -> ("AH Frequency"=w214:dbl)
                        n159 = global write "global.vi" "Frequency"(w214) -> ()
                      }
                      frame #1 {
                        n160 = stacked-sequence {
                          seq-local: [w216 _] -> [_ w221]
                          seq-local: [w219 _] -> [_ w220]
                          frame #0 {
                            n161 = call <vilib>:"Application Directory.vi"() -> ("Application Directory"=w218:path)
                            n162 = Build Path(base path=w218, name or relative path="sub_vi-s\\Monitors\\Equipment\\AH2500Monitor.vi") -> (appended path=w216:path)
                            n163 = call "Check_if_running.vi"("VI-Pfad"=w216) -> ("Running"=w219:bool)
                          }
                          frame #1 {
                            n164 = case shown="False" w220 {
                              tunnel: w221 -> [w222 _]
                              frame False {
                                # "Start Monitor"
                                n165 = call "Start_Vi.vi"("VI-Pfad"=w222) -> ()  [unwired: 1 in]
                              }
                              frame True {
                              }
                            }
                          }
                        }
                      }
                    }
                  }
                }
              }
              frame #11 {
                # "SIM921"
                n166 = global read "Instrument_Setup.vi" "SIM921"() -> (w224:bool)
                n167 = case shown="True" w224 {
                  tunnel: w223 -> [_ w225]
                  frame False {
                  }
                  frame True {
                    n168 = stacked-sequence {
                      seq-local: [w227 _] -> [_ w231]
                      seq-local: [w229 _] -> [_ w230]
                      tunnel: w225 -> [w226 _]
                      frame #0 {
                        n169 = Build Path(base path=w226, name or relative path="sub_vi-s\\Monitors\\Equipment\\SIM921_Resistance_Bridge.vi") -> (appended path=w227:path)
                        n170 = call "Check_if_running.vi"("VI-Pfad"=w227) -> ("Running"=w229:bool)
                      }
                      frame #1 {
                        n171 = case shown="False" w230 {
                          tunnel: w231 -> [w232 _]
                          frame False {
                            # "Start Monitor"
                            n172 = call "Start_Vi.vi"("VI-Pfad"=w232) -> ()  [unwired: 1 in]
                          }
                          frame True {
                          }
                        }
                      }
                    }
                  }
                }
              }
              frame #12 {
                # "SR830"
                n173 = global read "Instrument_Setup.vi" "Lock In #2"() -> (w238:bool)
                n174 = global read "Instrument_Setup.vi" "Choose Lock-In #2"() -> (w242:u16)
                n175 = global read "Instrument_Setup.vi" "Choose Lock-In #1"() -> (w247:u16)
                n176 = global read "Instrument_Setup.vi" "Choose Lock-In #3"() -> (w237:u16)
                n177 = global read "Instrument_Setup.vi" "Lock In #1"() -> (w244:bool)
                n178 = global read "Instrument_Setup.vi" "Lock In #3"() -> (w233:bool)
                n179 = Build Path(base path=w249, name or relative path="sub_vi-s\\Monitors\\Equipment\\SR830Monitor.vi") -> (appended path=w248:path)
                n180 = Equal?(x=w242, y=0) -> (x = y?=w239:bool)
                n181 = Equal?(x=w247, y=0) -> (x = y?=w245:bool)
                n182 = Equal?(x=w237, y=0) -> (x = y?=w234:bool)
                n183 = And(x=w239, y=w238) -> (x .and. y?=w240:bool)
                n184 = And(x=w245, y=w244) -> (x .and. y?=w243:bool)
                n185 = And(x=w234, y=w233) -> (x .and. y?=w235:bool)
                n186 = stacked-sequence {
                  tunnel: w248 -> [w252 w262 w272]
                  tunnel: w243 -> [w251 _ _]
                  tunnel: w240 -> [_ w261 _]
                  tunnel: w235 -> [_ _ w271]
                  frame #0 {
                    n187 = case shown="True" w251 {
                      tunnel: w252 -> [_ w253]
                      frame False {
                      }
                      frame True {
                        n188 = stacked-sequence {
                          seq-local: [w256 _] -> [_ w257]
                          seq-local: [w254 _] -> [_ w258]
                          tunnel: [w254 _] -> _
                          tunnel: w253 -> [w256 _]
                          frame #0 {
                            n189 = global read "Data_Display_global.vi" "Lock-In-Running-Cluster"() -> (w255:T43)
                            n190 = Unbundle By Name(w255) -> ("SR830-Running"=w254:bool)
                          }
                          frame #1 {
                            n191 = case shown="False" w258 {
                              tunnel: w257 -> [_ _]
                              tunnel: w257 -> [w260 _]
                              frame False {
                                # "Start Monitor"
                                n192 = call "Start_SR830.vi"("Lock-in Reference"=u16 0, "VI-Pfad"=w260) -> ()
                              }
                              frame True {
                              }
                            }
                          }
                        }
                      }
                    }
                  }
                  frame #1 {
                    n193 = case shown="True" w261 {
                      tunnel: w262 -> [_ w263]
                      frame False {
                      }
                      frame True {
                        n194 = stacked-sequence {
                          seq-local: [w266 _] -> [_ w268]
                          seq-local: [w264 _] -> [_ w267]
                          tunnel: [w264 _] -> _
                          tunnel: w263 -> [w266 _]
                          frame #0 {
                            n195 = global read "Data_Display_global.vi" "Lock-In-Running-Cluster"() -> (w265:T43)
                            n196 = Unbundle By Name(w265) -> ("SR830-Running 2"=w264:bool)
                          }
                          frame #1 {
                            n197 = case shown="False" w267 {
                              tunnel: w268 -> [w270 _]
                              frame False {
                                # "Start Monitor"
                                n198 = call "Start_SR830.vi"("Lock-in Reference"=u16 1, "VI-Pfad"=w270) -> ()
                              }
                              frame True {
                              }
                            }
                          }
                        }
                      }
                    }
                  }
                  frame #2 {
                    n199 = case shown="True" w271 {
                      tunnel: w272 -> [_ w273]
                      frame False {
                      }
                      frame True {
                        n200 = stacked-sequence {
                          seq-local: [w276 _] -> [_ w278]
                          seq-local: [w274 _] -> [_ w277]
                          tunnel: [w274 _] -> _
                          tunnel: w273 -> [w276 _]
                          frame #0 {
                            n201 = global read "Data_Display_global.vi" "Lock-In-Running-Cluster"() -> (w275:T43)
                            n202 = Unbundle By Name(w275) -> ("SR830-Running 3"=w274:bool)
                          }
                          frame #1 {
                            n203 = case shown="False" w277 {
                              tunnel: w278 -> [w280 _]
                              frame False {
                                # "Start Monitor"
                                n204 = call "Start_SR830.vi"("Lock-in Reference"=u16 2, "VI-Pfad"=w280) -> ()
                              }
                              frame True {
                              }
                            }
                          }
                        }
                      }
                    }
                  }
                }
              }
              frame #13 {
                # "PE7265"
                n205 = global read "Instrument_Setup.vi" "Lock In #3"() -> (w282:bool)
                n206 = global read "Instrument_Setup.vi" "Lock In #2"() -> (w283:bool)
                n207 = global read "Instrument_Setup.vi" "Lock In #1"() -> (w287:bool)
                n208 = case shown="True" w283 {
                  tunnel: [FALSE w295] -> w284
                  frame False {
                  }
                  frame True {
                    n209 = global read "Instrument_Setup.vi" "Choose Lock-In #2"() -> (w297:u16)
                    n210 = Equal?(x=w297, y=1) -> (x = y?=w295:bool)
                  }
                }
                n211 = case shown="True" w282 {
                  tunnel: [FALSE w291] -> w281
                  frame False {
                  }
                  frame True {
                    n212 = global read "Instrument_Setup.vi" "Choose Lock-In #3"() -> (w293:u16)
                    n213 = Equal?(x=w293, y=1) -> (x = y?=w291:bool)
                  }
                }
                n214 = case shown="True" w287 {
                  tunnel: [FALSE w299] -> w286
                  frame False {
                  }
                  frame True {
                    n215 = global read "Instrument_Setup.vi" "Choose Lock-In #1"() -> (w301:u16)
                    n216 = Equal?(x=w301, y=1) -> (x = y?=w299:bool)
                  }
                }
                n217 = Build Path(base path=w285, name or relative path="sub_vi-s\\Monitors\\Equipment\\PE7265Monitor.vi") -> (appended path=w288:path)
                n218 = stacked-sequence {
                  tunnel: w288 -> [w302 w312 w322]
                  tunnel: w281 -> [_ _ w323]
                  tunnel: w284 -> [_ w313 _]
                  tunnel: w286 -> [w303 _ _]
                  frame #0 {
                    n219 = case shown="True" w303 {
                      tunnel: w302 -> [_ w304]
                      frame False {
                      }
                      frame True {
                        n220 = stacked-sequence {
                          seq-local: [w307 _] -> [_ w308]
                          seq-local: [w305 _] -> [_ w309]
                          tunnel: w304 -> [w307 _]
                          frame #0 {
                            n221 = global read "Data_Display_global.vi" "Lock-In-Running-Cluster"() -> (w306:T43)
                            n222 = Unbundle By Name(w306) -> ("PE7265-running"=w305:bool)
                          }
                          frame #1 {
                            n223 = case shown="False" w309 {
                              tunnel: w308 -> [w311 _]
                              frame False {
                                # "Start Monitor"
                                n224 = call "Start_PE7265.vi"("Lock-in Reference"=0, "VI-Pfad"=w311) -> ()
                              }
                              frame True {
                              }
                            }
                          }
                        }
                      }
                    }
                  }
                  frame #1 {
                    n225 = case shown="True" w313 {
                      tunnel: w312 -> [_ w314]
                      frame False {
                      }
                      frame True {
                        n226 = stacked-sequence {
                          seq-local: [w317 _] -> [_ w318]
                          seq-local: [w315 _] -> [_ w319]
                          tunnel: w314 -> [w317 _]
                          frame #0 {
                            n227 = global read "Data_Display_global.vi" "Lock-In-Running-Cluster"() -> (w316:T43)
                            n228 = Unbundle By Name(w316) -> ("PE7265-running"=w315:bool)
                          }
                          frame #1 {
                            n229 = case shown="False" w319 {
                              tunnel: w318 -> [w320 _]
                              frame False {
                                # "Start Monitor"
                                n230 = call "Start_PE7265.vi"("Lock-in Reference"=1, "VI-Pfad"=w320) -> ()
                              }
                              frame True {
                              }
                            }
                          }
                        }
                      }
                    }
                  }
                  frame #2 {
                    n231 = case shown="True" w323 {
                      tunnel: w322 -> [_ w324]
                      frame False {
                      }
                      frame True {
                        n232 = stacked-sequence {
                          seq-local: [w327 _] -> [_ w328]
                          seq-local: [w325 _] -> [_ w329]
                          tunnel: w324 -> [w327 _]
                          frame #0 {
                            n233 = global read "Data_Display_global.vi" "Lock-In-Running-Cluster"() -> (w326:T43)
                            n234 = Unbundle By Name(w326) -> ("PE7265-running"=w325:bool)
                          }
                          frame #1 {
                            n235 = case shown="False" w329 {
                              tunnel: w328 -> [w330 _]
                              frame False {
                                # "Start Monitor"
                                n236 = call "Start_PE7265.vi"("Lock-in Reference"=2, "VI-Pfad"=w330) -> ()
                              }
                              frame True {
                              }
                            }
                          }
                        }
                      }
                    }
                  }
                }
              }
              frame #14 {
                # "LIA7230"
                n237 = global read "Instrument_Setup.vi" "Lock In #1"() -> (w334:bool)
                n238 = global read "Instrument_Setup.vi" "Lock In #3"() -> (w336:bool)
                n239 = global read "Instrument_Setup.vi" "Lock In #2"() -> (w337:bool)
                n240 = case shown="True" w337 {
                  tunnel: [FALSE w350] -> w338
                  frame False {
                  }
                  frame True {
                    n241 = global read "Instrument_Setup.vi" "Choose Lock-In #2"() -> (w352:u16)
                    n242 = Equal?(x=w352, y=2) -> (x = y?=w350:bool)
                  }
                }
                n243 = case shown="True" w336 {
                  tunnel: [FALSE w346] -> w335
                  frame False {
                  }
                  frame True {
                    n244 = global read "Instrument_Setup.vi" "Choose Lock-In #3"() -> (w348:u16)
                    n245 = Equal?(x=w348, y=2) -> (x = y?=w346:bool)
                  }
                }
                n246 = case shown="True" w334 {
                  tunnel: [FALSE w342] -> w333
                  frame False {
                  }
                  frame True {
                    n247 = global read "Instrument_Setup.vi" "Choose Lock-In #1"() -> (w344:u16)
                    n248 = Equal?(x=w344, y=2) -> (x = y?=w342:bool)
                  }
                }
                n249 = Build Path(base path=w332, name or relative path="sub_vi-s\\Monitors\\Equipment\\LIA7230Monitor.vi") -> (appended path=w339:path)
                n250 = stacked-sequence {
                  tunnel: w339 -> [w353 w363 w373]
                  tunnel: w335 -> [_ _ w374]
                  tunnel: w338 -> [_ w364 _]
                  tunnel: w333 -> [w354 _ _]
                  frame #0 {
                    n251 = case shown="True" w354 {
                      tunnel: w353 -> [_ w355]
                      frame False {
                      }
                      frame True {
                        n252 = stacked-sequence {
                          seq-local: [w358 _] -> [_ w359]
                          seq-local: [w356 _] -> [_ w360]
                          tunnel: w355 -> [w358 _]
                          frame #0 {
                            n253 = global read "Data_Display_global.vi" "Lock-In-Running-Cluster"() -> (w357:T43)
                            n254 = Unbundle By Name(w357) -> ("LIA7230-Running"=w356:bool)
                          }
                          frame #1 {
                            n255 = case shown="False" w360 {
                              tunnel: w359 -> [w362 _]
                              frame False {
                                # "Start Monitor"
                                n256 = call "Start_PE7265.vi"("Lock-in Reference"=0, "VI-Pfad"=w362) -> ()
                              }
                              frame True {
                              }
                            }
                          }
                        }
                      }
                    }
                  }
                  frame #1 {
                    n257 = case shown="False" w364 {
                      tunnel: w363 -> [_ w365]
                      frame False {
                      }
                      frame True {
                        n258 = stacked-sequence {
                          seq-local: [w368 _] -> [_ w369]
                          seq-local: [w366 _] -> [_ w370]
                          tunnel: w365 -> [w368 _]
                          frame #0 {
                            n259 = global read "Data_Display_global.vi" "Lock-In-Running-Cluster"() -> (w367:T43)
                            n260 = Unbundle By Name(w367) -> ("LIA7230-Running 2"=w366:bool)
                          }
                          frame #1 {
                            n261 = case shown="False" w370 {
                              tunnel: w369 -> [w371 _]
                              frame False {
                                # "Start Monitor"
                                n262 = call "Start_PE7265.vi"("Lock-in Reference"=1, "VI-Pfad"=w371) -> ()
                              }
                              frame True {
                              }
                            }
                          }
                        }
                      }
                    }
                  }
                  frame #2 {
                    n263 = case shown="True" w374 {
                      tunnel: w373 -> [_ w375]
                      frame False {
                      }
                      frame True {
                        n264 = stacked-sequence {
                          seq-local: [w378 _] -> [_ w379]
                          seq-local: [w376 _] -> [_ w380]
                          tunnel: w375 -> [w378 _]
                          frame #0 {
                            n265 = global read "Data_Display_global.vi" "Lock-In-Running-Cluster"() -> (w377:T43)
                            n266 = Unbundle By Name(w377) -> ("LIA7230-Running 3"=w376:bool)
                          }
                          frame #1 {
                            n267 = case shown="False" w380 {
                              tunnel: w379 -> [w381 _]
                              frame False {
                                # "Start Monitor"
                                n268 = call "Start_PE7265.vi"("Lock-in Reference"=2, "VI-Pfad"=w381) -> ()
                              }
                              frame True {
                              }
                            }
                          }
                        }
                      }
                    }
                  }
                }
              }
              frame #15 {
                # "zurich lock-in"
                n269 = global read "Instrument_Setup.vi" "Lock In #3"() -> (w385:bool)
                n270 = global read "Instrument_Setup.vi" "Lock In #2"() -> (w386:bool)
                n271 = global read "Instrument_Setup.vi" "Lock In #1"() -> (w389:bool)
                n272 = case shown="True" w386 {
                  tunnel: [FALSE w397] -> w387
                  frame False {
                  }
                  frame True {
                    n273 = global read "Instrument_Setup.vi" "Choose Lock-In #2"() -> (w399:u16)
                    n274 = Equal?(x=w399, y=3) -> (x = y?=w397:bool)
                  }
                }
                n275 = case shown="True" w385 {
                  tunnel: [FALSE w393] -> w384
                  frame False {
                  }
                  frame True {
                    n276 = global read "Instrument_Setup.vi" "Choose Lock-In #3"() -> (w395:u16)
                    n277 = Equal?(x=w395, y=3) -> (x = y?=w393:bool)
                  }
                }
                n278 = case shown="True" w389 {
                  tunnel: [FALSE w401] -> w388
                  frame False {
                  }
                  frame True {
                    n279 = global read "Instrument_Setup.vi" "Choose Lock-In #1"() -> (w403:u16)
                    n280 = Equal?(x=w403, y=3) -> (x = y?=w401:bool)
                  }
                }
                n281 = Build Path(base path=w383, name or relative path="sub_vi-s\\Monitors\\Equipment\\zurichinstMonitor.vi") -> (appended path=w390:path)
                n282 = stacked-sequence {
                  tunnel: w390 -> [w404 w414 w424]
                  tunnel: w384 -> [_ _ w425]
                  tunnel: w387 -> [_ w415 _]
                  tunnel: w388 -> [w405 _ _]
                  frame #0 {
                    n283 = case shown="True" w405 {
                      tunnel: w404 -> [_ w406]
                      frame False {
                      }
                      frame True {
                        n284 = stacked-sequence {
                          seq-local: [w409 _] -> [_ w410]
                          seq-local: [w407 _] -> [_ w411]
                          tunnel: w406 -> [w409 _]
                          frame #0 {
                            n285 = global read "Data_Display_global.vi" "Lock-In-Running-Cluster"() -> (w408:T43)
                            n286 = Unbundle By Name(w408) -> ("zurich_Lock_in-running"=w407:bool)
                          }
                          frame #1 {
                            n287 = case shown="False" w411 {
                              tunnel: w410 -> [w413 _]
                              frame False {
                                # "Start Monitor"
                                n288 = call "Start_PE7265.vi"("Lock-in Reference"=0, "VI-Pfad"=w413) -> ()
                              }
                              frame True {
                              }
                            }
                          }
                        }
                      }
                    }
                  }
                  frame #1 {
                    n289 = case shown="False" w415 {
                      tunnel: w414 -> [_ w416]
                      frame False {
                      }
                      frame True {
                        n290 = stacked-sequence {
                          seq-local: [w419 _] -> [_ w420]
                          seq-local: [w417 _] -> [_ w421]
                          tunnel: w416 -> [w419 _]
                          frame #0 {
                            n291 = global read "Data_Display_global.vi" "Lock-In-Running-Cluster"() -> (w418:T43)
                            n292 = Unbundle By Name(w418) -> ("zurich_Lock_in-running"=w417:bool)
                          }
                          frame #1 {
                            n293 = case shown="False" w421 {
                              tunnel: w420 -> [w422 _]
                              frame False {
                                # "Start Monitor"
                                n294 = call "Start_PE7265.vi"("Lock-in Reference"=1, "VI-Pfad"=w422) -> ()
                              }
                              frame True {
                              }
                            }
                          }
                        }
                      }
                    }
                  }
                  frame #2 {
                    n295 = case shown="True" w425 {
                      tunnel: w424 -> [_ w426]
                      frame False {
                      }
                      frame True {
                        n296 = stacked-sequence {
                          seq-local: [w429 _] -> [_ w430]
                          seq-local: [w427 _] -> [_ w431]
                          tunnel: w426 -> [w429 _]
                          frame #0 {
                            n297 = global read "Data_Display_global.vi" "Lock-In-Running-Cluster"() -> (w428:T43)
                            n298 = Unbundle By Name(w428) -> ("zurich_Lock_in-running"=w427:bool)
                          }
                          frame #1 {
                            n299 = case shown="False" w431 {
                              tunnel: w430 -> [w432 _]
                              frame False {
                                # "Start Monitor"
                                n300 = call "Start_PE7265.vi"("Lock-in Reference"=2, "VI-Pfad"=w432) -> ()
                              }
                              frame True {
                              }
                            }
                          }
                        }
                      }
                    }
                  }
                }
              }
              frame #16 {
                # "Keithley 2182A"
                n301 = global read "Instrument_Setup.vi" "Keithley 2182A"() -> (w435:bool)
                n302 = case shown="True" w435 {
                  tunnel: w434 -> [_ w436]
                  frame False {
                  }
                  frame True {
                    n303 = stacked-sequence {
                      seq-local: [w438 _] -> [_ w442]
                      seq-local: [w440 _] -> [_ w441]
                      tunnel: w436 -> [w437 _]
                      frame #0 {
                        n304 = Build Path(base path=w437, name or relative path="sub_vi-s\\Monitors\\Equipment\\Keithley2182AMonitor.vi") -> (appended path=w438:path)
                        n305 = call "Check_if_running.vi"("VI-Pfad"=w438) -> ("Running"=w440:bool)
                      }
                      frame #1 {
                        n306 = case shown="False" w441 {
                          tunnel: w442 -> [w443 _]
                          frame False {
                            # "Start Monitor"
                            n307 = call "Start_Vi.vi"("VI-Pfad"=w443) -> ()  [unwired: 1 in]
                          }
                          frame True {
                          }
                        }
                      }
                    }
                  }
                }
              }
              frame #17 {
                # "Keithley 2440"
                n308 = global read "Instrument_Setup.vi" "Keithley 2440"() -> (w445:bool)
                n309 = case shown="True" w445 {
                  tunnel: w444 -> [_ w446]
                  frame False {
                  }
                  frame True {
                    n310 = stacked-sequence {
                      seq-local: [w448 _] -> [_ w452]
                      seq-local: [w450 _] -> [_ w451]
                      tunnel: [w450 _] -> _
                      tunnel: w446 -> [w447 _]
                      frame #0 {
                        w449 = "sub_vi-s\\Monitors\\Equipment\\\nKeithleyMonitor.vi"  # sub_vi-s\Monitors\Equipment\ KeithleyMonitor.vi
                        # "Check if running"
                        n311 = Build Path(base path=w447, name or relative path=w449) -> (appended path=w448:path)
                        n312 = call "Check_if_running.vi"("VI-Pfad"=w448) -> ("Running"=w450:bool)
                      }
                      frame #1 {
                        n313 = case shown="False" w451 {
                          tunnel: w452 -> [w453 _]
                          frame False {
                            # "Start Monitor"
                            n314 = call "Start_Vi.vi"("VI-Pfad"=w453) -> ()  [unwired: 1 in]
                          }
                          frame True {
                          }
                        }
                      }
                    }
                  }
                }
              }
              frame #18 {
                # "Torque Motor"
                n315 = global read "Instrument_Setup.vi" "Torque \nMeasurem."() -> (w455:bool)
                n316 = case shown="True" w455 {
                  tunnel: w454 -> [_ w456]
                  frame False {
                  }
                  frame True {
                    n317 = stacked-sequence {
                      seq-local: [w458 _] -> [_ w462]
                      seq-local: [w460 _] -> [_ w461]
                      tunnel: w456 -> [w457 _]
                      frame #0 {
                        n318 = Build Path(base path=w457, name or relative path="sub_vi-s\\Monitors\\Equipment\\TMCMonitor.vi") -> (appended path=w458:path)
                        n319 = call "Check_if_running.vi"("VI-Pfad"=w458) -> ("Running"=w460:bool)
                      }
                      frame #1 {
                        n320 = case shown="False" w461 {
                          tunnel: w462 -> [w463 _]
                          frame False {
                            # "Start Monitor"
                            n321 = call "Start_Vi.vi"("VI-Pfad"=w463) -> ()  [unwired: 1 in]
                          }
                          frame True {
                          }
                        }
                      }
                    }
                  }
                }
              }
              frame #19 {
                # "Keithley 6221"
                n322 = global read "Instrument_Setup.vi" "Keithley 6221"() -> (w465:bool)
                n323 = case shown="True" w465 {
                  tunnel: w464 -> [_ w466]
                  frame False {
                  }
                  frame True {
                    n324 = stacked-sequence {
                      seq-local: [w467 _] -> [_ w472]
                      seq-local: [w470 _] -> [_ w471]
                      tunnel: w466 -> [w468 _]
                      frame #0 {
                        # "Check if running"
                        n325 = Build Path(base path=w468, name or relative path="sub_vi-s\\Monitors\\Equipment\\Keithley6221Monitor.vi") -> (appended path=w467:path)
                        n326 = call "Check_if_running.vi"("VI-Pfad"=w467) -> ("Running"=w470:bool)
                      }
                      frame #1 {
                        n327 = case shown="False" w471 {
                          tunnel: w472 -> [w473 _]
                          frame False {
                            # "Start Monitor"
                            n328 = call "Start_Vi.vi"("VI-Pfad"=w473) -> ()  [unwired: 1 in]
                          }
                          frame True {
                          }
                        }
                      }
                    }
                  }
                }
              }
              frame #20 {
                # "Picowatt AVS47"
                n329 = global read "Instrument_Setup.vi" "Picowatt AVS47"() -> (w475:bool)
                n330 = case shown="True" w475 {
                  tunnel: w474 -> [_ w476]
                  frame False {
                  }
                  frame True {
                    n331 = stacked-sequence {
                      seq-local: [w479 _] -> [_ w481]
                      seq-local: [w478 _] -> [_ w482]
                      tunnel: w476 -> [w480 _]
                      frame #0 {
                        # "Check if running"
                        n332 = Build Path(base path=w480, name or relative path="sub_vi-s\\Monitors\\Equipment\\PicowattAVS47Monitor.vi") -> (appended path=w479:path)
                        n333 = call "Check_if_running.vi"("VI-Pfad"=w479) -> ("Running"=w478:bool)
                      }
                      frame #1 {
                        n334 = case shown="False" w482 {
                          tunnel: w481 -> [w483 _]
                          frame False {
                            # "Start Monitor"
                            n335 = call "Start_Vi.vi"("VI-Pfad"=w483) -> ()  [unwired: 1 in]
                          }
                          frame True {
                          }
                        }
                      }
                    }
                  }
                }
              }
              frame #21 {
                # "Levelmeter"
                n336 = global read "Instrument_Setup.vi" "Instrument"() -> (w484:string)
                n337 = case shown="\"20T\"" w484 {
                  tunnel: w485 -> [_ w486 w496 _ w504 _]
                  frame "None" {
                  }
                  frame "Sweet 16", Default {
                    n338 = stacked-sequence {
                      seq-local: [w488 _] -> [_ w494]
                      seq-local: [w491 _] -> [_ w493]
                      tunnel: w486 -> [w489 _]
                      frame #0 {
                        n339 = global read "Instrument_Setup.vi" "Instrument"() -> (w487:string)
                        n340 = case shown="\"Sweet 16\", Default" w487 {
                          tunnel: [w492] -> w490
                          frame "Sweet 16", Default {
                            w492 = "sub_vi-s\\Monitors\\Instrument\\16TILMMonitor.vi"  # sub_vi-s\Monitors\Instrument\16TILMMonitor.vi
                          }
                        }
                        n341 = Build Path(base path=w489, name or relative path=w490) -> (appended path=w488:path)
                        n342 = call "Check_if_running.vi"("VI-Pfad"=w488) -> ("Running"=w491:bool)
                      }
                      frame #1 {
                        n343 = case shown="False" w493 {
                          tunnel: w494 -> [w495 _]
                          frame False {
                            # "Start Monitor"
                            n344 = call "Start_Vi.vi"("VI-Pfad"=w495) -> ()  [unwired: 1 in]
                          }
                          frame True {
                          }
                        }
                      }
                    }
                  }
                  frame "20T" {
                    n345 = stacked-sequence {
                      seq-local: [w498 _] -> [_ w502]
                      seq-local: [w500 _] -> [_ w501]
                      tunnel: w496 -> [w497 _]
                      frame #0 {
                        w499 = "sub_vi-s\\Monitors\\Instrument\\20TILMMonitor.vi"  # sub_vi-s\Monitors\Instrument\20TILMMonitor.vi
                        n346 = Build Path(base path=w497, name or relative path=w499) -> (appended path=w498:path)
                        n347 = call "Check_if_running.vi"("VI-Pfad"=w498) -> ("Running"=w500:bool)
                      }
                      frame #1 {
                        n348 = case shown="False" w501 {
                          tunnel: w502 -> [w503 _]
                          frame False {
                            # "Start Monitor"
                            n349 = call "Start_Vi.vi"("VI-Pfad"=w503) -> ()  [unwired: 1 in]
                          }
                          frame True {
                          }
                        }
                      }
                    }
                  }
                  frame "Berta" {
                  }
                  frame "Mischer" {
                    n350 = stacked-sequence {
                      seq-local: [w507 _] -> [_ w509]
                      seq-local: [w506 _] -> [_ w510]
                      tunnel: w504 -> [w508 _]
                      frame #0 {
                        w505 = "sub_vi-s\\Monitors\\Instrument\\Mischer_LevelmeterMonitor.vi"  # sub_vi-s\Monitors\Instrument\Mischer_LevelmeterMonitor.vi
                        n351 = Build Path(base path=w508, name or relative path=w505) -> (appended path=w507:path)
                        n352 = call "Check_if_running.vi"("VI-Pfad"=w507) -> ("Running"=w506:bool)
                      }
                      frame #1 {
                        n353 = case shown="False" w510 {
                          tunnel: w509 -> [w511 _]
                          frame False {
                            # "Start Monitor"
                            n354 = call "Start_Vi.vi"("VI-Pfad"=w511) -> ()  [unwired: 1 in]
                          }
                          frame True {
                          }
                        }
                      }
                    }
                  }
                  frame "PPMS" {
                  }
                }
              }
              frame #22 {
                # "Mischer Monitor"
                n355 = global read "Instrument_Setup.vi" "Instrument"() -> (w513:string)
                n356 = case shown="\"Mischer\"" w513 {
                  tunnel: w512 -> [_ w514]
                  frame "Sweet 16", Default {
                  }
                  frame "Mischer" {
                    n357 = stacked-sequence {
                      seq-local: [w517 _] -> [_ w519]
                      seq-local: [w516 _] -> [_ w520]
                      tunnel: w514 -> [w518 _]
                      frame #0 {
                        w515 = "sub_vi-s\\Monitors\\Instrument\\MischerMonitor.vi"  # sub_vi-s\Monitors\Instrument\MischerMonitor.vi
                        n358 = Build Path(base path=w518, name or relative path=w515) -> (appended path=w517:path)
                        n359 = call "Check_if_running.vi"("VI-Pfad"=w517) -> ("Running"=w516:bool)
                      }
                      frame #1 {
                        n360 = case shown="False" w520 {
                          tunnel: w519 -> [w521 _]
                          frame False {
                            # "Start Monitor"
                            n361 = call "Start_Vi.vi"("VI-Pfad"=w521) -> ()  [unwired: 1 in]
                          }
                          frame True {
                          }
                        }
                      }
                    }
                  }
                }
              }
              frame #23 {
                # "VCM Monitor"
                n362 = global read "Instrument_Setup.vi" "Instrument"() -> (w523:string)
                n363 = case shown="\"Mischer\"" w523 {
                  tunnel: w522 -> [_ w525]
                  frame "Sweet 16", Default {
                  }
                  frame "Mischer" {
                    n364 = global read "Instrument_Setup.vi" "VCM"() -> (w524:bool)
                    n365 = case shown="True" w524 {
                      tunnel: w525 -> [_ w526]
                      frame False {
                      }
                      frame True {
                        n366 = stacked-sequence {
                          seq-local: [w528 _] -> [_ w531]
                          seq-local: [w527 _] -> [_ w532]
                          tunnel: w526 -> [w530 _]
                          frame #0 {
                            w529 = "sub_vi-s\\Monitors\\Equipment\\VCM_ControlMonitor.vi"  # sub_vi-s\Monitors\Equipment\VCM_ControlMonitor.vi
                            n367 = Build Path(base path=w530, name or relative path=w529) -> (appended path=w528:path)
                            n368 = call "Check_if_running.vi"("VI-Pfad"=w528) -> ("Running"=w527:bool)
                          }
                          frame #1 {
                            n369 = case shown="False" w532 {
                              tunnel: w531 -> [w533 _]
                              frame False {
                                n370 = call "Start_Vi.vi"("VI-Pfad"=w533) -> ()  [unwired: 1 in]
                              }
                              frame True {
                              }
                            }
                          }
                        }
                      }
                    }
                  }
                }
              }
              frame #24 {
                # "Magnetic Field Monitors"
                n371 = global read "Instrument_Setup.vi" "Magnet"() -> (w534:bool)
                n372 = case shown="True" w534 {
                  tunnel: w535 -> [_ w536]
                  frame False {
                  }
                  frame True {
                    n373 = stacked-sequence {
                      seq-local: [w539 _] -> [_ w549]
                      seq-local: [w537 _] -> [_ w548]
                      tunnel: w536 -> [w540 _]
                      frame #0 {
                        n374 = global read "Instrument_Setup.vi" "Instrument"() -> (w538:string)
                        n375 = case shown="\"20T\"" w538 {
                          tunnel: ["sub_vi-s\\Monitors\\Instrument\\5TMonitor.vi" "sub_vi-s\\Monitors\\Instrument\\15TMonitor.vi" "sub_vi-s\\Monitors\\Instrument\\16TMonitor.vi" "sub_vi-s\\Monitors\\Instrument\\AMIMonitor.vi" "sub_vi-s\\Monitors\\Instrument\\20TMonitor.vi" "sub_vi-s\\Monitors\\Instrument\\P9MagnetMonitor.vi"] -> w541
                          frame "Mischer" {
                          }
                          frame "Berta" {
                          }
                          frame "Sweet 16", Default {
                          }
                          frame "AMI" {
                          }
                          frame "20T" {
                          }
                          frame "PPMS" {
                          }
                        }
                        n376 = Build Path(base path=w540, name or relative path=w541) -> (appended path=w539:path)
                        n377 = call "Check_if_running.vi"("VI-Pfad"=w539) -> ("Running"=w537:bool)
                      }
                      frame #1 {
                        n378 = case shown="False" w548 {
                          tunnel: w549 -> [w550 _]
                          frame False {
                            # "Start Monitor"
                            n379 = call "Start_Vi.vi"("VI-Pfad"=w550) -> ()  [unwired: 1 in]
                          }
                          frame True {
                          }
                        }
                      }
                    }
                  }
                }
              }
              frame #25 {
                # "Insert Monitor"
                n380 = global read "Instrument_Setup.vi" "Insert"() -> (w551:string)
                n381 = case shown="\"True\", Default" w551 {
                  tunnel: w551 -> [w553 _]
                  tunnel: w552 -> [w554 _]
                  frame "True", Default {
                    n382 = stacked-sequence {
                      seq-local: [w558 _] -> [_ w565]
                      seq-local: [w559 _] -> [_ w564]
                      tunnel: w554 -> [w557 _]
                      tunnel: w553 -> [w555 _]
                      frame #0 {
                        n383 = case shown="\"Kelvinox\"" w555 {
                          tunnel: ["sub_vi-s\\Monitors\\Insert\\16TVTIMonitor.vi" "sub_vi-s\\Monitors\\Insert\\20TVTIMonitor.vi" "sub_vi-s\\Monitors\\Insert\\JTMonitor.vi" "sub_vi-s\\Monitors\\Insert\\KelvinoxMonitor.vi"] -> w556
                          frame "VTI", Default {
                          }
                          frame "20TVTI" {
                            # "Check if running"
                          }
                          frame "JT" {
                          }
                          frame "Kelvinox" {
                          }
                        }
                        n384 = Build Path(base path=w557, name or relative path=w556) -> (appended path=w558:path)
                        n385 = call "Check_if_running.vi"("VI-Pfad"=w558) -> ("Running"=w559:bool)
                      }
                      frame #1 {
                        n386 = case shown="False" w564 {
                          tunnel: w565 -> [w566 _]
                          frame False {
                            # "Start Monitor"
                            n387 = call "Start_Vi.vi"("VI-Pfad"=w566) -> ()  [unwired: 1 in]
                          }
                          frame True {
                          }
                        }
                      }
                    }
                  }
                  frame "None" {
                  }
                }
              }
              frame #26 {
                # "Dewar Monitor"
                n388 = global read "Instrument_Setup.vi" "Instrument"() -> (w568:string)
                n389 = case shown="\"20T\"" w568 {
                  tunnel: w567 -> [w569 _]
                  frame "20T" {
                    n390 = stacked-sequence {
                      seq-local: [w572 _] -> [_ w575]
                      seq-local: [w573 _] -> [_ w574]
                      tunnel: w569 -> [w571 _]
                      frame #0 {
                        # "Check if running"
                        n391 = Build Path(base path=w571, name or relative path="sub_vi-s\\Monitors\\Instrument\\20TDewarMonitor.vi") -> (appended path=w572:path)
                        n392 = call "Check_if_running.vi"("VI-Pfad"=w572) -> ("Running"=w573:bool)
                      }
                      frame #1 {
                        n393 = case shown="False" w574 {
                          tunnel: w575 -> [w576 _]
                          frame False {
                            # "Start Monitor"
                            n394 = call "Start_Vi.vi"("VI-Pfad"=w576) -> ()  [unwired: 1 in]
                          }
                          frame True {
                          }
                        }
                      }
                    }
                  }
                  frame "None", Default {
                  }
                }
              }
              frame #27 {
                # "If the monitors are stopped during measurement \n, this is the case if LS370 is used with VTI option,\nthey will be restarted in the next cycle"
                n395 = global write "Data_Display_global.vi" "Stop Monitors"(FALSE) -> ()
              }
            }
          }
          frame #2 {
            # "Handle Measurement Skript"
            n396 = Less?(x=w578, y=1) -> (x < y?=w580:bool)
            n397 = case shown="False" w580 {
              frame False {
              }
              frame True {
                n398 = Wait (ms)(milliseconds to wait=3000) -> ()  [unwired: 1 out]
              }
            }
            n399 = call <vilib>:"Application Directory.vi"() -> ("Application Directory"=w581:path)
            n400 = case shown="True" TRUE {
              tunnel: w581 -> [_ w584]
              frame False {
              }
              frame True {
                n401 = stacked-sequence {
                  seq-local: [_ w599 _ _ _ _ _ _] -> [_ _ w625 w638 w646 _ _ _]
                  seq-local: [w586 _ _ _ _ _ _ _] -> [_ w599 _ _ _ _ _ _]
                  tunnel: w584 -> [w587 _ _ _ _ _ _ _]
                  frame #0 {
                    w588 = "sub_vi-s\\Global\\Main.vi"  # sub_vi-s\Global\Main.vi
                    # "Check if Main is running"
                    n402 = vi-ref "Main.vi"() -> (w594:refnum<vi>)
                    n403 = Build Path(base path=w587, name or relative path=w588) -> (appended path=w586:path)
                    n404 = Open VI Reference(type specifier VI Refnum (for type only)=w594, vi path=w586) -> (vi reference=w595:refnum<vi>, error out=w598:errorcluster)  [unwired: 4 in]
                    n405 = property class="VI"(reference=w595, error in=w598) -> (reference out=w597:refnum<vi>, error out=w596:errorcluster, "Exec.State"=w589:T39)
                    n406 = Equal?(x=T39."Run top level" ("LS 370 Monitor 2"), y=w589) -> (x = y?=w590:bool)
                    n407 = Close Reference(reference=w597, error in (no error)=w596) -> ()  [unwired: 1 out]
                    n408 = Equal?(x=T39."Running" ("LS 370 Monitor 2"), y=w589) -> (x = y?=w592:bool)
                    n409 = Or(x=w592, y=w590) -> (x .or. y?=w585:bool)
                    n410 = local write "Measurement"(w585) -> ()
                    n411 = global write "global.vi" "Measurement Running?"(w585) -> ()
                  }
                  frame #1 {
                    n412 = stacked-sequence {
                      seq-local: [w601 _] -> [_ w608]
                      tunnel: w599 -> [w600 _]
                      frame #0 {
                        (unwired) 13816530 ("Numerisch")
                        # "Check if Main is paused"
                        n413 = vi-ref "Main.vi"() -> (w602:refnum<vi>)
                        n414 = Open VI Reference(type specifier VI Refnum (for type only)=w602, vi path=w600) -> (vi reference=w603:refnum<vi>, error out=w606:errorcluster)  [unwired: 4 in]
                        n415 = property class="VI"(reference=w603, error in=w606) -> (reference out=w605:refnum<vi>, error out=w604:errorcluster, "Is VI Paused?"=w601:bool)
                        n416 = Close Reference(reference=w605, error in (no error)=w604) -> ()  [unwired: 1 out]
                      }
                      frame #1 {
                        n417 = local read "Measurement"() -> (w609:bool)
                        n418 = case shown="False" w608 {
                          tunnel: [w613 w620] -> w607
                          tunnel: [w611 w618] -> w610
                          tunnel: w609 -> [w612 w619]
                          frame False {
                            n419 = case shown="False" w612 {
                              tunnel: ["Stopped" "Running"] -> w613
                              tunnel: [13816530 7797099] -> w611
                              frame False {
                              }
                              frame True {
                              }
                            }
                          }
                          frame True {
                            n420 = case shown="True" w619 {
                              tunnel: ["Stopped" "Paused"] -> w620
                              tunnel: [14671839 16737792] -> w618
                              frame False {
                              }
                              frame True {
                              }
                            }
                          }
                        }
                        "Current Measurement" <- w607
                        n421 = property on="Current Measurement" class="Str"("Text.BGColor"=w610, "Text.BGColor"=w610) -> ()  [unwired: 2 in, 2 out]
                      }
                    }
                  }
                  frame #2 {
                    n422 = case shown="True" "Start" {
                      tunnel: w625 -> [_ w627]
                      frame False {
                      }
                      frame True {
                        n423 = vi-ref "Main.vi"() -> (w629:refnum<vi>)
                        n424 = Open VI Reference ("VI-Referenz öffnen")(type specifier VI Refnum (for type only)=w629, vi path=w627) -> (vi reference=w633:refnum<vi>, error out=w632:errorcluster)  [unwired: 4 in]
                        n425 = invoke class="VI" method="Run VI"(reference=w633, error in=w632, "Wait until done"=FALSE) -> (reference out=w628:refnum<vi>, error out=w631:errorcluster)  [unwired: 2 in, 3 out]
                        n426 = Close Reference(reference=w628, error in (no error)=w631) -> (error out=w634:errorcluster)
                        n427 = call <vilib>:"General Error Handler.vi"("error in (no error)"=w634) -> ()  [unwired: 10 in, 5 out]
                      }
                    }
                  }
                  frame #3 {
                    n428 = local read "Stop Main"() -> (w636:bool)
                    n429 = Or(x="Stop", y=w636) -> (x .or. y?=w635:bool)
                    n430 = case shown="True" w635 {
                      tunnel: w638 -> [_ w639]
                      frame False {
                      }
                      frame True {
                        n431 = vi-ref "Main.vi"() -> (w642:refnum<vi>)
                        n432 = Open VI Reference ("VI-Referenz öffnen")(type specifier VI Refnum (for type only)=w642, vi path=w639) -> (vi reference=w645:refnum<vi>, error out=w644:errorcluster)  [unwired: 4 in]
                        n433 = invoke class="VI" method="Abort VI"(reference=w645, error in=w644) -> (reference out=w643:refnum<vi>, error out=w641:errorcluster)  [unwired: 1 in, 1 out]
                        n434 = Close Reference(reference=w643, error in (no error)=w641) -> (error out=w640:errorcluster)
                        n435 = call <vilib>:"General Error Handler.vi"("error in (no error)"=w640) -> ()  [unwired: 10 in, 5 out]
                      }
                    }
                  }
                  frame #4 {
                    n436 = case shown="True" "Pause" {
                      tunnel: w646 -> [_ w649]
                      frame False {
                      }
                      frame True {
                        n437 = vi-ref "Main.vi"() -> (w650:refnum<vi>)
                        n438 = Open VI Reference ("VI-Referenz öffnen")(type specifier VI Refnum (for type only)=w650, vi path=w649) -> (vi reference=w648:refnum<vi>, error out=w654:errorcluster)  [unwired: 4 in]
                        n439 = invoke class="VI" method="PauseVI"(reference=w648, error in=w654) -> (reference out=w653:refnum<vi>, error out=w652:errorcluster)  [unwired: 1 in, 1 out]
                        n440 = Close Reference(reference=w653, error in (no error)=w652) -> (error out=w651:errorcluster)
                        n441 = call <vilib>:"General Error Handler.vi"("error in (no error)"=w651) -> ()  [unwired: 10 in, 5 out]
                      }
                    }
                  }
                  frame #5 {
                    n442 = local read "Measurement"() -> (w661:bool)
                    n443 = case shown="True" w661 {
                      tunnel: [w667 w678] -> w666
                      tunnel: [w667 w677] -> w662
                      tunnel: [w667 w676] -> w663
                      tunnel: [w667 w675] -> w664
                      tunnel: [w667 w674] -> w665
                      tunnel: [w667 w673] -> w660
                      tunnel: [w667 w670] -> w659
                      tunnel: [w667 w672] -> w658
                      tunnel: [w667 w671] -> w657
                      tunnel: [w667 w669] -> w656
                      tunnel: [w667 w668] -> w655
                      frame False {
                        w667 = 0.0
                      }
                      frame True {
                        n444 = global read "Data_Display_global.vi" "current number of steps"() -> (w671:i32)
                        n445 = global read "Data_Display_global.vi" "waiting time"() -> (w670:dbl)
                        n446 = global read "Data_Display_global.vi" "CC running time"() -> (w673:dbl)
                        n447 = global read "global.vi" "-ter Messungsreihe"() -> (w678:dbl)
                        n448 = global read "global.vi" "Sweep final rate"() -> (w668:dbl)
                        n449 = global read "global.vi" "Sweep init rate"() -> (w669:dbl)
                        n450 = global read "global.vi" "Sweep init"() -> (w675:dbl)
                        n451 = global read "global.vi" "phi_final"() -> (w672:dbl)
                        n452 = global read "global.vi" "Sweep final"() -> (w674:dbl)
                        n453 = global read "global.vi" "H init.(T)"() -> (w677:dbl)
                        n454 = global read "global.vi" "T init. (K)"() -> (w676:dbl)
                      }
                    }
                    "Init" <- w664
                    "Final" <- w665
                    "B (T)" <- w662
                    "T (K)" <- w663
                    "Row" <- w666
                    "Waiting time" <- w659
                    "CC Running time" <- w660
                    "Phi (Deg)" <- w658
                    "Step #" <- w657
                    "Final rate" <- w655
                    "Init rate" <- w656
                  }
                  frame #6 {
                    n455 = local read "Measurement"() -> (w679:bool)
                    n456 = case shown="True" w679 {
                      tunnel: ["" w685] -> w680
                      frame False {
                        w681 = 13816530 ("Numerisch")
                        n457 = property on="Sweep Type" class="Str"("Text.BGColor"=w681, "Text.BG Color"=w681) -> ()  [unwired: 2 in, 2 out]
                      }
                      frame True {
                        n458 = global read "global.vi" "Sweep Type"() -> (w684:string)
                        n459 = global read "global.vi" "Cerrent State"() -> (w690:i32)
                        n460 = Equal?(x=1, y=w690) -> (x = y?=w688:bool)
                        n461 = case shown="True" w688 {
                          tunnel: ["" "Initalize"] -> w687
                          tunnel: [7797099 16737792] -> w686
                          frame False {
                          }
                          frame True {
                          }
                        }
                        n462 = Concatenate Strings(w687, "\r\n", w684) -> (w685:string)
                        n463 = property on="Sweep Type" class="Str"("Text.BGColor"=w686, "Text.BG Color"=w686) -> ()  [unwired: 2 in, 2 out]
                      }
                    }
                    "Sweep Type" <- w680
                  }
                  frame #7 {
                    n464 = global read "Data_Display_global.vi" "Remaining Duration of rows"() -> (→"Remaining time of rows":string)
                    n465 = global read "Data_Display_global.vi" "End of measurement"() -> (w699:timestamp)
                    n466 = Format Date/Time String(time format string (%c)="%c", seconds (now)=w699) -> (date/time string=→"End of measurement":string)  [unwired: 1 in]
                    n467 = Get Date/Time In Seconds() -> (seconds since 1Jan1904=w698:timestamp)
                    n468 = Subtract(x=w699, y=w698) -> (x-y=w696:dbl)
                    n469 = Format Into String(format string="%<%Dd %Hh:%Mm:%Ss>t", w696) -> (resulting string=→"Remaining time":string)  [unwired: 2 in, 1 out]
                  }
                }
              }
            }
          }
          frame #3 {
            w756 = string[] ["empty", "SR830-1", "SR830-2", "ILM", "20TILM", "AH2700", "K6221", "Plot3", "20T-Dewar", "SR830-3", "PE7265", "MischerMonitor", "MischerLevelmeter", "LS370 Readout", "LS372 Readout", "LIA7230-1", "LIA7230-2", "LIA7230-3", "K2182A", "TMC Monitor", "zurich_Lock_in", "SIM921"]
            # "Customize Plot Panels"
            n470 = property on="Panel 1" class="Ring (strict)"("Strings []"=w756) -> (error out=w776:errorcluster)  [unwired: 2 in, 1 out]
            n471 = property on="Panel 2" class="Ring (strict)"("Strings []"=w756) -> ()  [unwired: 2 in, 2 out]
            n472 = property on="Panel 3" class="Ring (strict)"("Strings []"=w756) -> ()  [unwired: 2 in, 2 out]
            n473 = property on="Panel 4" class="Ring (strict)"("Strings []"=w756) -> ()  [unwired: 2 in, 2 out]
            n474 = property on="Panel 5" class="Ring (strict)"("Strings []"=w756) -> ()  [unwired: 2 in, 2 out]
            n475 = property on="Panel 6" class="Ring (strict)"("Strings []"=w756) -> ()  [unwired: 2 in, 2 out]
            n476 = property on="Panel 1" class="Ring (strict)"(error in=w776) -> ("RingText.Text"=w800:string)  [unwired: 1 in, 2 out]
            n477 = property on="Panel 2" class="Ring (strict)"() -> ("RingText.Text"=w799:string)  [unwired: 2 in, 2 out]
            n478 = property on="Panel 3" class="Ring (strict)"() -> ("RingText.Text"=w798:string)  [unwired: 2 in, 2 out]
            n479 = property on="Panel 4" class="Ring (strict)"() -> ("RingText.Text"=w797:string)  [unwired: 2 in, 2 out]
            n480 = property on="Panel 5" class="Ring (strict)"() -> ("RingText.Text"=w796:string)  [unwired: 2 in, 2 out]
            n481 = property on="Panel 6" class="Ring (strict)"() -> ("RingText.Text"=w795:string)  [unwired: 2 in, 2 out]
            n482 = Build Array(w800, w799, w798, w797, w796, w795) -> (w794:string[])
            n483 = call "Choose_Panels.vi"("Array"=w794) -> ("Array 2"=w707:string[])  [unwired: 10 in]
            n484 = call "Activate_Panel.vi"("Panel Name"="20TILM", "Panel Array"=w707) -> ("Top"=w740:i32, "Left"=w741:i32, "Active"=w742:bool)
            n485 = call "Activate_Panel.vi"("Panel Name"="SR830-1", "Panel Array"=w707) -> ("Top"=w777:i32, "Left"=w778:i32, "Active"=w779:bool)
            n486 = call "Activate_Panel.vi"("Panel Name"="SR830-2", "Panel Array"=w707) -> ("Top"=w780:i32, "Left"=w781:i32, "Active"=w782:bool)
            n487 = call "Activate_Panel.vi"("Panel Name"="AH2700", "Panel Array"=w707) -> ("Top"=w786:i32, "Left"=w787:i32, "Active"=w788:bool)
            n488 = call "Activate_Panel.vi"("Panel Name"="ILM", "Panel Array"=w707) -> ("Top"=w783:i32, "Left"=w784:i32, "Active"=w785:bool)
            n489 = call "Activate_Panel.vi"("Panel Name"="K6221", "Panel Array"=w707) -> ("Top"=w763:i32, "Left"=w762:i32, "Active"=w761:bool)
            n490 = call "Activate_Panel.vi"("Panel Name"="MischerMonitor", "Panel Array"=w707) -> ("Top"=w750:i32, "Left"=w749:i32, "Active"=w748:bool)
            n491 = property on="20TILM" class="Clust (strict)"("Top"=w740, "Left"=w741, "Visible"=w742) -> ()  [unwired: 2 in, 2 out]
            n492 = property on="SR830-1" class="Clust (strict)"("Top"=w777, "Left"=w778, "Visible"=w779) -> ()  [unwired: 2 in, 2 out]
            n493 = property on="SR830-2" class="Clust (strict)"("Top"=w780, "Left"=w781, "Visible"=w782) -> ()  [unwired: 2 in, 2 out]
            n494 = property on="ILM" class="Clust (strict)"("Top"=w783, "Left"=w784, "Visible"=w785) -> ()  [unwired: 2 in, 2 out]
            n495 = property on="AH 2700 Monitor" class="Clust (strict)"("Top"=w786, "Left"=w787, "Visible"=w788) -> ()  [unwired: 2 in, 2 out]
            n496 = property on="K6221" class="Clust (strict)"("Top"=w763, "Left"=w762, "Visible"=w761) -> ()  [unwired: 2 in, 2 out]
            n497 = property on="Mischer Monitor" class="Clust (strict)"("Top"=w750, "Left"=w749, "Visible"=w748) -> ()  [unwired: 2 in, 2 out]
            n498 = call "Activate_Panel.vi"("Panel Name"="20T-Dewar", "Panel Array"=w707) -> ("Top"=w770:i32, "Left"=w769:i32, "Active"=w768:bool)
            n499 = call "Activate_Panel.vi"("Panel Name"="LS372 Readout", "Panel Array"=w707) -> ("Top"=w734:i32, "Left"=w733:i32, "Active"=w732:bool)
            n500 = call "Activate_Panel.vi"("Panel Name"="Plot 3", "Panel Array"=w707) -> ("Top"=w774:i32, "Left"=w773:i32, "Active"=w772:bool)
            n501 = call "Activate_Panel.vi"("Panel Name"="SR830-3", "Panel Array"=w707) -> ("Top"=w764:i32, "Left"=w765:i32, "Active"=w766:bool)
            n502 = call "Activate_Panel.vi"("Panel Name"="PE7265", "Panel Array"=w707) -> ("Top"=w759:i32, "Left"=w758:i32, "Active"=w757:bool)
            n503 = call "Activate_Panel.vi"("Panel Name"="MischerLevelmeter", "Panel Array"=w707) -> ("Top"=w754:i32, "Left"=w753:i32, "Active"=w752:bool)
            n504 = call "Activate_Panel.vi"("Panel Name"="LS370 Readout", "Panel Array"=w707) -> ("Top"=w738:i32, "Left"=w737:i32, "Active"=w736:bool)
            n505 = call "Activate_Panel.vi"("Panel Name"="AH2500", "Panel Array"=w707) -> ("Top"=w746:i32, "Left"=w745:i32, "Active"=w744:bool)
            n506 = property on="Plot 3" class="Clust (strict)"("Top"=w774, "Left"=w773, "Visible"=w772) -> ()  [unwired: 2 in, 2 out]
            n507 = property on="20T-Dewar-Cluster" class="Clust (strict)"("Top"=w770, "Left"=w769, "Visible"=w768) -> ()  [unwired: 2 in, 2 out]
            n508 = property on="SR830-3" class="Clust (strict)"("Top"=w764, "Left"=w765, "Visible"=w766) -> ()  [unwired: 2 in, 2 out]
            n509 = property on="PE7265-Cluster" class="Clust (strict)"("Top"=w759, "Left"=w758, "Visible"=w757) -> ()  [unwired: 2 in, 2 out]
            n510 = property on="LS372_Readout-Monitor" class="Clust (strict)"("Top"=w734, "Left"=w733, "Visible"=w732) -> ()  [unwired: 2 in, 2 out]
            n511 = property on="Mischer Levelmeter" class="Clust (strict)"("Top"=w754, "Left"=w753, "Visible"=w752) -> ()  [unwired: 2 in, 2 out]
            n512 = property on="AH2500 Monitor" class="Clust (strict)"("Top"=w746, "Left"=w745, "Visible"=w744) -> ()  [unwired: 2 in, 2 out]
            n513 = property on="LS370_Readout-Monitor" class="Clust (strict)"("Top"=w738, "Left"=w737, "Visible"=w736) -> ()  [unwired: 2 in, 2 out]
            n514 = call "Activate_Panel.vi"("Panel Name"="LIA7230-1", "Panel Array"=w707) -> ("Top"=w730:i32, "Left"=w729:i32, "Active"=w728:bool)
            n515 = call "Activate_Panel.vi"("Panel Name"="LIA7230-3", "Panel Array"=w707) -> ("Top"=w722:i32, "Left"=w721:i32, "Active"=w720:bool)
            n516 = call "Activate_Panel.vi"("Panel Name"="K2182A", "Panel Array"=w707) -> ("Top"=w718:i32, "Left"=w717:i32, "Active"=w716:bool)
            n517 = call "Activate_Panel.vi"("Panel Name"="LIA7230-2", "Panel Array"=w707) -> ("Top"=w727:i32, "Left"=w726:i32, "Active"=w725:bool)
            n518 = call "Activate_Panel.vi"("Panel Name"="TMC Monitor", "Panel Array"=w707) -> ("Top"=w714:i32, "Left"=w713:i32, "Active"=w712:bool)
            n519 = property on="LIA7230-1" class="Clust (strict)"("Top"=w730, "Left"=w729, "Visible"=w728) -> ()  [unwired: 2 in, 2 out]
            n520 = call "Activate_Panel.vi"("Panel Name"="zurich_Lock_in", "Panel Array"=w707) -> ("Top"=w710:i32, "Left"=w709:i32, "Active"=w708:bool)
            n521 = call "Activate_Panel.vi"("Panel Name"="SIM921", "Panel Array"=w707) -> ("Top"=w705:i32, "Left"=w704:i32, "Active"=w703:bool)
            n522 = property on="LIA7230-2" class="Clust (strict)"("Top"=w727, "Left"=w726, "Visible"=w725) -> ()  [unwired: 2 in, 2 out]
            n523 = property on="LIA7230-3" class="Clust (strict)"("Top"=w722, "Left"=w721, "Visible"=w720) -> ()  [unwired: 2 in, 2 out]
            n524 = property on="TMC-Control" class="Clust (strict)"("Top"=w714, "Left"=w713, "Visible"=w712) -> ()  [unwired: 2 in, 2 out]
            n525 = property on="K2182A" class="Clust (strict)"("Top"=w718, "Left"=w717, "Visible"=w716) -> ()  [unwired: 2 in, 2 out]
            n526 = property on="Zurich-Lock-In Monitor" class="Clust (strict)"("Top"=w710, "Left"=w709, "Visible"=w708) -> ()  [unwired: 2 in, 2 out]
            n527 = property on="SIM921" class="Clust (strict)"("Top"=w705, "Left"=w704, "Visible"=w703) -> ()  [unwired: 2 in, 2 out]
          }
          frame #4 {
            # "Levelmeter Control / Lambda Controller"
            n528 = global read "Instrument_Setup.vi" "Instrument"() -> (w801:string)
            n529 = case shown="\"20T\"" w801 {
              tunnel: w803 -> [w805 w834 w839 w873 w885]
              tunnel: [w804 w834 w838 w872 w885] -> w802
              frame "Mischer" {
                n530 = stacked-sequence {
                  seq-local: [w814 _] -> [_ w830]
                  tunnel: w805 -> [w815 _]
                  tunnel: [_ w829] -> w804
                  frame #0 {
                    n531 = local read "Mischer Levelmeter"() -> (w820:T25)
                    n532 = global read "Data_Display_global.vi" "Mischer Levelmeter"() -> (w817:T25)
                    n533 = call "Levelmeter_Split_Cluster.vi"("Mischer Levelmeter"=w817) -> ("Mischer Levelmeter Status"=w816:T44)  [unwired: 1 out]
                    n534 = call "Levelmeter_Split_Cluster.vi"("Mischer Levelmeter"=w820) -> ("Mischer Levelmeter  Control"=w819:T45)  [unwired: 1 out]
                    n535 = call "Levelmeter_Open_Queue.vi"() -> ("queue out"=w821:refnum<queue>)  [unwired: 10 in, 1 out]
                    n536 = call "Levelmeter_Queue_Commands.vi"("Mischer Levelmeter  Control"=w819, "Mischer Levelmeter N"=w821) -> ("New Status"=w818:T45)  [unwired: 1 in]
                    n537 = call "Levelmeter_Merge_Cluster.vi"("Mischer Levelmeter  Control"=w818, "Mischer Levelmeter Status"=w816) -> ("Mischer Levelmeter"=w806:T25)
                    n538 = call "Levelmeter_Set_Monitor_Values.vi"("Mischer Levelmeter Status"=w816, "System Monitor Variables (in)"=w815) -> ("System Monitor Variables (out)"=w814:T37)  [unwired: 3 in]
                    n539 = Unbundle By Name(w814) -> ("H_Level"=w813:dbl[])
                    n540 = local write "Mischer Levelmeter"(w806) -> ()
                    n541 = Array Size(array=w813) -> (size(s)=w812:i32)
                    n542 = Decrement(x=w812) -> (x-1=w811:i32)
                    n543 = Index Array(array=w813, index=w811) -> (element=w810:dbl)
                    n544 = Less?(x=w810, y=5) -> (x < y?=w808:bool)
                    n545 = case shown="True" w808 {
                      tunnel: w808 -> [_ w823]
                      tunnel: "Oh shit, Helium below 5 %. Better fill" -> [_ w822]
                      frame False {
                      }
                      frame True {
                        n546 = Bundle By Name(cluster=errorcluster {"status"=FALSE, "code"=0, "source"=""} ("error constant"), "code"=999, "status"=w823, "source"=w822) -> (w825:errorcluster)
                        n547 = call "Error_handler.vi"("error constant"=w825) -> ()
                      }
                    }
                  }
                  frame #1 {
                    n548 = global read "Data_Display_global.vi" "Mischer Monitor"() -> (w828:T23)
                    n549 = local read "Mischer Monitor"() -> (w833:T23)
                    n550 = call "MischerMonitor_Split_Cluster.vi"("Mischer Monitor"=w833) -> ("Mischer  Control"=w832:T46)  [unwired: 1 out]
                    n551 = call "MischerMonitor_Split_Cluster.vi"("Mischer Monitor"=w828) -> ("Mischer  Status"=w831:T47)  [unwired: 1 out]
                    n552 = call "MischerMonitor_Merge_Cluster.vi"("Mischer  Control"=w832, "Mischer  Status"=w831) -> ("Mischer Monitor"=w827:T23)
                    n553 = call "MischerMonitor_set_Monitor_Values.vi"("Mischer  Status"=w831, "System Monitor Variables (in)"=w830) -> ("System Monitor Variables (out)"=w829:T37)  [unwired: 3 in]
                    n554 = global write "Data_Display_global.vi" "Mischer Monitor"(w827) -> ()
                    n555 = local write "Mischer Monitor"(w827) -> ()
                  }
                }
              }
              frame "Berta" {
              }
              frame "Sweet 16", Default {
                n556 = global read "Instrument_Setup.vi" "Instrument"() -> (w850:string)
                n557 = case shown="\"Sweet 16\", Default" w850 {
                  tunnel: [60 20] -> w851
                  tunnel: ["Oh shit, Helium below 60 %. Better fill" "Oh shit, Helium below 20 %. Better fill"] -> w849
                  frame "AMI" {
                  }
                  frame "Sweet 16", Default {
                  }
                }
                n558 = local read "ILM"() -> (w842:T33)
                n559 = global read "Data_Display_global.vi" "ILM"() -> (w847:T33)
                n560 = call-poly "Split_Cluster.vi"("SR830-2 2"=w842) -> ("SR830-2 3"=w846:T48)  [unwired: 1 out]
                n561 = call-poly "Open_Queue.vi"() -> ("queue out"=w844:refnum<queue>)  [unwired: 10 in, 1 out]
                n562 = call-poly "Queue_Commands.vi"("SR830-2 2"=w846, "20TVTI Queue"=w844) -> ("SR830-2 3"=w845:T48)  [unwired: 1 in]
                n563 = call-poly "Split_Cluster.vi"("SR830-2 2"=w847) -> ("SR830-2 4"=w843:T49)  [unwired: 1 out]
                n564 = call-poly "Merge_Cluster.vi"("SR830-2 3"=w845, "SR830-2 4"=w843) -> ("SR830-2 2"=w841:T33)
                n565 = call "ILM_Set_Monitor_Values.vi"("SR830-2 2"=w843, "System Monitor Variables (in)"=w839) -> ("System Monitor Variables (out)"=w838:T37)  [unwired: 3 in]
                n566 = local write "ILM"(w841) -> ()
                n567 = Unbundle By Name(w838) -> ("H_Level"=w837:dbl[])
                n568 = Array Size(array=w837) -> (size(s)=w835:i32)
                n569 = Decrement(x=w835) -> (x-1=w836:i32)
                n570 = Index Array(array=w837, index=w836) -> (element=w840:dbl)
                n571 = Less?(x=w840, y=w851) -> (x < y?=w848:bool)
                n572 = case shown="True" w848 {
                  tunnel: w848 -> [_ w855]
                  tunnel: w849 -> [_ w854]
                  frame False {
                  }
                  frame True {
                    n573 = Bundle By Name(cluster=errorcluster {"status"=FALSE, "code"=0, "source"=""} ("error constant"), "code"=999, "status"=w855, "source"=w854) -> (w853:errorcluster)
                    n574 = call "Error_handler.vi"("error constant"=w853) -> ()
                  }
                }
              }
              frame "20T" {
                # "-Inf happens during a connection error"
                n575 = local read "20TILM"() -> (w876:T15)
                n576 = global read "Data_Display_global.vi" "20TILM"() -> (w874:T15)
                n577 = call "20TILM_Split_Cluster.vi"("20TILM"=w876) -> ("20T Control"=w868:T50)  [unwired: 1 out]
                n578 = call-poly "Open_Queue.vi"() -> ("queue out"=w869:refnum<queue>)  [unwired: 10 in, 1 out]
                n579 = call "20TILM_Split_Cluster.vi"("20TILM"=w874) -> ("20TILM Status"=w867:T51)  [unwired: 1 out]
                n580 = call "20TILM_Queue_Commands.vi"("20TILM Control (in)"=w868, "ILM Queue"=w869) -> ("20TILM Control (out)"=w866:T50)
                n581 = call "20TILM_Set_Monitor_Values.vi"("20TILM Status"=w867, "System Monitor Variables (in)"=w873) -> ("System Monitor Variables (out)"=w872:T37)
                n582 = call "20TILM_Merge_Cluster.vi"("20TILM Control"=w866, "20TILM Status"=w867) -> ("20TILM Cluster"=w875:T15)
                n583 = Unbundle By Name(w872) -> ("H_Level"=w879:dbl[])
                n584 = local write "20TILM"(w875) -> ()
                n585 = Array Size(array=w879) -> (size(s)=w877:i32)
                n586 = Decrement(x=w877) -> (x-1=w878:i32)
                n587 = Index Array(array=w879, index=w878) -> (element=w865:dbl)
                n588 = Not Equal?(x=w865, y=-inf) -> (x != y?=w862:bool)
                n589 = Less?(x=w865, y=10) -> (x < y?=w863:bool)
                n590 = And(x=w863, y=w862) -> (x .and. y?=w861:bool)
                n591 = case shown="True" w861 {
                  tunnel: w861 -> [_ w883]
                  tunnel: "Oh shit, Helium below 10 %. Better fill!" -> [_ w882]
                  frame False {
                  }
                  frame True {
                    n592 = Bundle By Name(cluster=errorcluster {"status"=FALSE, "code"=0, "source"=""} ("error constant"), "code"=999, "status"=w883, "source"=w882) -> (w881:errorcluster)
                    n593 = call "Error_handler.vi"("error constant"=w881) -> ()
                  }
                }
              }
              frame "PPMS" {
              }
            }
          }
          frame #5 {
            # "Lambda Warning"
            # "Constantly Check Magnet Temperature if 16 T Mode is active"
            n594 = global read "Instrument_Setup.vi" "16T /20T"() -> (w886:bool)
            n595 = case shown="True" w886 {
              frame False {
                n596 = global read "Data_Display_global.vi" "Magnetic Field SC"() -> (w888:dbl)
                n597 = global read "Data_Display_global.vi" "Magnet T (K)"() -> (w892:dbl)
                n598 = Greater?(x=w892, y=4.4) -> (0:w887:bool)
                n599 = Not Equal To 0?(x=w888) -> (x != 0?=w889:bool)
                n600 = And(x=w889, y=w887) -> (x .and. y?=w890:bool)
                n601 = case shown="True" w890 {
                  frame False {
                    n602 = local write "Stop Main"(FALSE) -> ()
                    n603 = property on="Quench Danger" class="Bool (strict)"("Visible"=FALSE) -> ()  [unwired: 2 in, 2 out]
                  }
                  frame True {
                    w898 = TRUE
                    n604 = call <vilib>:"Application Directory.vi"() -> ("Application Directory"=w897:path)
                    n605 = Build Path(base path=w897, name or relative path="sub_vi-s\\Global\\Main.vi") -> (appended path=w895:path)
                    n606 = local write "Quench Danger"(w898) -> ()
                    n607 = call "Check_if_running.vi"("VI-Pfad"=w895) -> ("Running"=w899:bool)
                    n608 = case shown="False" w899 {
                      frame False {
                        n609 = local write "Stop Main"(FALSE) -> ()
                      }
                      frame True {
                        n610 = local write "Stop Main"(TRUE) -> ()
                      }
                    }
                    n611 = property on="Quench Danger" class="Bool (strict)"("Visible"=w898) -> ()  [unwired: 2 in, 2 out]
                  }
                }
              }
              frame True {
                n612 = global read "Instrument_Setup.vi" "Instrument"() -> (w908:string)
                n613 = global read "Data_Display_global.vi" "Magnet T (K)"() -> (w911:dbl)
                n614 = case shown="\"Sweet16\", Default" w908 {
                  tunnel: [14.0 18.0] -> w906
                  tunnel: [2.3 2.31] -> w904
                  frame "Sweet16", Default {
                  }
                  frame "20T" {
                  }
                }
                n615 = Greater?(x=w911, y=w904) -> (0:w910:bool)
                n616 = case shown="True" w910 {
                  tunnel: [FALSE w918] -> w903
                  tunnel: w904 -> [_ w917]
                  frame False {
                  }
                  frame True {
                    n617 = stacked-sequence {
                      tunnel: [_ w921] -> w918
                      tunnel: w917 -> [_ w920]
                      frame #0 {
                        n618 = Wait (ms)(milliseconds to wait=2000) -> ()  [unwired: 1 out]
                      }
                      frame #1 {
                        n619 = global read "Data_Display_global.vi" "Magnet T (K)"() -> (w922:dbl)
                        n620 = Greater?(x=w922, y=w920) -> (0:w921:bool)
                      }
                    }
                  }
                }
                n621 = global read "Data_Display_global.vi" "Magnetic Field SC"() -> (w909:dbl)
                n622 = Absolute Value(x=w909) -> (abs(x)=w907:dbl)
                n623 = Greater?(x=w907, y=w906) -> (0:w905:bool)
                n624 = And(x=w905, y=w903) -> (x .and. y?=w902:bool)
                n625 = case shown="True" w902 {
                  frame False {
                    n626 = property on="Quench Danger" class="Bool (strict)"("Visible"=FALSE) -> ()  [unwired: 2 in, 2 out]
                  }
                  frame True {
                    w928 = TRUE
                    n627 = call <vilib>:"Application Directory.vi"() -> ("Application Directory"=w927:path)
                    n628 = Build Path(base path=w927, name or relative path="sub_vi-s\\Global\\Main.vi") -> (appended path=w925:path)
                    n629 = global read "Instrument_Setup.vi" "Instrument"() -> (w924:string)
                    n630 = call "Check_if_running.vi"("VI-Pfad"=w925) -> ("Running"=w929:bool)
                    n631 = case shown="\"20T\"" w924 {
                      frame "Sweet16", Default {
                        # "TODO: Implement switching off magnet!"
                      }
                      frame "20T" {
                        n632 = global read "Data_Display_global.vi" "20 T Magnet control"() -> (w936:T3)
                        n633 = call-poly "Split_Cluster.vi"("20 T Cluster"=w936) -> ("20 T Control"=w934:T52)  [unwired: 1 out]
                        n634 = Bundle By Name(cluster=w934, "Field Setpoint (T)"=0.0, "Rate Setpoint (T/min)"=0.05, "Go to Zero"=TRUE, "Set Rate"=TRUE) -> (w935:T52)
                        n635 = call-poly "Open_Queue.vi"() -> ("queue out"=w937:refnum<queue>)  [unwired: 10 in, 1 out]
                        n636 = call-poly "Queue_Commands.vi"("20T Control (in)"=w935, "20T Queue"=w937) -> ()  [unwired: 1 in, 1 out]
                      }
                    }
                    n637 = property on="Quench Danger" class="Bool (strict)"("Visible"=w928) -> ()  [unwired: 2 in, 2 out]
                    n638 = case shown="True" w929 {
                      frame False {
                      }
                      frame True {
                        "Stop Main" <- TRUE
                      }
                    }
                    "Quench Danger" <- w928
                  }
                }
              }
            }
          }
          frame #6 {
            # "Select Display Values"
            n639 = case shown="True" TRUE {
              tunnel: w940 -> [_ w942]
              frame False {
              }
              frame True {
                n640 = call "Select_Value.vi"("Numerisch"="Temperature 6", "System Monitor Variables"=w942) -> ("Value"=→"T3-v 2":dbl)  [unwired: 1 in, 2 out]
                n641 = call "Select_Value.vi"("Numerisch"="Temperature 2", "System Monitor Variables"=w942) -> ("Value"=→"T2-v":dbl)  [unwired: 1 in, 2 out]
                n642 = call "Select_Value.vi"("Numerisch"="Temperature 5", "System Monitor Variables"=w942) -> ("Value"=→"T2-v 2":dbl)  [unwired: 1 in, 2 out]
                n643 = call "Select_Value.vi"("Numerisch"="Temperature 1", "System Monitor Variables"=w942) -> ("Value"=→"T1-v":dbl)  [unwired: 1 in, 2 out]
                n644 = call "Select_Value.vi"("Numerisch"="Temperature 3", "System Monitor Variables"=w942) -> ("Value"=→"T3-v":dbl)  [unwired: 1 in, 2 out]
                n645 = call "Select_Value.vi"("Numerisch"="Temperature 4", "System Monitor Variables"=w942) -> ("Value"=→"T1-v 2":dbl)  [unwired: 1 in, 2 out]
                n646 = property on="System Monitor Variables" class="Clust (strict)"() -> ("Controls[]"=w943:refnum<vi>[])  [unwired: 2 in, 2 out]
                n647 = for {
                  tunnel: w943 -> [w957] mode=indexing
                  tunnel: [w956] -> w941 mode=indexing
                  n648 = property class="Ctl"(reference=w957) -> ("Label.Text"=w956:string)  [unwired: 1 in, 2 out]
                }
                n649 = property on="X-Axis" class="Ring (strict)"("Strings []"=w941) -> ()  [unwired: 2 in, 2 out]
                n650 = property on="Control Temperature" class="Ring (strict)"("Strings []"=w941) -> ()  [unwired: 2 in, 2 out]
                n651 = property on="X-Axis" class="Ring (strict)"("Strings []"=w941) -> ()  [unwired: 2 in, 2 out]
                n652 = property on="X-Axis" class="Ring (strict)"("Strings []"=w941) -> ()  [unwired: 2 in, 2 out]
                n653 = property on="Temperature 2" class="Ring (strict)"("Strings []"=w941) -> ()  [unwired: 2 in, 2 out]
                n654 = property on="Temperature 3" class="Ring (strict)"("Strings []"=w941) -> ()  [unwired: 2 in, 2 out]
                n655 = property on="Temperature 4" class="Ring (strict)"("Strings []"=w941) -> ()  [unwired: 2 in, 2 out]
                n656 = property on="Temperature 5" class="Ring (strict)"("Strings []"=w941) -> ()  [unwired: 2 in, 2 out]
                n657 = property on="Temperature 6" class="Ring (strict)"("Strings []"=w941) -> ()  [unwired: 2 in, 2 out]
                n658 = property on="Temperature 1" class="Ring (strict)"("Strings []"=w941) -> ()  [unwired: 2 in, 2 out]
                n659 = property on="Main Sample Temperature" class="Ring (strict)"("Strings []"=w941) -> ()  [unwired: 2 in, 2 out]
              }
            }
          }
          frame #7 {
            # "Readout Equipment"
            n660 = stacked-sequence {
              seq-local: [_ w986 _ _ _ _ _ _ _ _ _ _ _ _ _ _ _ _ _ _] -> [_ _ w1002 _ _ _ _ _ _ _ _ _ _ _ _ _ _ _ _ _]
              seq-local: [_ _ w1001 _ _ _ _ _ _ _ _ _ _ _ _ _ _ _ _ _] -> [_ _ _ w1018 _ _ _ _ _ _ _ _ _ _ _ _ _ _ _ _]
              seq-local: [w961 _ _ _ _ _ _ _ _ _ _ _ _ _ _ _ _ _ _ _] -> [_ w985 _ _ _ _ _ _ _ _ _ _ _ _ _ _ _ _ _ _]
              seq-local: [_ _ _ w1017 _ _ _ _ _ _ _ _ _ _ _ _ _ _ _ _] -> [_ _ _ _ w1038 _ _ _ _ _ _ _ _ _ _ _ _ _ _ _]
              seq-local: [_ _ _ _ _ _ _ _ _ _ _ _ w1193 _ _ _ _ _ _ _] -> [_ _ _ _ _ _ _ _ _ _ _ _ _ w1207 _ _ _ _ _ w1275]
              seq-local: [_ _ _ _ _ _ _ _ _ w1161 _ _ _ _ _ _ _ _ _ _] -> [_ _ _ _ _ _ _ _ _ _ w1171 _ _ _ _ _ _ _ _ _]
              seq-local: [_ _ _ _ w1037 _ _ _ _ _ _ _ _ _ _ _ _ _ _ _] -> [_ _ _ _ _ w1073 _ _ _ _ _ _ _ _ _ _ _ _ _ _]
              seq-local: [_ _ _ _ _ _ _ _ _ _ _ w1184 _ _ _ _ _ _ _ _] -> [_ _ _ _ _ _ _ _ _ _ _ _ w1194 _ _ _ _ _ _ _]
              seq-local: [_ _ _ _ _ _ _ _ _ _ _ _ _ w1206 _ _ _ _ _ _] -> [_ _ _ _ _ _ _ _ _ _ _ _ _ _ w1219 _ _ _ _ _]
              seq-local: [_ _ _ _ _ _ _ _ _ _ _ _ _ _ _ _ _ w1254 _ _] -> [_ _ _ _ _ _ _ _ _ _ _ _ _ _ _ _ _ _ w1269 _]
              seq-local: [_ _ _ _ _ w1072 _ _ _ _ _ _ _ _ _ _ _ _ _ _] -> [_ _ _ _ _ _ w1088 _ _ _ _ _ _ _ _ _ _ _ _ _]
              seq-local: [_ _ _ _ _ _ w1087 _ _ _ _ _ _ _ _ _ _ _ _ _] -> [_ _ _ _ _ _ _ w1104 _ _ _ _ _ _ _ _ _ _ _ _]
              seq-local: [_ _ _ _ _ _ _ w1103 _ _ _ _ _ _ _ _ _ _ _ _] -> [_ _ _ _ _ _ _ _ w1121 _ _ _ _ _ _ _ _ _ _ _]
              seq-local: [_ _ _ _ _ _ _ _ _ _ w1170 _ _ _ _ _ _ _ _ _] -> [_ _ _ _ _ _ _ _ _ _ _ w1183 _ _ _ _ _ _ _ _]
              seq-local: [_ _ _ _ _ _ _ _ _ _ _ _ _ _ _ _ w1240 _ _ _] -> [_ _ _ _ _ _ _ _ _ _ _ _ _ _ _ _ _ w1253 _ _]
              seq-local: [_ _ _ _ _ _ _ _ w1120 _ _ _ _ _ _ _ _ _ _ _] -> [_ _ _ _ _ _ _ _ _ w1159 _ _ _ _ _ _ _ _ _ _]
              seq-local: [_ _ _ _ _ _ _ _ _ _ _ _ _ _ w1218 _ _ _ _ _] -> [_ _ _ _ _ _ _ _ _ _ _ _ _ _ _ _ w1239 _ _ _]
              tunnel: w958 -> [w962 _ _ _ _ _ _ _ _ _ _ _ _ _ _ _ _ _ _ _]
              tunnel: [_ _ _ _ _ _ _ _ _ _ _ _ _ _ _ _ _ _ w1270 _] -> w959
              frame #0 {
                # "Lakeshore Readout"
                n661 = global read "Instrument_Setup.vi" "T-control"() -> (w960:string)
                n662 = case shown="\"LS372\", Default" w960 {
                  tunnel: w962 -> [w967 w972 w980 w981]
                  tunnel: [w963 w971 w979 w982] -> w961
                  frame "LS372", Default {
                    n663 = global read "Instrument_Setup.vi" "LS 350"() -> (w965:bool)
                    n664 = global read "Instrument_Setup.vi" "LS 370"() -> (w966:bool)
                    n665 = Or(x=w966, y=w965) -> (x .or. y?=w964:bool)
                    n666 = case shown="True" w964 {
                      tunnel: [w968 w969] -> w963
                      tunnel: w967 -> [w968 w970]
                      frame False {
                      }
                      frame True {
                        n667 = call "Write_LS_Data_without_LS372.vi"("In"=w970) -> ("Out"=w969:T37)
                      }
                    }
                  }
                  frame "LS370" {
                    n668 = global read "Instrument_Setup.vi" "LS 372"() -> (w975:bool)
                    n669 = global read "Instrument_Setup.vi" "LS 350"() -> (w974:bool)
                    n670 = Or(x=w975, y=w974) -> (x .or. y?=w973:bool)
                    n671 = case shown="True" w973 {
                      tunnel: [w976 w977] -> w971
                      tunnel: w972 -> [w976 w978]
                      frame False {
                      }
                      frame True {
                        n672 = call "Write_LS_Data_without_LS370.vi"("In"=w978) -> ("Out"=w977:T37)
                      }
                    }
                  }
                  frame "Insert-control" {
                    n673 = call "Write_LS_Data.vi"("In"=w980) -> ("Out"=w979:T37)
                  }
                  frame "PPMS" {
                    n674 = call "Write_LS_Data.vi"("In"=w981) -> ("Out"=w982:T37)
                  }
                }
              }
              frame #1 {
                # "SR830-1"
                n675 = global read "Instrument_Setup.vi" "Lock In #1"() -> (w984:bool)
                n676 = case shown="True" w984 {
                  tunnel: [FALSE w988] -> w983
                  frame False {
                  }
                  frame True {
                    n677 = global read "Instrument_Setup.vi" "Choose Lock-In #1"() -> (w990:u16)
                    n678 = Equal?(x=w990, y=0) -> (x = y?=w988:bool)
                  }
                }
                n679 = case shown="True" w983 {
                  tunnel: [w991 w994] -> w986
                  tunnel: w985 -> [w991 w992]
                  frame False {
                  }
                  frame True {
                    n680 = global read "Data_Display_global.vi" "SR830-1"() -> (w997:T29)
                    n681 = local read "SR830-1"() -> (w998:T29)
                    n682 = call-poly "Open_Queue.vi"() -> ("queue out"=w996:refnum<queue>)  [unwired: 10 in, 1 out]
                    n683 = call-poly "Manage_Monitor.vi"("Lockin # (in)"=1, "System Monitor Variables (in)"=w992, "Global Status (in)"=w997, "Command (in)"=w998, "queue (in)"=w996) -> ("System Monitor Variables (out)"=w994:T37, "Monitor (out)"=w995:T29)  [unwired: 1 in]
                    n684 = local write "SR830-1"(w995) -> ()
                  }
                }
              }
              frame #2 {
                # "SR830-2"
                n685 = global read "Instrument_Setup.vi" "Lock In #2"() -> (w1000:bool)
                n686 = case shown="True" w1000 {
                  tunnel: [FALSE w1004] -> w999
                  frame False {
                  }
                  frame True {
                    n687 = global read "Instrument_Setup.vi" "Choose Lock-In #2"() -> (w1006:u16)
                    n688 = Equal?(x=w1006, y=0) -> (x = y?=w1004:bool)
                  }
                }
                n689 = case shown="True" w999 {
                  tunnel: w1002 -> [w1007 w1010]
                  tunnel: [w1007 w1009] -> w1001
                  frame False {
                  }
                  frame True {
                    n690 = global read "Data_Display_global.vi" "SR830-2"() -> (w1013:T29)
                    n691 = local read "SR830-2"() -> (w1014:T29)
                    n692 = call-poly "Open_Queue.vi"() -> ("queue out"=w1012:refnum<queue>)  [unwired: 10 in, 1 out]
                    n693 = call-poly "Manage_Monitor.vi"("Lockin # (in)"=2, "System Monitor Variables (in)"=w1010, "Global Status (in)"=w1013, "Command (in)"=w1014, "queue (in)"=w1012) -> ("System Monitor Variables (out)"=w1009:T37, "Monitor (out)"=w1011:T29)  [unwired: 1 in]
                    n694 = local write "SR830-2"(w1011) -> ()
                  }
                }
              }
              frame #3 {
                # "SR830-3"
                n695 = global read "Instrument_Setup.vi" "Lock In #3"() -> (w1016:bool)
                n696 = case shown="True" w1016 {
                  tunnel: [FALSE w1020] -> w1015
                  frame False {
                  }
                  frame True {
                    n697 = global read "Instrument_Setup.vi" "Choose Lock-In #3"() -> (w1022:u16)
                    n698 = Equal?(x=w1022, y=0) -> (x = y?=w1020:bool)
                  }
                }
                n699 = case shown="True" w1015 {
                  tunnel: w1018 -> [w1023 w1026]
                  tunnel: [w1023 w1024] -> w1017
                  frame False {
                  }
                  frame True {
                    n700 = global read "Data_Display_global.vi" "SR830-3"() -> (w1029:T29)
                    n701 = call-poly "Open_Queue.vi"() -> ("queue out"=w1028:refnum<queue>)  [unwired: 10 in, 1 out]
                    n702 = local read "SR830-3"() -> (w1030:T29)
                    n703 = call-poly "Manage_Monitor.vi"("Lockin # (in)"=3, "System Monitor Variables (in)"=w1026, "Global Status (in)"=w1029, "Command (in)"=w1030, "queue (in)"=w1028) -> ("System Monitor Variables (out)"=w1024:T37, "Monitor (out)"=w1027:T29)  [unwired: 1 in]
                    n704 = local write "SR830-3"(w1027) -> ()
                  }
                }
              }
              frame #4 {
                # "PE7265"
                n705 = global read "Instrument_Setup.vi" "Lock In #2"() -> (w1034:bool)
                n706 = case shown="True" w1034 {
                  tunnel: [FALSE w1046] -> w1033
                  frame False {
                  }
                  frame True {
                    n707 = global read "Instrument_Setup.vi" "Choose Lock-In #2"() -> (w1048:u16)
                    n708 = Equal?(x=w1048, y=1) -> (x = y?=w1046:bool)
                  }
                }
                n709 = global read "Instrument_Setup.vi" "Lock In #3"() -> (w1032:bool)
                n710 = global read "Instrument_Setup.vi" "Lock In #1"() -> (w1036:bool)
                n711 = case shown="True" w1036 {
                  tunnel: [FALSE w1050] -> w1035
                  frame False {
                  }
                  frame True {
                    n712 = global read "Instrument_Setup.vi" "Choose Lock-In #1"() -> (w1052:u16)
                    n713 = Equal?(x=w1052, y=1) -> (x = y?=w1050:bool)
                  }
                }
                n714 = case shown="True" w1032 {
                  tunnel: [FALSE w1042] -> w1031
                  frame False {
                  }
                  frame True {
                    n715 = global read "Instrument_Setup.vi" "Choose Lock-In #3"() -> (w1044:u16)
                    n716 = Equal?(x=w1044, y=1) -> (x = y?=w1042:bool)
                  }
                }
                n717 = Or(x=w1035, y=w1033) -> (x .or. y?=w1040:bool)
                n718 = Or(x=w1040, y=w1031) -> (x .or. y?=w1039:bool)
                n719 = case shown="True" w1039 {
                  tunnel: w1038 -> [w1053 w1061]
                  tunnel: [w1053 w1060] -> w1037
                  frame False {
                  }
                  frame True {
                    n720 = global read "Instrument_Setup.vi" "Choose Lock-In #3"() -> (w1056:u16)
                    n721 = Equal?(x=w1056, y=1) -> (x = y?=w1054:bool)
                    n722 = case shown="False" w1054 {
                      tunnel: [w1067 3] -> w1062
                      frame False {
                        n723 = global read "Instrument_Setup.vi" "Choose Lock-In #1"() -> (w1066:u16)
                        n724 = Equal?(x=w1066, y=1) -> (x = y?=w1064:bool)
                        n725 = case shown="True" w1064 {
                          tunnel: [2 1] -> w1067
                          frame False {
                          }
                          frame True {
                          }
                        }
                      }
                      frame True {
                      }
                    }
                    n726 = global read "Data_Display_global.vi" "PE7265-Cluster"() -> (w1058:T27)
                    n727 = local read "PE7265-Cluster"() -> (w1059:T27)
                    n728 = call "PE7265_Open_Queue.vi"() -> ("queue out"=w1063:refnum<queue>)  [unwired: 10 in, 1 out]
                    n729 = call "PE7265_Manage_Monitor.vi"("Lockin# (in)"=w1062, "System Monitor Variables (in)"=w1061, "Global-Status (in)"=w1058, "Command (in)"=w1059, "queue (in)"=w1063) -> ("System Monitor Variables (out)"=w1060:T37, "Monitor (out)"=w1057:T27)  [unwired: 1 in]
                    n730 = local write "PE7265-Cluster"(w1057) -> ()
                  }
                }
              }
              frame #5 {
                # "LIA7230"
                n731 = global read "Instrument_Setup.vi" "Lock In #1"() -> (w1074:bool)
                n732 = case shown="True" w1074 {
                  tunnel: [FALSE w1084] -> w1071
                  frame False {
                  }
                  frame True {
                    n733 = global read "Instrument_Setup.vi" "Choose Lock-In #1"() -> (w1086:u16)
                    n734 = Equal?(x=w1086, y=2) -> (x = y?=w1084:bool)
                  }
                }
                n735 = case shown="True" w1071 {
                  tunnel: w1073 -> [w1075 w1079]
                  tunnel: [w1075 w1076] -> w1072
                  frame False {
                  }
                  frame True {
                    n736 = global read "Data_Display_global.vi" "LIA7230-Cluster"() -> (w1080:T10)
                    n737 = local read "LIA7230-1"() -> (w1078:T10)
                    n738 = call "LIA7230_Open_Queue.vi"() -> ("queue out"=w1082:refnum<queue>)  [unwired: 4 in, 1 out]
                    n739 = call "LIA7230_Manage_Monitor.vi"("Lock -In # (in)"=1, "System Monitor Variables (in)"=w1079, "Command- (in)"=w1078, "Global Status (in)"=w1080, "queue (in)"=w1082) -> ("Monitor (out)"=w1077:T10, "System Monitor Variables (out)"=w1076:T37)  [unwired: 1 in]
                    n740 = local write "LIA7230-1"(w1077) -> ()
                  }
                }
              }
              frame #6 {
                # "LIA 7230"
                n741 = global read "Instrument_Setup.vi" "Lock In #2"() -> (w1090:bool)
                n742 = case shown="True" w1090 {
                  tunnel: [FALSE w1100] -> w1089
                  frame False {
                  }
                  frame True {
                    n743 = global read "Instrument_Setup.vi" "Choose Lock-In #2"() -> (w1102:u16)
                    n744 = Equal?(x=w1102, y=2) -> (x = y?=w1100:bool)
                  }
                }
                n745 = case shown="True" w1089 {
                  tunnel: w1088 -> [w1091 w1096]
                  tunnel: [w1091 w1093] -> w1087
                  frame False {
                  }
                  frame True {
                    n746 = global read "Data_Display_global.vi" "LIA7230-Cluster-2"() -> (w1094:T10)
                    n747 = local read "LIA7230-2"() -> (w1095:T10)
                    n748 = call "LIA7230-2_Open_Queue.vi"() -> ("queue out"=w1098:refnum<queue>)  [unwired: 4 in, 1 out]
                    n749 = call "LIA7230_Manage_Monitor.vi"("Lock -In # (in)"=2, "System Monitor Variables (in)"=w1096, "Command- (in)"=w1095, "Global Status (in)"=w1094, "queue (in)"=w1098) -> ("Monitor (out)"=w1092:T10, "System Monitor Variables (out)"=w1093:T37)  [unwired: 1 in]
                    n750 = local write "LIA7230-2"(w1092) -> ()
                  }
                }
              }
              frame #7 {
                # "LIA7230"
                n751 = global read "Instrument_Setup.vi" "Lock In #3"() -> (w1106:bool)
                n752 = case shown="True" w1106 {
                  tunnel: [FALSE w1116] -> w1105
                  frame False {
                  }
                  frame True {
                    n753 = global read "Instrument_Setup.vi" "Choose Lock-In #3"() -> (w1118:u16)
                    n754 = Equal?(x=w1118, y=2) -> (x = y?=w1116:bool)
                  }
                }
                n755 = case shown="True" w1105 {
                  tunnel: w1104 -> [w1107 w1112]
                  tunnel: [w1107 w1109] -> w1103
                  frame False {
                  }
                  frame True {
                    n756 = global read "Data_Display_global.vi" "LIA7230-Cluster-3"() -> (w1111:T10)
                    n757 = local read "LIA7230-3"() -> (w1110:T10)
                    n758 = call "LIA7230-3_Open_Queue.vi"() -> ("queue out"=w1114:refnum<queue>)  [unwired: 4 in, 1 out]
                    n759 = call "LIA7230_Manage_Monitor.vi"("Lock -In # (in)"=3, "System Monitor Variables (in)"=w1112, "Command- (in)"=w1110, "Global Status (in)"=w1111, "queue (in)"=w1114) -> ("Monitor (out)"=w1108:T10, "System Monitor Variables (out)"=w1109:T37)  [unwired: 1 in]
                    n760 = local write "LIA7230-3"(w1108) -> ()
                  }
                }
              }
              frame #8 {
                # "zurich_lock_in"
                n761 = global read "Instrument_Setup.vi" "Lock In #2"() -> (w1125:bool)
                n762 = case shown="True" w1125 {
                  tunnel: [FALSE w1152] -> w1124
                  frame False {
                  }
                  frame True {
                    n763 = global read "Instrument_Setup.vi" "Choose Lock-In #2"() -> (w1154:u16)
                    n764 = Equal?(x=w1154, y=3) -> (x = y?=w1152:bool)
                  }
                }
                n765 = global read "Instrument_Setup.vi" "Lock In #3"() -> (w1123:bool)
                n766 = global read "Instrument_Setup.vi" "Lock In #1"() -> (w1127:bool)
                n767 = case shown="True" w1127 {
                  tunnel: [FALSE w1156] -> w1126
                  frame False {
                  }
                  frame True {
                    n768 = global read "Instrument_Setup.vi" "Choose Lock-In #1"() -> (w1158:u16)
                    n769 = Equal?(x=w1158, y=3) -> (x = y?=w1156:bool)
                  }
                }
                n770 = case shown="True" w1123 {
                  tunnel: [FALSE w1148] -> w1122
                  frame False {
                  }
                  frame True {
                    n771 = global read "Instrument_Setup.vi" "Choose Lock-In #3"() -> (w1150:u16)
                    n772 = Equal?(x=w1150, y=3) -> (x = y?=w1148:bool)
                  }
                }
                n773 = Or(x=w1126, y=w1124) -> (x .or. y?=w1128:bool)
                n774 = Or(x=w1128, y=w1122) -> (x .or. y?=w1119:bool)
                n775 = case shown="True" w1119 {
                  tunnel: w1121 -> [w1129 w1134]
                  tunnel: [w1129 w1133] -> w1120
                  frame False {
                  }
                  frame True {
                    n776 = global read "Instrument_Setup.vi" "Choose Lock-In #3"() -> (w1139:u16)
                    n777 = global read "Data_Display_global.vi" "Zurich-Lock-In Monitor"() -> (w1135:T4)
                    n778 = Equal?(x=w1139, y=3) -> (x = y?=w1137:bool)
                    n779 = case shown="False" w1137 {
                      tunnel: [w1143 3] -> w1132
                      frame False {
                        n780 = global read "Instrument_Setup.vi" "Choose Lock-In #1"() -> (w1142:u16)
                        n781 = Equal?(x=w1142, y=3) -> (x = y?=w1140:bool)
                        n782 = case shown="True" w1140 {
                          tunnel: [2 1] -> w1143
                          frame False {
                          }
                          frame True {
                          }
                        }
                      }
                      frame True {
                      }
                    }
                    n783 = local read "Zurich-Lock-In Monitor"() -> (w1131:T4)
                    n784 = call "zurich_lock_in_Open_Queue_1.vi"() -> ("queue out"=w1136:refnum<queue>)  [unwired: 10 in, 1 out]
                    n785 = call "zurich_lock_in_Manage_Monitor.vi"("Lockin # (in)"=w1132, "System Monitor Variables (in)"=w1134, "Command (in)"=w1131, "Global Status (in)"=w1135, "queue (in)"=w1136) -> ("Monitor (out)"=w1130:T4, "System Monitor Variables (out)"=w1133:T37)  [unwired: 1 in]
                    n786 = local write "Zurich-Lock-In Monitor"(w1130) -> ()
                  }
                }
              }
              frame #9 {
                # "K6221"
                n787 = global read "Instrument_Setup.vi" "Keithley 6221"() -> (w1160:bool)
                n788 = case shown="True" w1160 {
                  tunnel: [w1162 w1165] -> w1161
                  tunnel: w1159 -> [w1162 w1163]
                  frame False {
                  }
                  frame True {
                    n789 = global read "Data_Display_global.vi" "K6221 Cluster"() -> (w1167:T28)
                    n790 = call "K6221_Open_Queue.vi"() -> ("queue out"=w1168:refnum<queue>)  [unwired: 10 in, 1 out]
                    n791 = local read "K6221"() -> (w1166:T28)
                    n792 = call-poly "Manage_Monitor.vi"("System Monitor Variables (in)"=w1163, "Command (in)"=w1166, "Global Status (in)"=w1167, "queue (in)"=w1168) -> ("System Monitor Variables (out)"=w1165:T37, "Monitor (out)"=w1164:T28)  [unwired: 2 in]
                    n793 = local write "K6221"(w1164) -> ()
                  }
                }
              }
              frame #10 {
                # "K2182A"
                n794 = global read "Instrument_Setup.vi" "Keithley 2182A"() -> (w1169:bool)
                n795 = case shown="True" w1169 {
                  tunnel: w1171 -> [w1172 w1174]
                  tunnel: [w1172 w1173] -> w1170
                  frame False {
                  }
                  frame True {
                    n796 = global read "Data_Display_global.vi" "K2182A Cluster"() -> (w1181:T7)
                    n797 = local read "K2182A"() -> (w1180:T7)
                    n798 = call "K2182A_Split_Cluster.vi"("K2182A Cluster"=w1180) -> ("K2182A Control"=w1177:T53)  [unwired: 1 out]
                    n799 = call "K2182A_Split_Cluster.vi"("K2182A Cluster"=w1181) -> ("K2182A Status"=w1178:T54)  [unwired: 1 out]
                    n800 = call "K2182A_Open_Queue.vi"() -> ("queue out"=w1179:refnum<queue>)  [unwired: 10 in, 1 out]
                    n801 = call "K2182A_Queue_Commands.vi"("K2182A Control"=w1177, "Queue in"=w1179) -> ("New Status"=w1176:T53)  [unwired: 1 in]
                    n802 = call "K2182A_Merge_Cluster.vi"("K2182A Control"=w1176, "AMI_Status"=w1178) -> ("K2182A Cluster"=w1175:T7)
                    n803 = local write "K2182A"(w1175) -> ()
                    n804 = call "K2182A_Set_Monitor_Values.vi"("System Monitor Variables (in)"=w1174) -> ("System Monitor Variables (out)"=w1173:T37)  [unwired: 4 in]
                  }
                }
              }
              frame #11 {
                # "AVS"
                n805 = global read "Instrument_Setup.vi" "Picowatt AVS47"() -> (w1182:bool)
                n806 = case shown="True" w1182 {
                  tunnel: [w1185 w1191] -> w1184
                  tunnel: w1183 -> [w1185 w1186]
                  frame False {
                  }
                  frame True {
                    n807 = local read "Picowatt AVS47/TS530 Cluster"() -> (w1188:T26)
                    n808 = global read "Data_Display_global.vi" "Picowatt AVS47/TS530 Cluster"() -> (w1187:T26)
                    n809 = call "PicowattAVS47_Open_Queue.vi"() -> ("queue out"=w1190:refnum<queue>)  [unwired: 10 in, 1 out]
                    n810 = call "PicowattAVS47_Manage_Monitor.vi"("System Monitor Variables (in)"=w1186, "Global Status (in)"=w1187, "Command (in)"=w1188, "Queue (in)"=w1190) -> ("System Monitor Variables (out)"=w1191:T37, "Monitor (out)"=w1189:T26)
                    n811 = local write "Picowatt AVS47/TS530 Cluster"(w1189) -> ()
                  }
                }
              }
              frame #12 {
                # "AH2500"
                n812 = global read "Instrument_Setup.vi" "AH 2500"() -> (w1192:bool)
                n813 = case shown="True" w1192 {
                  tunnel: w1194 -> [w1195 w1197]
                  tunnel: [w1195 w1196] -> w1193
                  frame False {
                  }
                  frame True {
                    n814 = local read "AH2500 Monitor"() -> (w1203:T18)
                    n815 = global read "Data_Display_global.vi" "AH2500-Cluster"() -> (w1201:T18)
                    n816 = call "AH2500_Open_Queue.vi"() -> ("queue out"=w1204:refnum<queue>)  [unwired: 10 in, 1 out]
                    n817 = call "AH2500_Splitt_Cluster.vi"("AH2500-Cluster"=w1203) -> ("AH2500-Control"=w1202:T55)  [unwired: 1 out]
                    n818 = call "AH2500_Splitt_Cluster.vi"("AH2500-Cluster"=w1201) -> ("AH2500-Status"=w1199:T56)  [unwired: 1 out]
                    n819 = call "AH2500_Queue_Commands.vi"("AH2500-Control"=w1202, "AH2500 Queue"=w1204) -> ("New Status"=w1200:T55)  [unwired: 1 in]
                    n820 = call "AH2500_Merge_Cluster.vi"("AH2500-Control"=w1200, "AH2500-Status"=w1199) -> ("AH2500-Cluster"=w1198:T18)
                    n821 = local write "AH2500 Monitor"(w1198) -> ()
                    n822 = call "AH2500_Set_Monitor_Values.vi"("System Monitor Variables (in)"=w1197) -> ("System Monitor Variables (out)"=w1196:T37)  [unwired: 4 in]
                  }
                }
              }
              frame #13 {
                # "AH2700"
                n823 = global read "Instrument_Setup.vi" "AH 2700"() -> (w1205:bool)
                n824 = case shown="True" w1205 {
                  tunnel: w1207 -> [w1208 w1210]
                  tunnel: [w1208 w1209] -> w1206
                  frame False {
                  }
                  frame True {
                    n825 = local read "AH 2700 Monitor"() -> (w1216:T17)
                    n826 = global read "Data_Display_global.vi" "AH 2700-Cluster"() -> (w1213:T17)
                    n827 = call "AH2700_Splitt_Cluster.vi"("AH 2700-Cluster"=w1216) -> ("AH2700-Control"=w1215:T57)  [unwired: 1 in, 1 out]
                    n828 = call "AH2700_Splitt_Cluster.vi"("AH 2700-Cluster"=w1213) -> ("AH 2700-Status"=w1212:T58)  [unwired: 1 in, 1 out]
                    n829 = call "AH2700_Open_Queue.vi"() -> ("queue out"=w1217:refnum<queue>)  [unwired: 10 in, 1 out]
                    n830 = call "AH2700_Queue_Commands.vi"("AH2700-Control"=w1215, "AH2700 Queue"=w1217) -> ("New Status"=w1214:T57)  [unwired: 1 in]
                    n831 = call "AH2700_Merge_Cluster.vi"("AH 2700-Status"=w1212, "AH2700-Control"=w1214) -> ("AH 2700-Cluster"=w1211:T17)
                    n832 = local write "AH 2700 Monitor"(w1211) -> ()
                    n833 = call "AH2700_Set_Monitor_Values.vi"("System Monitor Variables (in)"=w1210) -> ("System Monitor Variables (out)"=w1209:T37)  [unwired: 4 in]
                  }
                }
              }
              frame #14 {
                # "SIM921"
                n834 = global read "Instrument_Setup.vi" "SIM921"() -> (w1220:bool)
                n835 = case shown="False" w1220 {
                  tunnel: w1219 -> [w1221 w1223]
                  tunnel: [w1221 w1222] -> w1218
                  frame False {
                  }
                  frame True {
                    n836 = local read "SIM921"() -> (w1230:T1)
                    n837 = global read "Data_Display_global.vi" "SIM921"() -> (w1227:T1)
                    n838 = call "SIM921_splitt_cluster.vi"("SIM921"=w1230) -> ("SIM921-Control"=w1228:T59)  [unwired: 2 in, 1 out]
                    n839 = call "SIM921_Open_Queue.vi"() -> ("queue out"=w1229:refnum<queue>)  [unwired: 10 in, 1 out]
                    n840 = call "SIM921_splitt_cluster.vi"("SIM921"=w1227) -> ("SIM921-Status"=w1225:T60)  [unwired: 2 in, 1 out]
                    n841 = call "SIM921_Queue_Commands.vi"("SIM921-Control"=w1228, "SIM Queue"=w1229) -> ("SIM921-Control new status"=w1226:T59)  [unwired: 1 in]
                    n842 = call "SIM921_merge_cluster.vi"("SIM921-Status"=w1225, "SIM921-Control"=w1226) -> ("SIM921"=w1224:T1)  [unwired: 2 in]
                    n843 = local write "SIM921"(w1224) -> ()
                    n844 = call "SIM921_Set_values.vi"("System Monitor Variables (in)"=w1223) -> ("System Monitor Variables (out)"=w1222:T37)
                  }
                }
              }
              frame #15 {
                # "VCM Monitor"
                n845 = global read "Instrument_Setup.vi" "VCM"() -> (w1231:bool)
                n846 = case shown="True" w1231 {
                  frame False {
                  }
                  frame True {
                    n847 = global read "Data_Display_global.vi" "VCM Monitor"() -> (w1234:T22)
                    n848 = local read "VCM Monitor"() -> (w1238:T22)
                    n849 = call "VCM_Split_Cluster.vi"("VCM Monitor"=w1234) -> ("VCM Status"=w1233:T61)  [unwired: 1 out]
                    n850 = call "VCM_Open_Queue.vi"() -> ("queue out"=w1237:refnum<queue>)  [unwired: 10 in, 1 out]
                    n851 = call "VCM_Split_Cluster.vi"("VCM Monitor"=w1238) -> ("VCM Control"=w1236:T62)  [unwired: 1 out]
                    n852 = call "VCM_Queue_Commands.vi"("VCM Control"=w1236, "VCM Queue"=w1237) -> ("New Status"=w1235:T62)  [unwired: 1 in]
                    n853 = call "VCM_Merge_Cluster.vi"("VCM Control"=w1235, "VCM Status"=w1233) -> ("VCM Monitor"=w1232:T22)
                    n854 = local write "VCM Monitor"(w1232) -> ()
                  }
                }
              }
              frame #16 {
                n855 = global read "Instrument_Setup.vi" "Torque \nMeasurem."() -> (w1241:bool)
                n856 = case shown="True" w1241 {
                  tunnel: w1239 -> [w1242 w1244]
                  tunnel: [w1242 w1243] -> w1240
                  frame False {
                  }
                  frame True {
                    n857 = local read "TMC-Control"() -> (w1250:T6)
                    n858 = global read "Data_Display_global.vi" "TMC-Cluster"() -> (w1251:T6)
                    n859 = call "TMC_Split_Cluster.vi"("TMC Cluster"=w1251) -> ("TMC-Status"=w1247:T63)  [unwired: 2 in, 1 out]
                    n860 = call "TMC_Split_Cluster.vi"("TMC Cluster"=w1250) -> ("TMC-Control"=w1248:T64)  [unwired: 2 in, 1 out]
                    n861 = call "TMC_Open_Queue.vi"() -> ("queue out"=w1249:refnum<queue>)  [unwired: 10 in, 1 out]
                    n862 = call "TMC_Queue_Commands.vi"("TMC-Control"=w1248, "TMC Queue"=w1249) -> ("TMC-Control new"=w1246:T64)  [unwired: 1 in]
                    n863 = call "TMC_Merge_Cluster.vi"("TMC-Status"=w1247, "TMC-Control"=w1246) -> ("TMC Cluster"=w1245:T6)  [unwired: 2 in]
                    n864 = local write "TMC-Control"(w1245) -> ()
                    n865 = call "TMC_Set_Monitor_Values.vi"("System Monitor Variables (in)"=w1244) -> ("System Monitor Variables (out)"=w1243:T37)  [unwired: 4 in]
                  }
                }
              }
              frame #17 {
                # "20 T Dewar Heater Auto/Manual"
                n866 = global read "Instrument_Setup.vi" "Instrument"() -> (w1252:string)
                n867 = case shown="\"20T\"" w1252 {
                  tunnel: [w1255 w1258] -> w1254
                  tunnel: w1253 -> [w1255 w1256]
                  frame "PPMS", Default {
                  }
                  frame "20T" {
                    n868 = global read "Data_Display_global.vi" "20T-Dewar-Cluster"() -> (w1264:T30)
                    n869 = local read "20T-Dewar-Cluster"() -> (w1263:T30)
                    n870 = call-poly "Open_Queue.vi"() -> ("queue out"=w1268:refnum<queue>)  [unwired: 10 in, 1 out]
                    n871 = call-poly "Manage_Monitor.vi"("System Monitor Variables (in)"=w1256, "Command (in)"=w1263, "Global Status (in)"=w1264, "queue (in)"=w1268) -> ("System Monitor Variables (out)"=w1258:T37, "Monitor (out)"=w1257:T30)  [unwired: 2 in]
                    n872 = Unbundle By Name(w1257) -> ("Dewar heater manual"=w1261:bool)
                    n873 = local write "20T-Dewar-Cluster"(w1257) -> ()
                    n874 = global write "Data_Display_global.vi" "20T-Dewar-Cluster"(w1257) -> ()
                    n875 = Select(t=cluster{u32, u32}[] [{16711680, 0}] ("Colors [4]"), s=w1261, f=cluster{u32, u32}[] [{65280, 0}] ("Colors [4]")) -> (s? t:f=w1265:cluster{u32, u32}[])
                    n876 = Select(t="Manual", s=w1261, f="Auto") -> (s? t:f=w1259:string)
                    n877 = property on="Change D-Heater Status" class="Bool (strict)"("Colors [4]"=w1265, "BoolText.Text"=w1259) -> ()  [unwired: 2 in, 2 out]
                  }
                }
              }
              frame #18 {
                # "Add \"Nada\""
                n878 = Unbundle By Name(w1269) -> ("Nada"=w1273:dbl[])
                n879 = Build Array (concatenate)(w1273, nan) -> (w1271:dbl[])
                n880 = Bundle By Name(cluster=w1269, "Nada"=w1271) -> (w1270:T37)
              }
              frame #19 {
                # "Set Control Temperature and Main Sample Temperature"
                n881 = call "Select_Value.vi"("Numerisch"="Control Temperature", "System Monitor Variables"=w1275) -> ()  [unwired: 1 in, 3 out]
                n882 = call "Select_Value.vi"("Numerisch"="Main Sample Temperature", "System Monitor Variables"=w1275) -> ("String"=w1274:string)  [unwired: 1 in, 2 out]
                n883 = global write "Data_Display_global.vi" "Main Sample Therometer"(w1274) -> ()
              }
            }
          }
          frame #8 {
            # "To do! Set AMI Values!!!"
            # "Magnet Control"
            n884 = global read "Instrument_Setup.vi" "Instrument"() -> (w1280:string)
            n885 = case shown="\"20T\"" w1280 {
              tunnel: w1279 -> [w1282 w1316 w1335 w1337 w1371 w1393 w1416]
              tunnel: [w1281 w1315 w1335 w1336 w1370 w1392 w1417] -> w1278
              frame "Sweet 16" {
                n886 = stacked-sequence {
                  tunnel: w1282 -> [w1286 _ _]
                  tunnel: [w1285 _ _] -> w1281
                  frame #0 {
                    n887 = global read "Data_Display_global.vi" "16 T Cluster"() -> (w1283:T34)
                    n888 = local read "16 T Magnet control"() -> (w1290:T34)
                    n889 = call-poly "Open_Queue.vi"() -> ("queue out"=w1291:refnum<queue>)  [unwired: 10 in, 1 out]
                    n890 = call-poly "Split_Cluster.vi"("16 T Magnet control"=w1290) -> ("16 T Magnet control"=w1289:T65)  [unwired: 1 out]
                    n891 = call-poly "Split_Cluster.vi"("16 T Magnet control"=w1283) -> ("16 T Status"=w1287:T66)  [unwired: 1 out]
                    n892 = call-poly "Queue_Commands.vi"("16 T Magnet control"=w1289, "16T Queue"=w1291) -> ("New Status"=w1288:T65)  [unwired: 1 in]
                    n893 = call "16T_Set_Monitor_Values.vi"("System Monitor Variables (in)"=w1286) -> ("System Monitor Variables (out)"=w1285:T37)  [unwired: 4 in]
                    n894 = call-poly "Merge_Cluster.vi"("16 T Control"=w1288, "16 T Status"=w1287) -> ("16 T Magnet control"=w1284:T34)
                    n895 = local write "16 T Magnet control"(w1284) -> ()
                  }
                  frame #1 {
                    n896 = global read "Data_Display_global.vi" "16 T Cluster"() -> (w1302:T34)
                    n897 = global read "Data_Display_global.vi" "Switch heater waiting"() -> (w1299:bool)
                    n898 = global read "Data_Display_global.vi" "Switch Button Text"() -> (w1301:string)
                    n899 = Unbundle By Name(w1302) -> ("Switch"=w1303:bool)
                    n900 = Select(t=cluster{u32, u32}[] [{16711680, 0}] ("Colors [4]"), s=w1303, f=cluster{u32, u32}[] [{11974326, 0}] ("Colors [4]")) -> (s? t:f=w1292:cluster{u32, u32}[])
                    n901 = Select(t=w1301, s=w1299, f="Switch") -> (s? t:f=w1295:string)
                    n902 = Select(t=1, s=w1299, f=0) -> (s? t:f=w1296:i32)
                    n903 = property on="Switch Heater" class="Bool (strict)"("BoolText.Text"=w1295, "DisabledEnum"=w1296, "Colors [4]"=w1292) -> ()  [unwired: 2 in, 2 out]
                  }
                  frame #2 {
                    w1312 = cluster{u32, u32}[] [{11974326, 0}] ("Colors [4]")
                    w1311 = cluster{u32, u32}[] [{16711680, 0}] ("Colors [4]")
                    n904 = global read "Data_Display_global.vi" "16 T Cluster"() -> (w1314:T34)
                    n905 = Unbundle By Name(w1314) -> ("Clamped"=w1313:bool, "Hold"=w1306:bool, "Set"=w1305:bool, "Zero"=w1304:bool)
                    n906 = Select(t=w1311, s=w1313, f=w1312) -> (s? t:f=w1307:cluster{u32, u32}[])
                    n907 = Select(t=w1311, s=w1306, f=w1312) -> (s? t:f=w1308:cluster{u32, u32}[])
                    n908 = Select(t=w1311, s=w1305, f=w1312) -> (s? t:f=w1309:cluster{u32, u32}[])
                    n909 = Select(t=w1311, s=w1304, f=w1312) -> (s? t:f=w1310:cluster{u32, u32}[])
                    n910 = property on="Clamp" class="Bool (strict)"("Colors [4]"=w1307) -> ()  [unwired: 2 in, 2 out]
                    n911 = property on="Go to Hold" class="Bool (strict)"("Colors [4]"=w1308) -> ()  [unwired: 2 in, 2 out]
                    n912 = property on="Go to set" class="Bool (strict)"("Colors [4]"=w1309) -> ()  [unwired: 2 in, 2 out]
                    n913 = property on="Go to Zero" class="Bool (strict)"("Colors [4]"=w1310) -> ()  [unwired: 2 in, 2 out]
                  }
                }
              }
              frame "Mischer" {
                n914 = stacked-sequence {
                  tunnel: w1316 -> [w1318 _]
                  tunnel: [w1317 _] -> w1315
                  frame #0 {
                    n915 = local read "5 T Cluster"() -> (w1320:T24)
                    n916 = global read "Data_Display_global.vi" "5 T Cluster"() -> (w1325:T24)
                    n917 = call "5T_Split_Cluster.vi"("5 T Cluster"=w1320) -> ("5T Control"=w1319:T67)  [unwired: 1 out]
                    n918 = call "5T_open_queue.vi"() -> ("queue out"=w1322:refnum<queue>)  [unwired: 10 in, 1 out]
                    n919 = call "5T_Split_Cluster.vi"("5 T Cluster"=w1325) -> ("5 T Status"=w1324:T68)  [unwired: 1 out]
                    n920 = call "5T_Queue_Commands.vi"("5T Control"=w1319, "5T Queue"=w1322) -> ("New Status"=w1321:T67)  [unwired: 1 in]
                    n921 = call "5T_Merge_Cluster.vi"("5T Control"=w1321, "5 T Status"=w1324) -> ("5 T Cluster"=w1323:T24)
                    n922 = local write "5 T Cluster"(w1323) -> ()
                    n923 = call "5T_Set_Monitor_Values.vi"("System Monitor Variables (in)"=w1318) -> ("System Monitor Variables (out)"=w1317:T37)  [unwired: 4 in]
                  }
                  frame #1 {
                    w1330 = cluster{u32, u32}[] [{11974326, 0}] ("Colors [4]")
                    w1329 = cluster{u32, u32}[] [{16711680, 0}] ("Colors [4]")
                    n924 = global read "Data_Display_global.vi" "5 T Cluster"() -> (w1334:T24)
                    n925 = Unbundle By Name(w1334) -> ("Hold"=w1333:bool, "Set"=w1332:bool, "Zero"=w1331:bool)
                    n926 = Select(t=w1329, s=w1333, f=w1330) -> (s? t:f=w1328:cluster{u32, u32}[])
                    n927 = Select(t=w1329, s=w1332, f=w1330) -> (s? t:f=w1327:cluster{u32, u32}[])
                    n928 = Select(t=w1329, s=w1331, f=w1330) -> (s? t:f=w1326:cluster{u32, u32}[])
                    n929 = property on="Go to Hold" class="Bool (strict)"("Colors [4]"=w1328) -> ()  [unwired: 2 in, 2 out]
                    n930 = property on="Go to set" class="Bool (strict)"("Colors [4]"=w1327) -> ()  [unwired: 2 in, 2 out]
                    n931 = property on="Go to Zero" class="Bool (strict)"("Colors [4]"=w1326) -> ()  [unwired: 2 in, 2 out]
                  }
                }
              }
              frame "None", Default {
              }
              frame "Berta" {
                n932 = stacked-sequence {
                  tunnel: w1337 -> [w1339 _ _]
                  tunnel: [w1338 _ _] -> w1336
                  frame #0 {
                    n933 = local read "15T-Cluster"() -> (w1345:T16)
                    n934 = global read "Data_Display_global.vi" "15T-Cluster"() -> (w1346:T16)
                    n935 = call "15T_Open_Queue.vi"() -> ("queue out"=w1344:refnum<queue>)  [unwired: 10 in, 1 out]
                    n936 = call "15T_Splitt_Queue.vi"("15T-Cluster"=w1345) -> ("15T-Control"=w1343:T69)  [unwired: 1 in, 1 out]
                    n937 = call "15T_Splitt_Queue.vi"("15T-Cluster"=w1346) -> ("15T-Status"=w1342:T70)  [unwired: 1 in, 1 out]
                    n938 = call "15T_Queue_Commands.vi"("15T-Control"=w1343, "15T Queue"=w1344) -> ("New Status"=w1341:T69)  [unwired: 1 in]
                    n939 = call "15T_Merge_Cluster.vi"("15T-Status"=w1342, "15T-Control"=w1341) -> ("15T-Cluster"=w1340:T16)  [unwired: 1 in]
                    n940 = local write "15T-Cluster"(w1340) -> ()
                    n941 = call "5T_Set_Monitor_Values.vi"("System Monitor Variables (in)"=w1339) -> ("System Monitor Variables (out)"=w1338:T37)  [unwired: 4 in]
                  }
                  frame #1 {
                    n942 = global read "Data_Display_global.vi" "15T-Cluster"() -> (w1358:T16)
                    n943 = global read "Data_Display_global.vi" "Switch heater waiting"() -> (w1350:bool)
                    n944 = global read "Data_Display_global.vi" "Switch Button Text"() -> (w1354:string)
                    n945 = Unbundle By Name(w1358) -> ("Switch"=w1356:bool)
                    n946 = Select(t=cluster{u32, u32}[] [{16711680, 0}] ("Colors [4]"), s=w1356, f=cluster{u32, u32}[] [{11974326, 0}] ("Colors [4]")) -> (s? t:f=w1348:cluster{u32, u32}[])
                    n947 = Select(t=w1354, s=w1350, f="Switch") -> (s? t:f=w1349:string)
                    n948 = Select(t=1, s=w1350, f=0) -> (s? t:f=w1347:i32)
                    n949 = property on="Switch Heater" class="Bool (strict)"("BoolText.Text"=w1349, "DisabledEnum"=w1347, "Colors [4]"=w1348) -> ()  [unwired: 2 in, 2 out]
                  }
                  frame #2 {
                    w1368 = cluster{u32, u32}[] [{11974326, 0}] ("Colors [4]")
                    w1367 = cluster{u32, u32}[] [{16711680, 0}] ("Colors [4]")
                    n950 = global read "Data_Display_global.vi" "15T-Cluster"() -> (w1369:T16)
                    n951 = Unbundle By Name(w1369) -> ("Set"=w1365:bool, "Zero"=w1363:bool, "Hold"=w1361:bool, "Clamped"=w1359:bool)
                    n952 = Select(t=w1367, s=w1365, f=w1368) -> (s? t:f=w1366:cluster{u32, u32}[])
                    n953 = Select(t=w1367, s=w1363, f=w1368) -> (s? t:f=w1364:cluster{u32, u32}[])
                    n954 = Select(t=w1367, s=w1361, f=w1368) -> (s? t:f=w1362:cluster{u32, u32}[])
                    n955 = Select(t=w1367, s=w1359, f=w1368) -> (s? t:f=w1360:cluster{u32, u32}[])
                    n956 = property on="Go to Set" class="Bool (strict)"("Colors [4]"=w1366) -> ()  [unwired: 2 in, 2 out]
                    n957 = property on="Go to zero" class="Bool (strict)"("Colors [4]"=w1364) -> ()  [unwired: 2 in, 2 out]
                    n958 = property on="Go to Hold" class="Bool (strict)"("Colors [4]"=w1362) -> ()  [unwired: 2 in, 2 out]
                    n959 = property on="Clamp" class="Bool (strict)"("Colors [4]"=w1360) -> ()  [unwired: 2 in, 2 out]
                  }
                }
              }
              frame "AMI" {
                n960 = stacked-sequence {
                  tunnel: w1371 -> [_ w1383]
                  tunnel: [_ w1382] -> w1370
                  frame #0 {
                    # "Set switch Button Text"
                    n961 = global read "Data_Display_global.vi" "Switch heater waiting"() -> (w1375:bool)
                    n962 = case shown="False" w1375 {
                      tunnel: ["Switch" w1381] -> w1374
                      tunnel: [0 1] -> w1373
                      tunnel: [16777215 255] -> w1372
                      frame False {
                        # "IF not waiting for SH"
                      }
                      frame True {
                        n963 = global read "Data_Display_global.vi" "Switch Button Text"() -> (w1381:string)
                      }
                    }
                    n964 = property on="Switch Heater" class="Bool (strict)"("BoolText.Text"=w1374, "DisabledEnum"=w1373, "BoolText.BGColor"=w1372, "BoolText.TextColor"=w1372) -> ()  [unwired: 2 in, 2 out]
                  }
                  frame #1 {
                    # "Set AMI Field"
                    n965 = global read "Data_Display_global.vi" "AMI_Cluster"() -> (w1387:T20)
                    n966 = local read "AMI_Cluster"() -> (w1391:T20)
                    n967 = local read "AMI Status"() -> (w1389:T19)
                    n968 = call "AMI_Open_Queue.vi"() -> ("queue out"=w1390:refnum<queue>)  [unwired: 10 in, 1 out]
                    n969 = call "AMI_Split_Cluster.vi"("AMI_Cluster"=w1387) -> ("AMI_Status"=w1386:T71)  [unwired: 1 out]
                    n970 = call "AMI_Split_Cluster.vi"("AMI_Cluster"=w1391) -> ("AMI_Control"=w1388:T19)  [unwired: 1 out]
                    n971 = call "AMI_Queue_Commands.vi"("AMI_Control"=w1388, "Last Status"=w1389, "Queue in"=w1390) -> ("New Status"=w1384:T19)
                    "AMI Status" <- w1384
                    n972 = call "AMI_Merge_Cluster.vi"("AMI_Control"=w1384, "AMI_Status"=w1386) -> ("AMI_Cluster"=w1385:T20)
                    n973 = local write "AMI_Cluster"(w1385) -> ()
                    n974 = call "AMI_Set_Monitor_Values.vi"("System Monitor Variables (in)"=w1383) -> ("System Monitor Variables (out)"=w1382:T37)  [unwired: 4 in]
                  }
                }
              }
              frame "20T" {
                n975 = stacked-sequence {
                  tunnel: w1393 -> [_ w1408]
                  tunnel: [_ w1407] -> w1392
                  frame #0 {
                    n976 = global read "Data_Display_global.vi" "Switch heater waiting"() -> (w1398:bool)
                    n977 = case shown="True" w1398 {
                      tunnel: [0 1] -> w1396
                      tunnel: [0 255] -> w1394
                      tunnel: ["Switch" w1404] -> w1395
                      tunnel: [T40."Disabled and Grayed Out" ("Disabled") T40."Disabled and Grayed Out" ("Disabled")] -> w1397
                      frame False {
                      }
                      frame True {
                        n978 = global read "Data_Display_global.vi" "Switch Button Text"() -> (w1404:string)
                      }
                    }
                    n979 = property on="16 T Magnet control" class="Clust (strict)"("DisabledEnum"=w1397) -> ()  [unwired: 2 in, 2 out]
                    n980 = property on="Switch Heater" class="Bool (strict)"("BoolText.Text"=w1395, "DisabledEnum"=w1396, "Label.BG Color"=w1394, "Label.FG Color"=w1394) -> ()  [unwired: 2 in, 2 out]
                  }
                  frame #1 {
                    n981 = global read "Data_Display_global.vi" "20 T Magnet control"() -> (w1410:T3)
                    n982 = local read "20 T Magnet control"() -> (w1413:T3)
                    n983 = call-poly "Split_Cluster.vi"("20 T Cluster"=w1410) -> ("20 T Status"=w1411:T72)  [unwired: 1 out]
                    n984 = call-poly "Split_Cluster.vi"("20 T Cluster"=w1413) -> ("20 T Control"=w1412:T52)  [unwired: 1 out]
                    n985 = call-poly "Open_Queue.vi"() -> ("queue out"=w1414:refnum<queue>)  [unwired: 10 in, 1 out]
                    n986 = call-poly "Queue_Commands.vi"("20T Control (in)"=w1412, "20T Queue"=w1414) -> ("20T Control (out)"=w1415:T52)  [unwired: 1 in]
                    n987 = call-poly "Merge_Cluster.vi"("20T Control"=w1415, "20T Status"=w1411) -> ("20 T Magnet control"=w1409:T3)
                    n988 = call "20T_Set_Monitor_Values.vi"("System Monitor Variables (in)"=w1408) -> ("System Monitor Variables (out)"=w1407:T37)  [unwired: 4 in]
                    n989 = local write "20 T Magnet control"(w1409) -> ()
                  }
                }
              }
              frame "PPMS" {
                n990 = stacked-sequence {
                  tunnel: [w1419 _] -> w1417
                  tunnel: w1416 -> [w1418 _]
                  frame #0 {
                    n991 = local read "P9/P14-Magnet-Cluster"() -> (w1426:T9)
                    n992 = global read "Data_Display_global.vi" "P9/P14-Magnet-Cluster"() -> (w1424:T9)
                    n993 = call "P9P14_Splitt_Cluster.vi"("P9/P14-Magnet-Cluster"=w1424) -> ("P9/P14-Magnet Status"=w1422:T73, "P9/P14-Magnet-Control"=w1423:T74)  [unwired: 1 in]
                    n994 = call "P9P14_Splitt_Cluster.vi"("P9/P14-Magnet-Cluster"=w1426) -> ("P9/P14-Magnet-Control"=w1425:T74)  [unwired: 1 in, 1 out]
                    n995 = call "P9P14T_Open_Queue.vi"() -> ("queue out"=w1427:refnum<queue>)  [unwired: 10 in, 1 out]
                    n996 = call "P9P14T_Queue_Commands.vi"("P9/P14-Magnet-Control"=w1425, "P9/P14-Magnet-Control old status"=w1423, "16T Queue"=w1427) -> ("P9/P14-Magnet-Control new status"=w1421:T74)
                    n997 = call "P9P14T_Merge_Cluster.vi"("P9/P14-Magnet-Control"=w1421, "P9/P14-Magnet Status"=w1422) -> ("P9/P14-Magnet-Cluster"=w1420:T9)
                    n998 = local write "P9/P14-Magnet-Cluster"(w1420) -> ()
                    n999 = call "P9P14T_set_Monitor_values.vi"("System Monitor Variables (in)"=w1418) -> ("System Monitor Variables (out)"=w1419:T37)
                  }
                  frame #1 {
                    n1000 = global read "Data_Display_global.vi" "P9/P14-Magnet-Cluster"() -> (w1435:T9)
                    n1001 = Unbundle By Name(w1435) -> ("Magnet Status"=w1429:i32)
                    n1002 = case shown="1" w1429 {
                      tunnel: [FALSE TRUE] -> w1433
                      frame 0, Default {
                      }
                      frame 1 {
                      }
                    }
                    n1003 = case shown="3" w1429 {
                      tunnel: [FALSE TRUE] -> w1428
                      frame 0, Default {
                      }
                      frame 3 {
                      }
                    }
                    n1004 = Select(t="Persitent", s=w1433, f="Non-Persitent") -> (s? t:f=w1434:string)
                    n1005 = Select(t=cluster{u32, u32}[] [{16711680, 0}] ("Colors [4]"), s=w1433, f=cluster{u32, u32}[] [{11974326, 0}] ("Colors [4]")) -> (s? t:f=w1438:cluster{u32, u32}[])
                    n1006 = Select(t=1, s=w1428, f=0) -> (s? t:f=w1430:i32)
                    n1007 = property on="Set Persitant/non-pers" class="Bool (strict)"("BoolText.Text"=w1434, "Colors [4]"=w1438, "DisabledEnum"=w1430) -> ()  [unwired: 2 in, 2 out]
                  }
                }
              }
            }
          }
          frame #9 {
            n1008 = case shown="True" TRUE {
              tunnel: w1447 -> [w1448 w1450]
              tunnel: [w1448 w1452] -> w1446
              frame False {
              }
              frame True {
                # "Angle"
                # "Keithely"
                # "Heater & Needle Valve monitor"
                n1009 = Unbundle By Name(w1450) -> ("Time"=w1464:timestamp[])
                n1010 = Get Date/Time In Seconds() -> (seconds since 1Jan1904=w1462:timestamp)
                n1011 = Build Array (concatenate)(w1464, w1462) -> (w1463:timestamp[])
                n1012 = Bundle By Name(cluster=w1450, "Time"=w1463) -> (w1449:T37)
                n1013 = Unbundle By Name(w1449) -> ("K2440_Res"=w1460:dbl[], "K2440_Current"=w1461:dbl[])
                n1014 = global read "Data_Display_global.vi" "Resistance"() -> (w1457:dbl)
                n1015 = global read "Data_Display_global.vi" "Current"() -> (w1456:dbl)
                n1016 = global read "Data_Display_global.vi" "Angle"() -> (w1455:dbl)
                n1017 = Build Array (concatenate)(w1460, w1457) -> (w1459:dbl[])
                n1018 = Build Array (concatenate)(w1461, w1456) -> (w1458:dbl[])
                n1019 = Bundle By Name(cluster=w1449, "K2440_Res"=w1459, "K2440_Current"=w1458) -> (w1453:T37)
                n1020 = Unbundle By Name(w1453) -> ("Angle"=w1454:dbl[])
                n1021 = Build Array (concatenate)(w1454, w1455) -> (w1451:dbl[])
                n1022 = Bundle By Name(cluster=w1453, "Angle"=w1451) -> (w1452:T37)
              }
            }
          }
          frame #10 {
            # "Insert Setup"
            n1023 = global read "Instrument_Setup.vi" "Insert"() -> (w1471:string)
            n1024 = case shown="\"VTI\"" w1471 {
              tunnel: [w1472 TRUE w1496 w1498 w1536] -> w1470
              tunnel: [w1475 w1485 w1497 w1515 w1533] -> w1469
              tunnel: [w1472 w1484 w1496 TRUE w1536] -> w1468
              tunnel: [TRUE w1484 w1496 w1498 w1536] -> w1467
              tunnel: w1466 -> [w1473 w1486 w1497 w1499 w1534]
              tunnel: [w1472 w1484 w1496 w1498 TRUE] -> w1465
              frame "VTI" {
                w1479 = T75 {"Set VTI SP"=FALSE, "Change NV Status"=FALSE, "Set NV Setpoint"=FALSE, "Change Heater Status"=FALSE, "Set Heater Setpoint"=FALSE, "Setpoint (K)"=0.0, "Rate (K/min)"=0.0, "Setpoint Heater"=0.0, "Setpoint NV"=0.0, "Change Auto PID"=FALSE, "Stop Sweep"=FALSE}  # Inital Status
                w1472 = FALSE
                n1025 = global read "Data_Display_global.vi" "VTI"() -> (w1483:T35)
                n1026 = local read "VTI"() -> (w1482:T35)
                n1027 = call "VTI_Open_Queue.vi"() -> ("queue out"=w1481:refnum<queue>)  [unwired: 10 in, 1 out]
                n1028 = call "VTI_Split_Cluster.vi"("VTI"=w1482) -> ("VTI Control"=w1480:T75)  [unwired: 1 out]
                n1029 = call "VTI_Split_Cluster.vi"("VTI"=w1483) -> ("VTI Status"=w1476:T76)  [unwired: 1 out]
                n1030 = call "VTI_Queue_Commands.vi"("VTI Control"=w1480, "Last status"=w1479, "20TVTI Queue"=w1481) -> ("New Status"=w1478:T75)
                n1031 = call "VTI_Merge_Cluster.vi"("VTI Control"=w1478, "VTI Status"=w1476) -> ("VTI"=w1477:T35)
                n1032 = call "VTI_Set_Monitor_Values.vi"("VTI Status"=w1476, "System Monitor Variables (in)"=w1473) -> ("System Monitor Variables (out)"=w1475:T37)  [unwired: 3 in]
                n1033 = local write "VTI"(w1477) -> ()
              }
              frame "20TVTI" {
                w1487 = T77 {"Set VTI SP"=FALSE, "Change NV Status"=FALSE, "Set NV Setpoint"=FALSE, "Change Heater Status"=FALSE, "Set D-Heater Setpoint"=FALSE, "Set Heater Setpoint"=FALSE, "Change D-Heater Status"=FALSE, "Set Sweep Type"=FALSE, "Setpoint (K)"=0.0, "Rate (K/min)"=0.0, "Setpoint Heater"=0.0, "Setpoint D-Heater"=0.0, "Setpoint NV"=0.0}  # 20TVTI INIT
                w1484 = FALSE
                n1034 = local read "20TVTI"() -> (w1494:T32)
                n1035 = global read "Data_Display_global.vi" "20TVTI"() -> (w1493:T32)
                n1036 = call-poly "Open_Queue.vi"() -> ("queue out"=w1488:refnum<queue>)  [unwired: 10 in, 1 out]
                n1037 = call-poly "Split_Cluster.vi"("VTI Cluster"=w1494) -> ("VTI Control"=w1491:T77)  [unwired: 1 out]
                n1038 = call-poly "Queue_Commands.vi"("VTI Control"=w1491, "Last Status"=w1487, "20TVTI Queue"=w1488) -> ("New Status"=w1490:T77)
                n1039 = call-poly "Split_Cluster.vi"("VTI Cluster"=w1493) -> ("VTI Status"=w1489:T78)  [unwired: 1 out]
                n1040 = call-poly "Merge_Cluster.vi"("VTI Control"=w1490, "VTI Status"=w1489) -> ("VTI Cluster"=w1492:T32)
                n1041 = call "20TVTI_Set_Monitor_Values.vi"("VTI Status"=w1489, "System Monitor Variables (in)"=w1486) -> ("System Monitor Variables (out)"=w1485:T37)  [unwired: 3 in]
                n1042 = local write "20TVTI"(w1492) -> ()
              }
              frame "None", Default {
                w1496 = FALSE
              }
              frame "JT" {
                w1501 = T12 {"Disable Heater"=FALSE, "Activate Tsweep"=FALSE, "Update Lakeshores"=FALSE, "Setpoint - Manual"=0.23, "Rate (K/min)"=3.0, "Sorb Power (mW)"=0.0, "Still Power (mW)"=0.0, "Sorb Heater"=FALSE, "Still Heater"=FALSE, "Set Temperature Sweep Main"=FALSE}  # JT Last Status
                w1498 = FALSE
                n1043 = local read "Readout\nMonitor (s)"() -> (w1512:dbl)
                n1044 = local read "JT-Cluster"() -> (w1517:T36)
                n1045 = call-poly "Split_Cluster.vi"("Cluster"=w1517) -> ("Status"=w1511:T79, "Control"=w1502:T12)
                n1046 = call-poly "Open_Queue.vi"() -> ("queue out"=w1518:refnum<queue>)  [unwired: 10 in, 1 out]
                n1047 = call-poly "Queue_Commands.vi"("Control"=w1502, "Last Status"=w1501, "Queue"=w1518) -> ("New Status"=w1516:T12)
                n1048 = call-poly "Set_Monitor_Values.vi"("Plot-Control"=w1511, "X-Axis (S)"=60.0, "Measurement Time (s)"=w1512, "System Monitor Variables (in)"=w1499) -> ("Cluster"=w1513:T79, "System Monitor Variables (out)"=w1515:T37)
                n1049 = call-poly "Merge_Cluster.vi"("JT Control"=w1516, "JT Status"=w1513) -> ("JT Cluster"=w1510:T36)
                n1050 = local write "Emergency Stop JT"("JT Emergency") -> ()
                n1051 = Unbundle By Name(w1510) -> ("Box Temp"=w1504:dbl)
                n1052 = Greater?(x=w1504, y=30) -> (0:w1508:bool)
                n1053 = Greater?(x=w1504, y=35) -> (0:w1503:bool)
                n1054 = case shown="True" w1508 {
                  tunnel: [w1526 6946805] -> w1506
                  tunnel: w1504 -> [w1525 _]
                  tunnel: 50 -> [w1524 _]
                  frame True {
                    n1055 = Greater?(x=w1525, y=w1524) -> (0:w1523:bool)
                    n1056 = case shown="True" w1523 {
                      tunnel: [13567526 15159808] -> w1526
                      frame True {
                      }
                      frame False {
                      }
                    }
                  }
                  frame False, Default {
                  }
                }
                n1057 = case shown="True" w1503 {
                  frame False {
                  }
                  frame True {
                    n1058 = call <vilib>:"Error Cluster From Error Code.vi"("error message (\"\")"="Error Code 999: Critical warning: Box Temperature is over 35 C", "error code (0)"=999) -> ("error out"=w1521:errorcluster)  [unwired: 7 in]
                    n1059 = call "Error_handler.vi"("error constant"=w1521) -> ()
                  }
                }
                n1060 = local write "JT-Cluster"(w1510) -> ()
                n1061 = property on="Box Temp" class="DigNum (strict)"("NumText.BG Color"=w1506, "NumText.FG Color"=w1506, "NumText.BGColor"=w1506) -> ()  [unwired: 2 in, 2 out]
              }
              frame "Kelvinox" {
                w1536 = FALSE
                n1062 = local read "Kelvinox-Cluster"() -> (w1531:T2)
                n1063 = global read "Data_Display_global.vi" "Kelvinox-Cluster"() -> (w1532:T80)
                n1064 = call "Kelvinox_Open_Queue.vi"() -> ("queue out"=w1539:refnum<queue>)  [unwired: 10 in, 1 out]
                n1065 = call "Kelvinox_Split_Cluster.vi"("Kelvinox-Cluster"=w1531) -> ("Kelvinox-Control"=w1538:T81)  [unwired: 1 out]
                n1066 = call "Kelvinox_Queue_Commands.vi"("Control"=w1538, "Queue"=w1539) -> ("New Status"=w1537:T81)  [unwired: 1 in]
                n1067 = call "Kelvinox_Merge_Cluster.vi"("Kelvinox-Control"=w1537, "Kelvinox-Status"=w1532) -> ("Kelvinox-Cluster"=w1530:T2)
                n1068 = local write "Kelvinox-Cluster"(w1530) -> ()
                n1069 = call "Kelvinox_Set_Monitor_Values.vi"("System Monitor Variables (in)"=w1534) -> ("System Monitor Variables (out)"=w1533:T37)  [unwired: 4 in]
              }
            }
            n1070 = property on="Kelvinox-Cluster" class="Clust (strict)"("Visible"=w1465) -> ()  [unwired: 2 in, 2 out]
            n1071 = property on="VTI" class="Clust (strict)"("Visible"=w1467) -> ()  [unwired: 2 in, 2 out]
            n1072 = property on="JT-Cluster" class="Clust (strict)"("Visible"=w1468) -> ()  [unwired: 2 in, 2 out]
            n1073 = property on="20TVTI" class="Clust (strict)"("Visible"=w1470) -> ()  [unwired: 2 in, 2 out]
          }
          frame #11 {
            # "Temperatur conrol"
            n1074 = global read "Instrument_Setup.vi" "T-control"() -> (w1546:string)
            n1075 = case shown="\"ITC503\"" w1546 {
              tunnel: w1545 -> [w1553 w1574 w1584 w1597 w1606 w1628]
              tunnel: [w1553 w1573 w1583 w1596 w1605 w1628] -> w1544
              tunnel: [FALSE TRUE FALSE FALSE FALSE w1627] -> w1543
              tunnel: [w1547 w1569 w1582 TRUE FALSE w1627] -> w1542
              tunnel: [FALSE FALSE TRUE FALSE FALSE w1627] -> w1541
              tunnel: [w1547 w1569 w1582 FALSE TRUE w1627] -> w1540
              frame "Insert-control", Default {
                w1547 = FALSE
                n1076 = global read "Instrument_Setup.vi" "LS 370"() -> (w1551:bool)
                n1077 = global read "Instrument_Setup.vi" "Insert"() -> (w1549:string)
                n1078 = global read "Instrument_Setup.vi" "LS 372"() -> (w1550:bool)
                n1079 = case shown="\"None\", Default" w1549 {
                  tunnel: w1551 -> [_ w1554]
                  frame "JT" {
                  }
                  frame "None", Default {
                    n1080 = case shown="True" w1554 {
                      frame False {
                      }
                      frame True {
                        n1081 = global read "Data_Display_global.vi" "Lakeshore 370 read only"() -> (w1557:T14)
                        n1082 = local read "LS370_Readout-Monitor"() -> (w1560:T14)
                        n1083 = call "LS370_read_only_Open_Queue.vi"() -> ("queue out"=w1561:refnum<queue>)  [unwired: 10 in, 1 out]
                        n1084 = call "LS370_read_only_Splitt_cluster.vi"("Lakeshore 370 read only"=w1560) -> ("Lakeshore 370 read only Control"=w1559:T82)  [unwired: 1 out]
                        n1085 = call "LS370_read_only_Splitt_cluster.vi"("Lakeshore 370 read only"=w1557) -> ("Lakeshore 370 read only Status"=w1556:T83)  [unwired: 1 out]
                        n1086 = call "LS370_read_only_Queue_Commands.vi"("Lakeshore 370 read only Control"=w1559, "Queue"=w1561) -> ("Lakeshore 370 read only Control new Status"=w1558:T82)  [unwired: 1 in]
                        n1087 = call "LS370_read_only_Merge_Cluster.vi"("Lakeshore 370 read only Control"=w1558, "Lakeshore 370 read only Status"=w1556) -> ("Lakeshore 370 read only"=w1555:T14)
                        n1088 = local write "LS370_Readout-Monitor"(w1555) -> ()
                      }
                    }
                  }
                }
                n1089 = case shown="True" w1550 {
                  frame False {
                  }
                  frame True {
                    n1090 = global read "Data_Display_global.vi" "LS372_only_read-Cluster"() -> (w1565:T13)
                    n1091 = local read "LS372_Readout-Monitor"() -> (w1567:T13)
                    n1092 = call "LS372_read_only_Open_Queue.vi"() -> ("queue out"=w1568:refnum<queue>)  [unwired: 10 in, 1 out]
                    n1093 = call "LS372_read_only_Split_Cluster.vi"("LS372_only_read-Cluster"=w1567) -> ("LS372_only_read-Cluster Control"=w1566:T84)  [unwired: 1 out]
                    n1094 = call "LS372_read_only_Split_Cluster.vi"("LS372_only_read-Cluster"=w1565) -> ("LS372_only_read-Cluster Status"=w1564:T85)  [unwired: 1 out]
                    n1095 = call "LS372_read_only_Quwue_Commands.vi"("LS372_only_read-Cluster Control"=w1566, "Queue"=w1568) -> ("LS372_only_read-Cluster Control new Status"=w1563:T84)  [unwired: 1 in]
                    n1096 = call "Ls372_read_only_Merge_Cluster.vi"("LS372_only_read-Cluster Control"=w1563, "LS372_only_read-Cluster Status"=w1564) -> ("LS372_only_read-Cluster"=w1562:T13)
                    n1097 = local write "LS372_Readout-Monitor"(w1562) -> ()
                  }
                }
              }
              frame "LS372" {
                w1569 = FALSE
                n1098 = global read "Data_Display_global.vi" "LS372-Cluster"() -> (w1581:T21)
                n1099 = local read "LS372-Cluster"() -> (w1578:T21)
                n1100 = call "LS372_Split_Cluster.vi"("LS372-Cluster"=w1578) -> ("LS372-Control"=w1577:T41)  [unwired: 1 out]
                n1101 = call "LS372_Open_Queue.vi"() -> ("queue out"=w1579:refnum<queue>)  [unwired: 10 in, 1 out]
                n1102 = call "LS372_Split_Cluster.vi"("LS372-Cluster"=w1581) -> ("LS372-Status"=w1572:T86)  [unwired: 1 out]
                n1103 = call "LS372_Queue_Commands.vi"("LS372-Control"=w1577, "LS372-Last Status"=T41 {"Activate Tsweep"=FALSE, "Setpoint - Manual"=0.0, "Rate (K/min)"=0.0, "Update Lakeshores"=FALSE, "Still Heater"=FALSE, "Still Power (mW)"=0.0, "Manual Heater"=FALSE, "Manual Heater  (mW) "=0.0, "MC Thermometer"=0, "Set Temperature Sweeep main"=FALSE, "Disable Heater"=FALSE} ("LS372-Control"), "Queue"=w1579) -> ("LS372-New Status"=w1576:T41)
                n1104 = call "Ls372_Merge_Cluster.vi"("LS372-Control"=w1576, "LS372-Status"=w1572) -> ("LS372-Cluster"=w1575:T21)
                n1105 = call "LS372_set_Monitor_Values.vi"("LS372-Status"=w1572, "System Monitor Variables (in)"=w1574) -> ("System Monitor Variables (out)"=w1573:T37)  [unwired: 3 in]
                n1106 = local write "LS372-Cluster"(w1575) -> ()
              }
              frame "ITC503" {
                w1582 = FALSE
                n1107 = local read "ITC503-Monitor"() -> (w1590:T11)
                n1108 = global read "Data_Display_global.vi" "ITC503-Monitor"() -> (w1587:T11)
                n1109 = call "ITC503_Split_Cluster.vi"("ITC503-Monitor"=w1590) -> ("ITC503-Control"=w1589:T87)  [unwired: 1 out]
                n1110 = call "ITC503_Split_Cluster.vi"("ITC503-Monitor"=w1587) -> ("ITC503-Status-Monitor"=w1585:T88)  [unwired: 1 out]
                n1111 = call "ITC503_Open_Queue.vi"() -> ("queue out"=w1591:refnum<queue>)  [unwired: 10 in, 1 out]
                n1112 = call "ITC503_Queue_commands.vi"("ITC503-Control"=w1589, "ITC503 Queue"=w1591) -> ("ITC503-Control New Status"=w1588:T87)  [unwired: 1 in]
                n1113 = call "ITC503_Merge_Cluster.vi"("ITC503-Control"=w1588, "ITC503-Status-Monitor"=w1585) -> ("ITC503-Monitor"=w1586:T11)
                n1114 = local write "ITC503-Monitor"(w1586) -> ()
                n1115 = call "ITC503_set_values.vi"("ITC503-Status-Monitor"=w1585, "System Monitor Variables (in)"=w1584) -> ("System Monitor Variables (out)"=w1583:T37)  [unwired: 3 in]
              }
              frame "LS370" {
                w1600 = T12 {"Disable Heater"=FALSE, "Activate Tsweep"=FALSE, "Update Lakeshores"=FALSE, "Setpoint - Manual"=0.23, "Rate (K/min)"=3.0, "Sorb Power (mW)"=0.0, "Still Power (mW)"=0.0, "Sorb Heater"=FALSE, "Still Heater"=FALSE, "Set Temperature Sweep Main"=FALSE}  # LS370 Last Status
                n1116 = local read "LS370-Control"() -> (w1599:T12)
                n1117 = call-poly "Open_Queue.vi"() -> ("queue out"=w1601:refnum<queue>)  [unwired: 10 in, 1 out]
                n1118 = call-poly "Queue_Commands.vi"("Control"=w1599, "Last Status"=w1600, "Queue"=w1601) -> ("New Status"=w1598:T12)
                n1119 = local write "LS370-Control"(w1598) -> ()
                n1120 = call "LS370_set_control_values.vi"("System Monitor Variables (in)"=w1597) -> ("System Monitor Variables (out)"=w1596:T37)
              }
              frame "PPMS" {
                n1121 = stacked-sequence {
                  seq-local: [w1611 _] -> [_ w1619]
                  tunnel: [_ w1619] -> w1604
                  frame #0 {
                    n1122 = local read "P9-P14 T-Cluster"() -> (w1616:T5)
                    n1123 = global read "Data_Display_global.vi" "P9-P14 T-Cluster"() -> (w1614:T5)
                    n1124 = call "P9P14_Temp_Split_Cluster.vi"("P9-P14 T-Cluster"=w1614) -> ("P9-P14 T-Cluster-Status"=w1611:T89)  [unwired: 1 out]
                    n1125 = call "P9P14_Temp_open_queue.vi"() -> ("queue out"=w1617:refnum<queue>)  [unwired: 10 in, 1 out]
                    n1126 = call "P9P14_Temp_Split_Cluster.vi"("P9-P14 T-Cluster"=w1616) -> ("P9-P14 T-Cluster -Control"=w1615:T90)  [unwired: 1 out]
                    n1127 = call "P9P14_Temp_Queue_Commands.vi"("P9-P14 T-Cluster -Control"=w1615, "Queue"=w1617) -> ("P9-P14 T-New Status"=w1613:T90)  [unwired: 1 in]
                    n1128 = call "P9P14_Temp_Merge_Cluster.vi"("P9-P14 T-Cluster -Control"=w1613, "P9-P14 T-Cluster-Status"=w1611) -> ("P9-P14 T-Cluster"=w1612:T5)
                    n1129 = local write "P9-P14 T-Cluster"(w1612) -> ()
                  }
                  frame #1 {
                    n1130 = global read "Instrument_Setup.vi" "LS 370"() -> (w1618:bool)
                    n1131 = case shown="True" w1618 {
                      frame False {
                      }
                      frame True {
                        n1132 = local read "LS370_Readout-Monitor"() -> (w1621:T14)
                        n1133 = global read "Data_Display_global.vi" "Lakeshore 370 read only"() -> (w1620:T14)
                        n1134 = call "LS370_read_only_Open_Queue.vi"() -> ("queue out"=w1626:refnum<queue>)  [unwired: 10 in, 1 out]
                        n1135 = call "LS370_read_only_Splitt_cluster.vi"("Lakeshore 370 read only"=w1621) -> ("Lakeshore 370 read only Control"=w1625:T82)  [unwired: 1 out]
                        n1136 = call "LS370_read_only_Splitt_cluster.vi"("Lakeshore 370 read only"=w1620) -> ("Lakeshore 370 read only Status"=w1623:T83)  [unwired: 1 out]
                        n1137 = call "LS370_read_only_Queue_Commands.vi"("Lakeshore 370 read only Control"=w1625, "Queue"=w1626) -> ("Lakeshore 370 read only Control new Status"=w1624:T82)  [unwired: 1 in]
                        n1138 = call "LS370_read_only_Merge_Cluster.vi"("Lakeshore 370 read only Control"=w1624, "Lakeshore 370 read only Status"=w1623) -> ("Lakeshore 370 read only"=w1622:T14)
                        n1139 = local write "LS370_Readout-Monitor"(w1622) -> ()
                      }
                    }
                  }
                }
                n1140 = call "P9P14_Temp_Set_values.vi"("P9-P14 T-Cluster-Status"=w1604, "System Monitor Variables (in)"=w1606) -> ("System Monitor Variables (out)"=w1605:T37)
              }
              frame "None" {
                w1627 = FALSE
              }
            }
            n1141 = property on="ITC503-Monitor" class="Clust (strict)"("Visible"=w1541) -> ()  [unwired: 2 in, 2 out]
            n1142 = property on="LS372-Cluster" class="Clust (strict)"("Visible"=w1543) -> ()  [unwired: 2 in, 2 out]
            n1143 = property on="LS370-Control" class="Clust (strict)"("Visible"=w1542) -> ()  [unwired: 2 in, 2 out]
            n1144 = property on="P9-P14 T-Cluster" class="Clust (strict)"("Visible"=w1540) -> ()  [unwired: 2 in, 2 out]
          }
          frame #12 {
            # "Write Logfile"
            n1145 = call <vilib>:"Application Directory.vi"() -> ("Application Directory"=w1630:path)
            n1146 = call "Write_Logfile.vi"("path"=w1630, "System Monitor Variables (in)"=w1629) -> ()  [unwired: 1 in]
          }
          frame #13 {
            # "Save and Open Configurations"
            n1147 = case shown="True" "Save" {
              frame False {
              }
              frame True {
                n1148 = call "Save_Monitor_Config.vi"() -> ()  [unwired: 12 in]
              }
            }
            n1149 = case shown="True" "Open" {
              frame False {
              }
              frame True {
                n1150 = call "Open_Monitor_Config.vi"() -> ()  [unwired: 12 in]
              }
            }
          }
          frame #14 {
            # "Stop Monitors and save System Montior Variables to file"
            n1151 = case shown="True" "Stop Monitor" {
              tunnel: [FALSE TRUE] -> w1634
              frame False {
              }
              frame True {
                n1152 = Two Button Dialog(message="Stop Monitors as well?? Choose NO, if measurement is running!", 1:"No!", 2:"Yes!") -> (T button?=w1648:bool)
                n1153 = global write "Data_Display_global.vi" "Stop Monitors"(w1648) -> ()
              }
            }
            n1154 = case shown="True" w1634 {
              tunnel: w1633 -> [_ w1642]
              frame False {
              }
              frame True {
                n1155 = call <vilib>:"Application Directory.vi"() -> ("Application Directory"=w1639:path)
                n1156 = Path To String(path=w1639) -> (string=w1640:string)
                n1157 = Concatenate Strings(w1640, "\\Configurations\\System Monitor.ini") -> (w1638:string)
                n1158 = String To Path(string=w1638) -> (path=w1637:path)
                n1159 = Open/Create/Replace Datalog(5:w1642, 10:4, 11:w1637) -> (0:w1643:errorcluster, 3:w1646:refnum<k1>)  [unwired: 3 in, 1 out]
                n1160 = Write Datalog(4:w1643, 6:w1642, 7:w1646) -> (0:w1644:errorcluster, 3:w1645:refnum<k1>)
                n1161 = Close File(refnum=w1645, error in=w1644) -> ()  [unwired: 2 out]
              }
            }
          }
          frame #15 {
            # "Email to Experiment Responsible, \nif critical error is detected"
            # "Reset Error, if noticed"
            # "Warning Handling"
            n1162 = global read "Data_Display_global.vi" "Error mail has been sent?"() -> (w1656:bool)
            n1163 = global read "Data_Display_global.vi" "Critical Error"() -> (w1654:bool)
            n1164 = local read "Reset Warning"() -> (w1657:bool)
            n1165 = Not(x=w1656) -> (.not. x?=w1653:bool)
            n1166 = And(x=w1654, y=w1653) -> (x .and. y?=w1655:bool)
            n1167 = case shown="True" w1655 {
              frame False {
              }
              frame True {
                n1168 = call "Email_notification.vi"("Email"="E-mail of Experiment resposible") -> ()
              }
            }
            n1169 = case shown="True" w1657 {
              tunnel: w1657 -> [_ w1661]
              frame False {
                n1170 = global read "Data_Display_global.vi" "Error String"() -> (w1659:string)
                n1171 = local write "Warning"(w1659) -> ()
              }
              frame True {
                w1660 = FALSE
                n1172 = Not(x=w1661) -> (.not. x?=w1662:bool)
                n1173 = global write "Data_Display_global.vi" "Error"(w1660) -> ()
                n1174 = global write "Data_Display_global.vi" "Error String"("") -> ()
                n1175 = local write "Reset Warning"(w1662) -> ()
                n1176 = global write "Data_Display_global.vi" "Error mail has been sent?"(w1660) -> ()
                n1177 = global write "Data_Display_global.vi" "Critical Error"(w1660) -> ()
              }
            }
          }
          frame #16 {
            # "Safety Checks for JT/Kelvinox"
            n1178 = global read "Instrument_Setup.vi" "Insert"() -> (w1665:string)
            n1179 = case shown="\"Kelvinox\"" w1665 {
              tunnel: w1664 -> [_ w1669 _]
              frame "None", Default {
              }
              frame "JT" {
                n1180 = global read "Data_Display_global.vi" "Error String"() -> (w1668:string)
                n1181 = call "JT_ueberwachung.vi"("Warning In"=w1668, "System Monitor Variables"=w1669) -> ("Warning-Bool"=w1666:bool, "Warning Out"=w1667:string)  [unwired: 8 in]
                n1182 = global write "Data_Display_global.vi" "Error String"(w1667) -> ()
                n1183 = global write "Data_Display_global.vi" "Error"(w1666) -> ()
              }
              frame "Kelvinox" {
                n1184 = global read "Instrument_Setup.vi" "Knox Safety Checks (temporarily here)"() -> (w1670:bool)
                n1185 = case shown="True" w1670 {
                  frame False {
                  }
                  frame True {
                    n1186 = local read "Kelvinox-Cluster"() -> (w1671:T2)
                    n1187 = Unbundle By Name(w1671) -> ("1K Pot"=w1672:dbl, "P2"=w1676:dbl, "P5"=w1681:dbl)
                    n1188 = Greater?(x=w1672, y=2.5) -> (0:w1673:bool)
                    n1189 = Greater?(x=w1676, y=500.0) -> (0:w1677:bool)
                    n1190 = Greater?(x=w1681, y=250.0) -> (0:w1680:bool)
                    n1191 = case shown="True" w1673 {
                      selector: w1673 -> [_ w1684]
                      tunnel: "Carefull! 1K Pot temperature above 2.5K. Check if the Pot has run empty." -> [_ w1687]
                      frame False {
                      }
                      frame True {
                        n1192 = Bundle By Name(cluster=errorcluster {"status"=FALSE, "code"=0, "source"=""} ("error constant"), "code"=999, "status"=w1684, "source"=w1687) -> (w1686:errorcluster)
                        n1193 = call "Error_handler.vi"("error constant"=w1686) -> ()
                      }
                    }
                    n1194 = case shown="True" w1677 {
                      selector: w1677 -> [_ w1689]
                      tunnel: "Carefull! Forepump out pressure above 500mbar." -> [_ w1692]
                      frame False {
                      }
                      frame True {
                        n1195 = Bundle By Name(cluster=errorcluster {"status"=FALSE, "code"=0, "source"=""} ("error constant"), "code"=999, "status"=w1689, "source"=w1692) -> (w1691:errorcluster)
                        n1196 = call "Error_handler.vi"("error constant"=w1691) -> ()
                      }
                    }
                    n1197 = case shown="True" w1680 {
                      selector: w1680 -> [_ w1694]
                      tunnel: "Carefull! Condenser pressure above 250mbar." -> [_ w1697]
                      frame False {
                      }
                      frame True {
                        n1198 = Bundle By Name(cluster=errorcluster {"status"=FALSE, "code"=0, "source"=""} ("error constant"), "code"=999, "status"=w1694, "source"=w1697) -> (w1696:errorcluster)
                        n1199 = call "Error_handler.vi"("error constant"=w1696) -> ()
                      }
                    }
                  }
                }
              }
            }
          }
          frame #17 {
            n1200 = case shown="True" "Truncate Button 2" {
              tunnel: "Keep every nth" -> [_ w1708]
              tunnel: w1699 -> [w1705 w1707]
              tunnel: [w1705 w1706] -> w1702
              frame False {
              }
              frame True {
                n1201 = call "Delete_every_nth_element.vi"("n"=w1708, "System Monitor Variables"=w1707) -> ("System Monitor Variables 2"=w1706:T37)
              }
            }
            n1202 = case shown="True" "Truncate Button" {
              tunnel: w1702 -> [w1709 w1715]
              tunnel: [w1709 w1716] -> w1700
              frame False {
              }
              frame True {
                n1203 = Unbundle By Name(w1715) -> ("Time"=w1714:timestamp[])
                n1204 = To Double Precision Float(number="Time Stamp") -> (double precision float=w1712:dbl)
                n1205 = To Double Precision Float(number=w1714) -> (double precision float=w1713:dbl[])
                n1206 = Threshold 1D Array(2:w1712, 3:w1713) -> (0:w1710:dbl)  [unwired: 1 in]
                n1207 = call "Truncate_cluster_Monitor.vi"("Length"=w1710, "System Monitor Variables"=w1715) -> ("System Monitor Variables 2"=w1716:T37)
              }
            }
          }
          frame #18 {
            # "Plot Panels"
            n1208 = property on="System Monitor Variables" class="Clust (strict)"() -> ("Controls[]"=w1732:refnum<vi>[])  [unwired: 2 in, 2 out]
            n1209 = local read "Plot 3"() -> (w1724:T31)
            n1210 = local read "Plot 1"() -> (w1726:T31)
            n1211 = local read "Plot 2"() -> (w1725:T31)
            n1212 = control-ref of="Measurement Graph"() -> (w1719:refnum<vi>)
            n1213 = for {
              tunnel: w1732 -> [w1741] mode=indexing
              tunnel: [w1740] -> w1730 mode=indexing
              n1214 = property class="Ctl"(reference=w1741) -> ("Label.Text"=w1740:string)  [unwired: 1 in, 2 out]
            }
            n1215 = control-ref of="Measurement Graph"() -> (w1739:refnum<vi>)
            n1216 = control-ref of="Measurement Graph"() -> (w1720:refnum<vi>)
            n1217 = control-ref of="Plot 2 Y"() -> (w1723:refnum<vi>)
            n1218 = control-ref of="Plot 2 Y"() -> (w1722:refnum<vi>)
            n1219 = control-ref of="Plot 2 Y"() -> (w1721:refnum<vi>)
            n1220 = Build Array(w1726, w1725, w1724) -> (w1729:T31[])
            n1221 = Build Array(w1720, w1739, w1719) -> (w1718:refnum<vi>[])
            n1222 = call "Handle_Plot.vi"("Graph reference"=w1718, "System Monitor Variables (in)"=w1717, "Plot Array (in)"=w1729) -> ("Measurement Graphs"=w1728:T31[])  [unwired: 1 in]
            n1223 = Build Array(w1723, w1722, w1721) -> (w1731:refnum<vi>[])
            n1224 = call "Max_Min_Measurement_Graph.vi"("Graph Reference"=w1718, "Measurement Graphs (in)"=w1728) -> ("Measurement Graphs (out)"=w1727:T31[])
            n1225 = Index Array(array=w1727, index=0) -> (element=w1733:T31)
            n1226 = Index Array(array=w1727, index=2) -> (element=w1735:T31)
            n1227 = Index Array(array=w1727, index=1) -> (element=w1734:T31)
            n1228 = local write "Plot 1"(w1733) -> ()
            n1229 = local write "Plot 3"(w1735) -> ()
            n1230 = local write "Plot 2"(w1734) -> ()
            n1231 = for {
              tunnel: w1718 -> [w1744] mode=indexing
              tunnel: w1729 -> [w1752] mode=indexing
              tunnel: w1731 -> [w1743] mode=indexing
              tunnel: w1730 -> [w1742]
              n1232 = Unbundle By Name(w1752) -> ("Y-Axis Array"=w1746:i16[], "X-Axis"=w1750:i16)
              n1233 = property on="Property Node" class="Ring (strict)"(reference=w1743, "Strings []"=w1742) -> ()  [unwired: 1 in, 2 out]
              n1234 = Array Size(array=w1746) -> (size(s)=w1745:i32)
              n1235 = Equal To 0?(x=w1750) -> (x = 0?=w1751:bool)
              n1236 = Select(t=7.0, s=w1751, f=0.0) -> (s? t:f=w1749:dbl)
              n1237 = property on="Property Node" class="XYGraph (strict)"(reference=w1744, "LegNumRows"=w1745, "XScale.Format"=w1749) -> ()  [unwired: 1 in, 2 out]
            }
          }
        }
      }
    }
  }
